vi "Main_Marvin Remake.vi"() -> ()   [LabVIEW 2017]
uses:
  PCAN_Driver/ControlCAN.llb/DevType.ctl
  PCAN_Driver/ControlCAN.llb/CAN Channel.ctl
  PCAN_Driver/ControlCAN.llb/VCI_INIT_CONFIG.ctl
  PCAN_Driver/ControlCAN.llb/InitFlag.ctl
  PCAN_Driver/ControlCAN.llb/Fliter.ctl
  PCAN_Driver/ControlCAN.llb/Mode.ctl
  <vilib>/Utility/miscctls.llb/LVRowAndColumnTypeDef.ctl
  <vilib>/Utility/sysdir.llb/System Directory Type.ctl
  <vilib>/Utility/config.llb/Read Key (String).vi
  <vilib>/Utility/config.llb/Write Key (String).vi
  <vilib>/Utility/cursorutil.llb/Set Cursor (Icon Pict).vi
  PCAN_Driver/ControlCAN.lvlib
  <vilib>/Utility/config.llb/NI_LVConfig.lvlib
panel:
  out "ADCValOutput Single":dbl
  out "Numeric 3":i32
  out "5.4.0":bool=TRUE
  out "MaxEbaySpeed":u16
  out "AuxiONResult 2":bool
  out "AuxiOFFResult 2":bool
  out "Numeric 2":dbl
  out "UUT SoftwareVer2":string
  out "Numeric":dbl
  out "DSP Board S/N":string
  out "POWER Board S/N":string caption="DRIVER Board S/N"
  out "BurnInSpeed":u16
  out "SpeedCommandSpeed":u16
  out "VenableSpeed":u16
  out "CurrentTest":T1(ring)
  out "TesterVersion":string
  out "ClosePanel":bool=TRUE
  out "UUT SN Report":string
  out "Automation":bool
  out "Test Failed":bool
  out "AuxiOFFResult":bool
  out "AuxiONResult":bool
  out "SensCalResult":bool
  out "VisualInspectionResult":bool
  out "BurnResult":bool
  out "BurnSpeed":bool
  out "BurnTemp":bool
  out "BurnDC":bool
  out "TempControlResult":bool
  out "MotorTempResult":bool
  out "StopTimeResult":bool
  out "SpeedResult":bool=TRUE
  out "VenableDirectionResult":bool
  out "VenableResult":bool
  out "ComTestResult":bool=TRUE
  out "UUT SoftwareVer":string
  out "Next SN":i32
  in  "SetSN":bool
  out "Current SN":i32
  out "Cal":dbl
  out "AO[1]Meas":dbl
  out "FullSpeed2 Speed":dbl
  out "FullSpeed2 Current":dbl
  out "FullSpeed1 Current":dbl
  out "FullSpeed1 Speed":dbl
  out "MaxBurnInTempVal":dbl
  in  "Stop Burn-in":bool
  out "VISA Tester":refnum<visa-resource-name>
  out "UUT":u8
  out "CAN Status":bool
  in  "Channel 2":T2 caption="Channel" items=["Channel 1", "Channel 2"]
  out "Config_CANAT":T8 {"DevType" items=["USB-CAN"=3, "USB-CAN2"=4]; "CanIndex" items=["通道1", "通道2"]; "VCI_INIT_CONFIG"."Fliter" items=["接收所有类型"=3, "只接收标准帧"=4, "只接收扩展帧"=7]; "VCI_INIT_CONFIG"."Mode" items=["正常工作", "自测模式（环回）", "仅侦听模式"]; "VCI_INIT_CONFIG"."InitFlag" items=["使用Flash参数", "使用界面设置参数"]}
  out "Array":u64[][](array[numeric]) format="%016x"
  out "Motor Phase Current RMS":dbl
  out "Ambient Temperature":dbl
  out "Speed error":bool
  out "Commutation err":bool
  out "Under voltage/Over voltage":bool
  out "Derated drive temp":bool
  out "Motor Over temperature":bool
  out "Motor Sensor temp Fauilre":bool
  out "Drive Over temperature":bool
  out "Drive Sensor temp Failure":bool
  out "Ambient Over temp":bool
  out "Ambient Sensor temp":bool
  out "DC Voltage":dbl
  out "DC Current":dbl
  out "Power transistor Heat sink Temp.":dbl
  out "Motor Stator Temp.":dbl
  out "Motor Speed RPM":dbl
  out "ECS State":u16
  out "UUT":string="EBAY"
  in  "Logger Path":path
  in  "Report":bool
  in  "Start":bool
  in  "ATR":string[][](table)=[["Test Communication", "-", "-", "-", "-", ""], ["Set S/N", "-", "-", "-", "-", ""], ["Set Board Number", "-", "-", "-", "-", ""], [" ", "", "", "", "", ""], ["Test Communication", "-", "-", "-", "-", ""], ["Get S/N", "-", "-", "-", "", ""], ["Get Board Number", "-", "-", "-", "", ""], ["Get FW", "-", "-", "-", "", ""], ["Enable Motor", "", "", "", "", ""], ["Small position command", "", "", "", "", ""], ["Measure delta", "", "", "", "", ""], ["Velocity command", "", "", "", "", ""]]
  in  "Settings":bool
  in  "Refresh Button":bool
  out "Status":bool
  in  "VISA Marvin":refnum<visa-resource-name>="COM6"
  in  "Serial Com":bool
  in  "Help Button":bool
  out "Pannel User Message":string
  in  "Stop Button":bool
  # "Marvin"
  # "REDLER TECHNOLOGIES LTD"
  # "ver 1.2p"
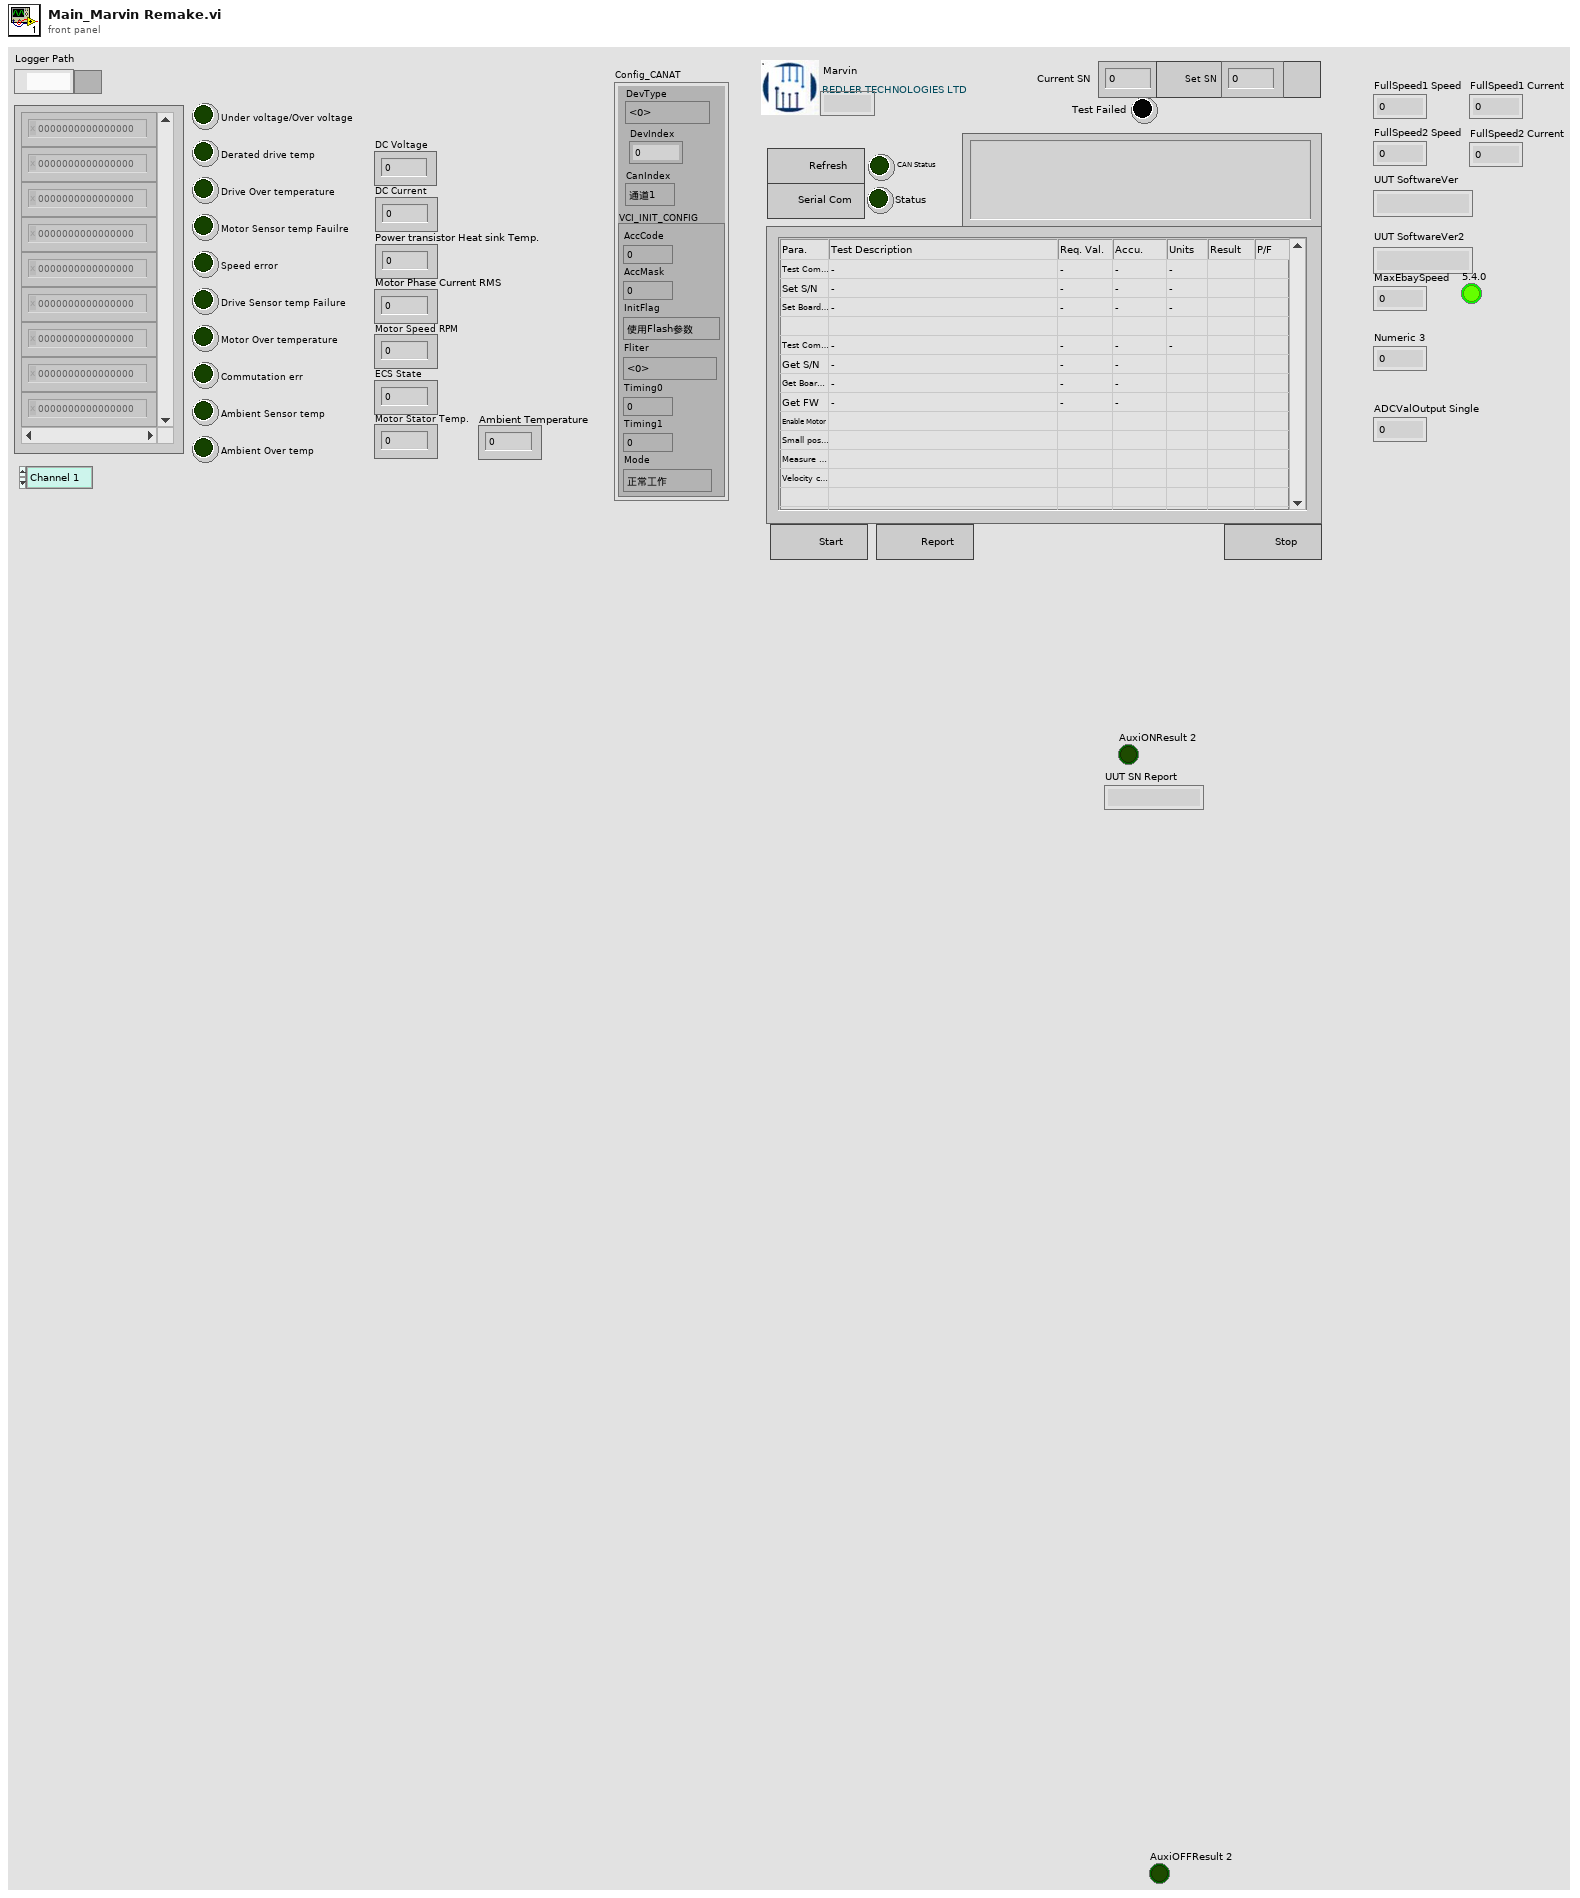
[diagram p1: front panel]
types:
  T1 = enum16{"Auxiliary", "Temp Sens Cal", "Com Test", "Enable Test", "Speed Command", "Stop Time", "Temp Control", "Burn in", "Visual Inspec", "Empty"}
  T2 = typedef "CAN Channel.ctl" = u32
  T3 = typedef "DevType.ctl" = u32
  T4 = typedef "ControlCAN.lvlib/VCI_INIT_CONFIG.ctl" = cluster{"AccCode":u32, "AccMask":u32, "InitFlag":T5, "Fliter":T6, "Timing0":u8, "Timing1":u8, "Mode":T7}
  T5 = typedef "ControlCAN.lvlib/InitFlag.ctl" = u32
  T6 = typedef "ControlCAN.lvlib/Fliter.ctl" = u8
  T7 = typedef "ControlCAN.lvlib/Mode.ctl" = u8
  T8 = cluster{"DevType":T3, "DevIndex":u32, "CanIndex":T2, "VCI_INIT_CONFIG":T4}
  T9 = cluster{"VISA":refnum<visa-resource-name>, "Array Test":enum16{"Auxiliary", "Temp Sens Cal", "Com Test", "Enable Test", "Speed Command", "Stop Time", "Temp Control", "Burn in", "Visual Inspec", "Empty"}[]}
  T10 = cluster{"ID":u32, "MSGTYPE":u8, "LEN":u8, "aDATA":u8[]}[]
  T11 = enum16{"Erase ATR Table", "Stop", "MainProgram", "Initialize"}
  T12 = typedef "NI_LVConfig.lvlib/Config Data RefNum.ctl" = refnum<k1>
  T13 = enum16{"K15", "K16", "K17", "Venable", "Firmeware", "Fan", "Power", "120C", "110C", "100C", "90C", "80C", "70C", "60C", "50C", "40C", "30C", "25C", "20C", "10C", "0C"}
  T14 = enum16{"Stop", "Result", "FullSpeed2", "MD[1]=1", "FullSpeed1", "MD[1]=0"}
  T15 = enum8{"Term1", "Term2", "Current", "Fan", "TempCPU"}
  T16 = enum16{"Stop", "AO[1]=Meas.", "TA[5]", "AO[1]=0", "Start"}
  T17 = enum16{"Stop", "BurnIn", "Ambient Temp", "MotorSpeed", "DC Current Measure", "Start"}
  T18 = enum16{"Auxiliary", "Temp Sens Cal", "Com Test", "Enable Test", "Speed Command", "Stop Time", "Temp Control", "Burn in", "Visual Inspec", "Empty"}[]
  T19 = enum16{"K15", "K16", "K17", "Venable", "Firmeware", "Fan", "Power", "120C", "110C", "100C", "90C", "80C", "70C", "60C", "50C", "40C", "30C", "25C", "20C", "10C", "0C"}[]
  T20 = enum32{"6000", "11500", "15100", "11500-2", "6000-2"}[]
  T21 = enum8{"Enabled", "Disabled", "Disabled and Grayed Out"}
  T22 = typedef "LVRowAndColumnTypeDef.ctl" = cluster{"Row":i32, "Column":i32}
  T23 = enum32{"Invalid", "Standard", "Closed", "Hidden", "Minimized", "Maximized"}
  T24 = cluster{"ID":u32, "MSGTYPE":u8, "LEN":u8, "aDATA":u8[]}
  T25 = enum16{"open", "replace", "create", "open or create", "replace or create", "replace or create with confirmation"}
  T26 = typedef "ControlCAN.lvlib/DevType.ctl" = u32
  T27 = typedef "ControlCAN.lvlib/CAN Channel.ctl" = u32
  T28 = cluster{"DevType":T26, "DevIndex":u32, "CanIndex":T27, "VCI_INIT_CONFIG":T4}
  T29 = typedef "ControlCAN.lvlib/VCI_CAN_OBJ.ctl" = cluster{"ID":u32, "TimeStamp":u32, "TimeFlag":u8, "SendType":u8, "RemoteFlag":u8, "ExternFlag":u8, "DataLen":u8, "Data":u8[], "Reserved":u8[]}
  T30 = cluster{"Type":enum16{"接收", "发送"}, "Channel":T2, "Time":timestamp, "VCI_CAN_OBJ":T29}[]
  T31 = cluster{"Type":enum16{"接收", "发送"}, "Channel":T2, "Time":timestamp, "VCI_CAN_OBJ":T29}
  T32 = typedef "LVPoint32TypeDef.ctl" = cluster{"Horizontal":i32, "Vertical":i32}
  T33 = enum8{"Term1", "Term2", "Current", "Fan", "TempCPU"}[]
  T34 = typedef "System Directory Type.ctl" = i32
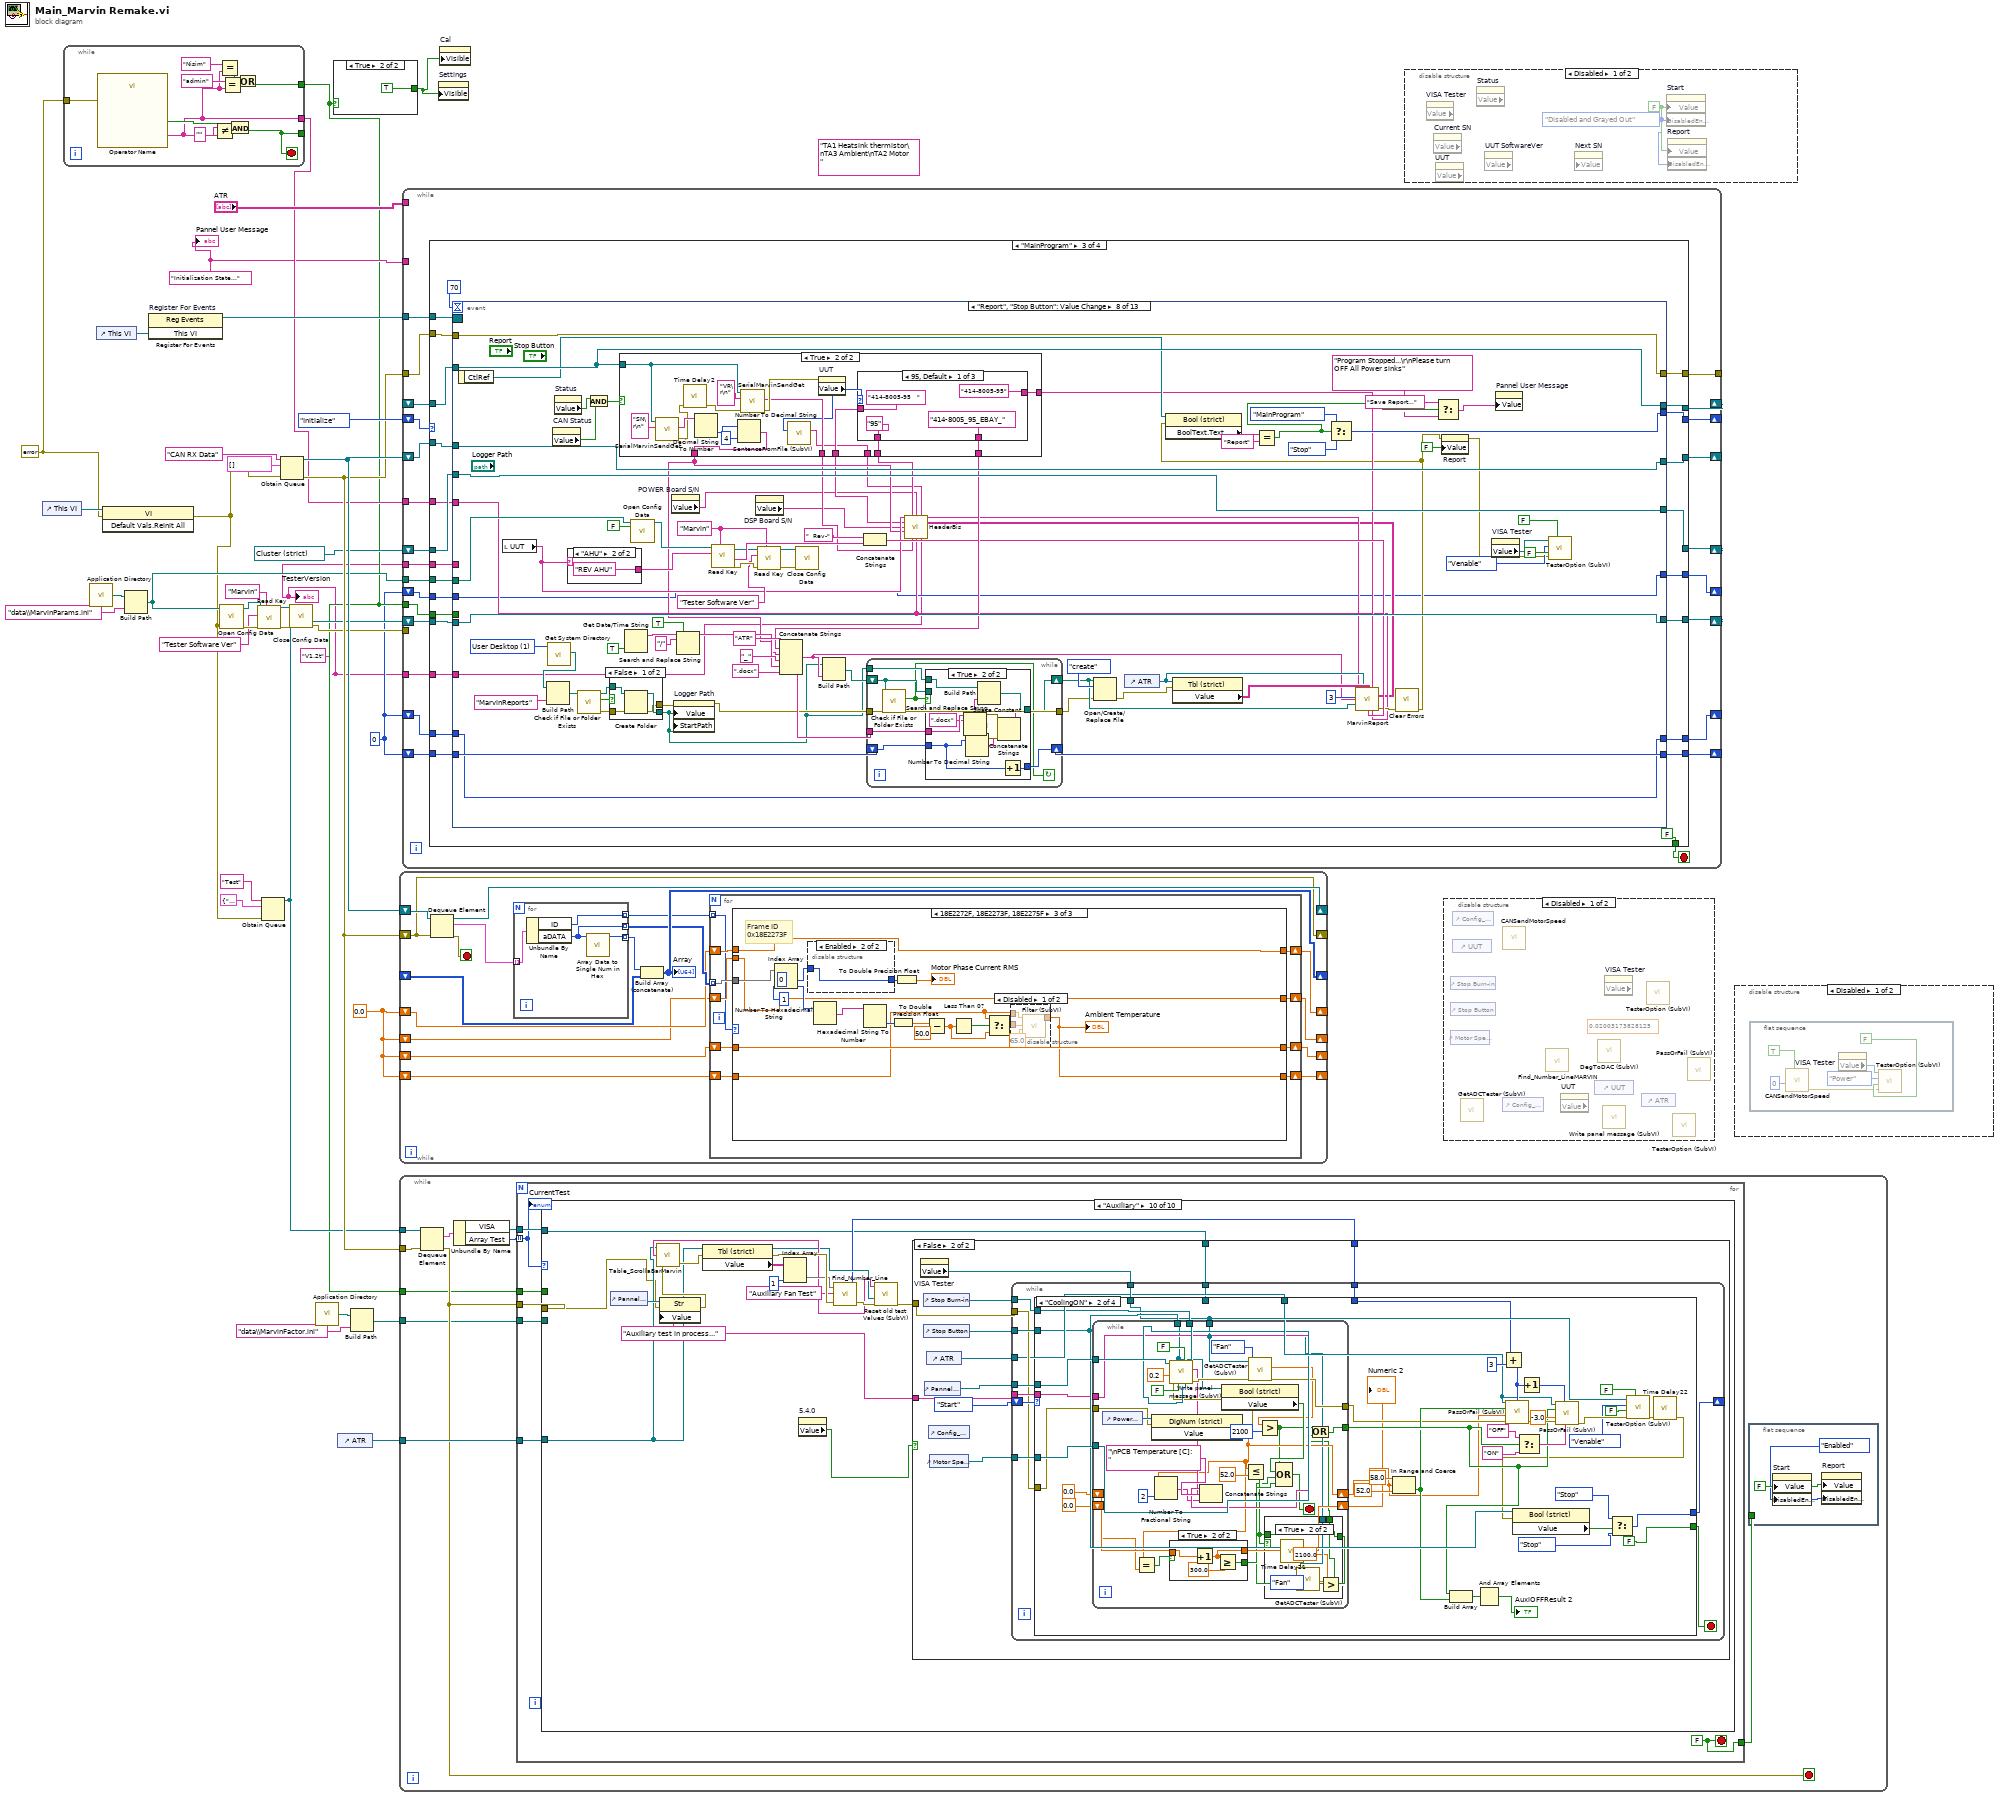
[diagram p0: block diagram]
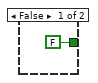
[diagram p2: hidden frame]
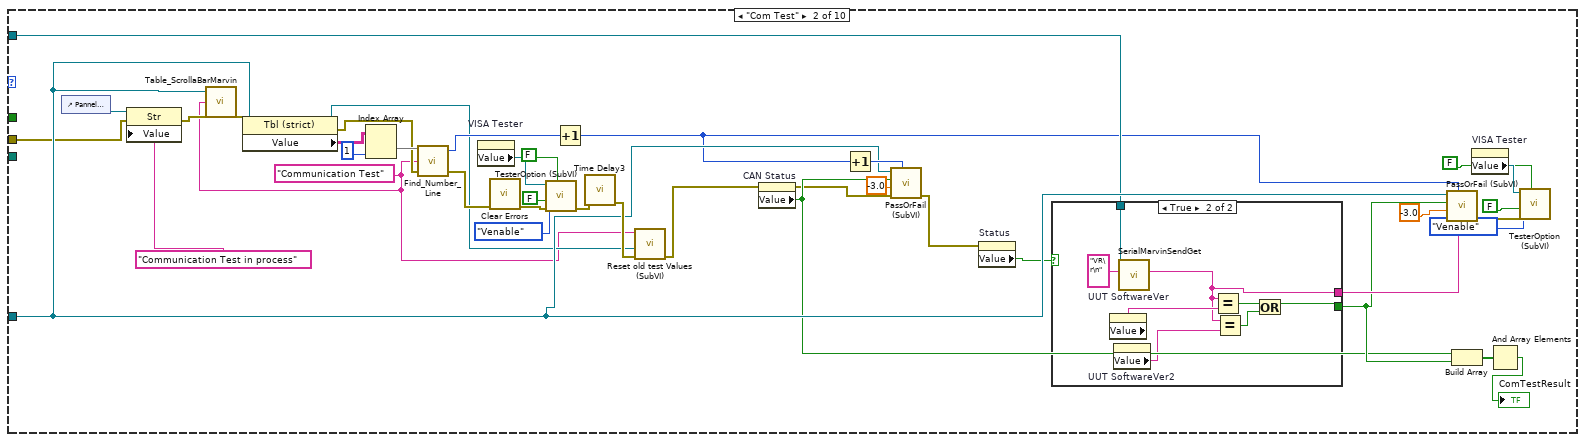
[diagram p7: hidden frame]
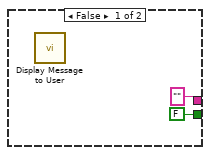
[diagram p8: hidden frame]
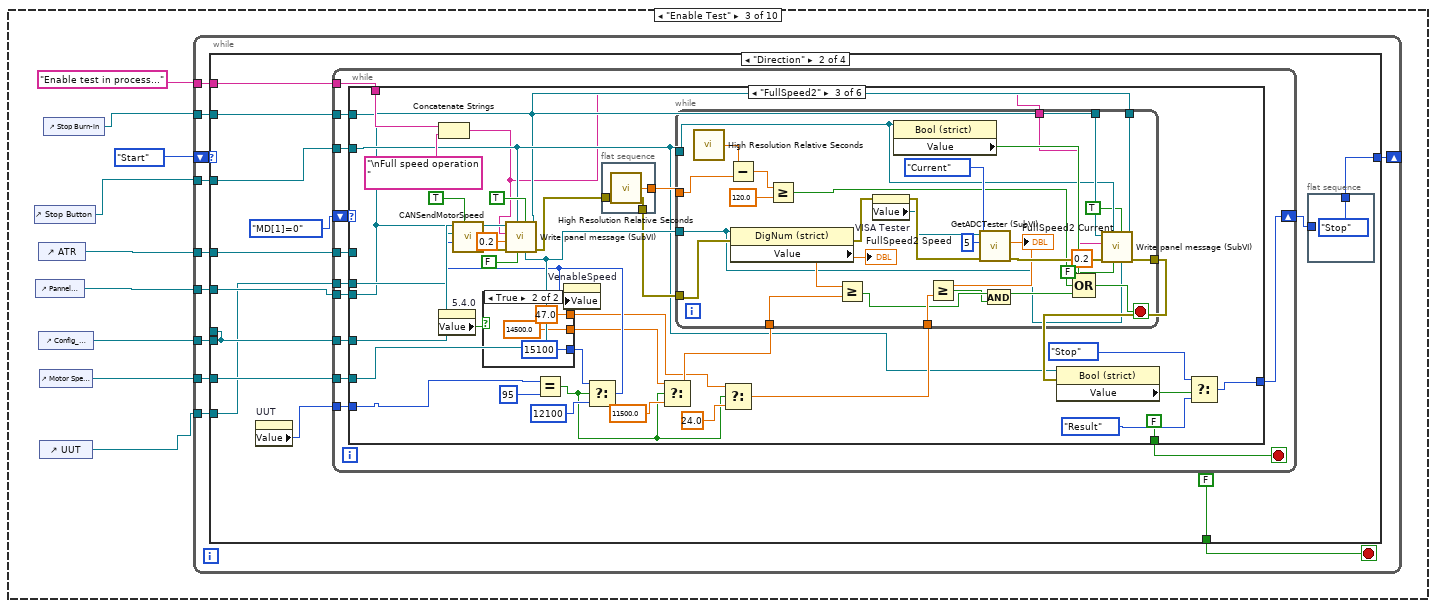
[diagram p9: hidden frame]
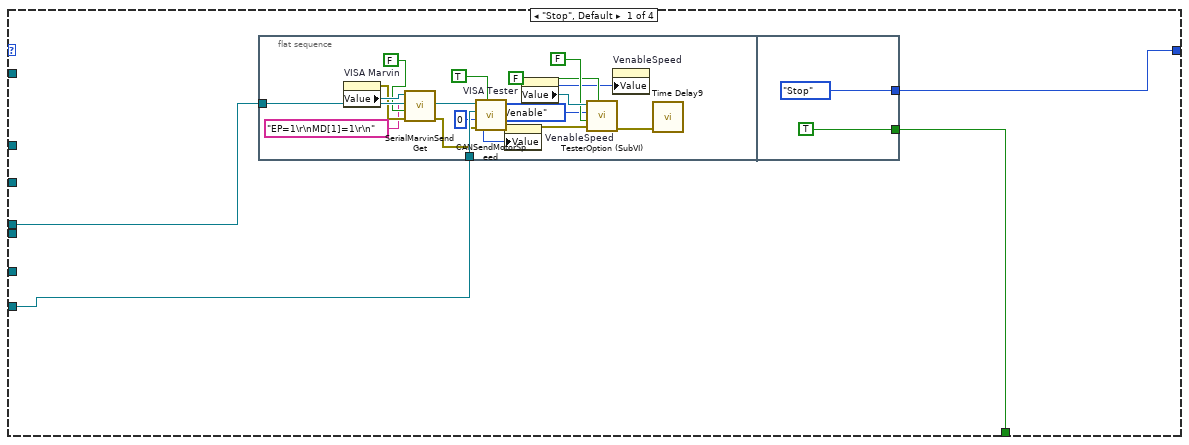
[diagram p10: hidden frame]
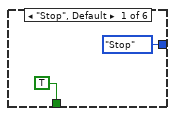
[diagram p11: hidden frame]
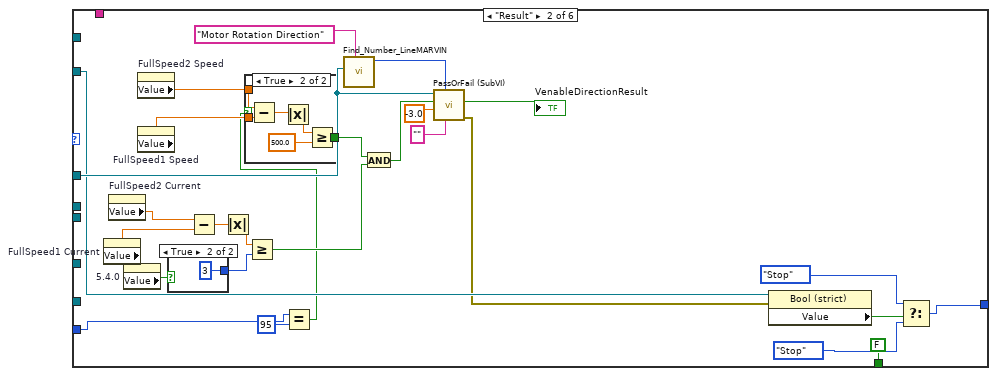
[diagram p12: hidden frame]
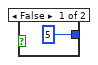
[diagram p13: hidden frame]
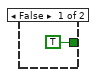
[diagram p14: hidden frame]
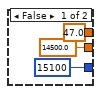
[diagram p15: hidden frame]
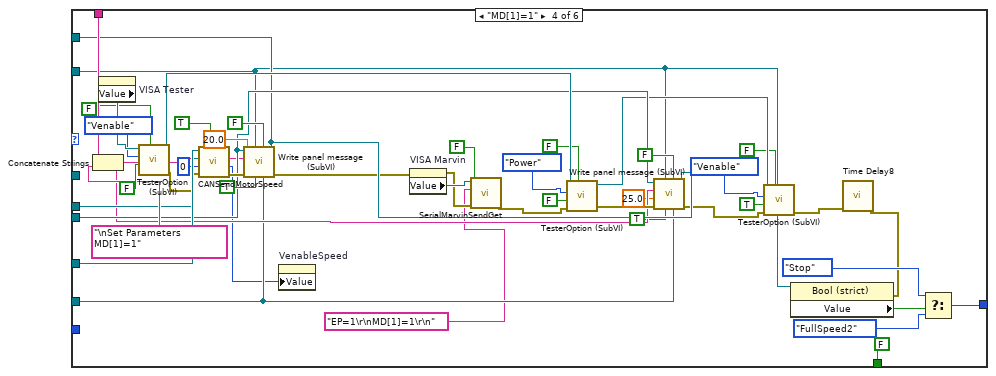
[diagram p16: hidden frame]
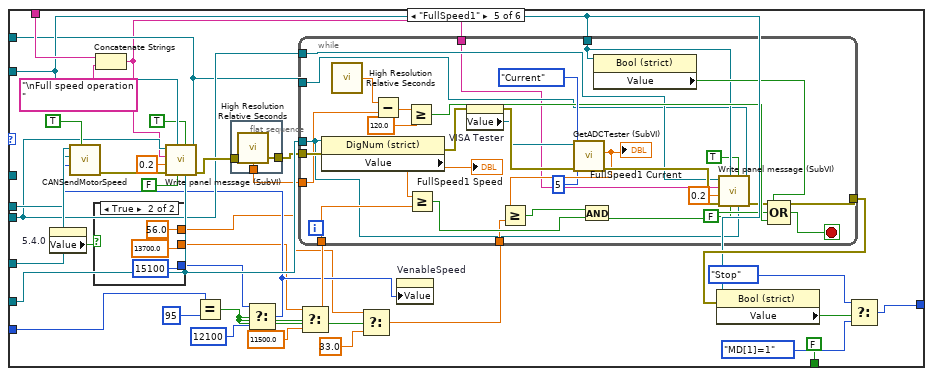
[diagram p17: hidden frame]
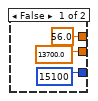
[diagram p18: hidden frame]
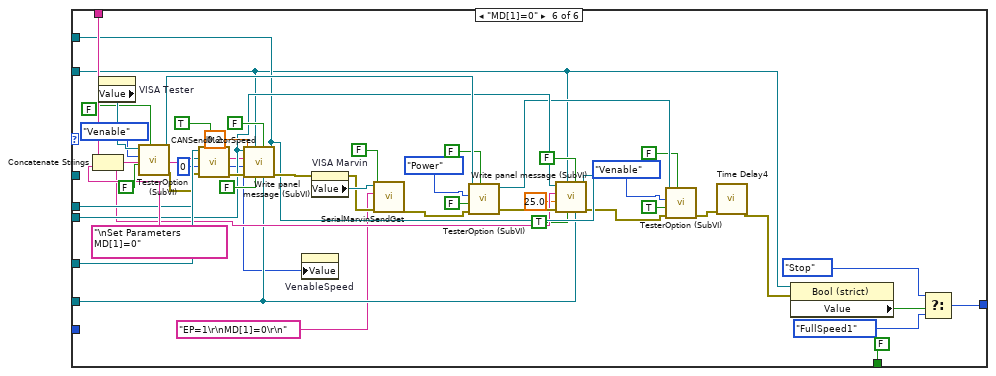
[diagram p19: hidden frame]
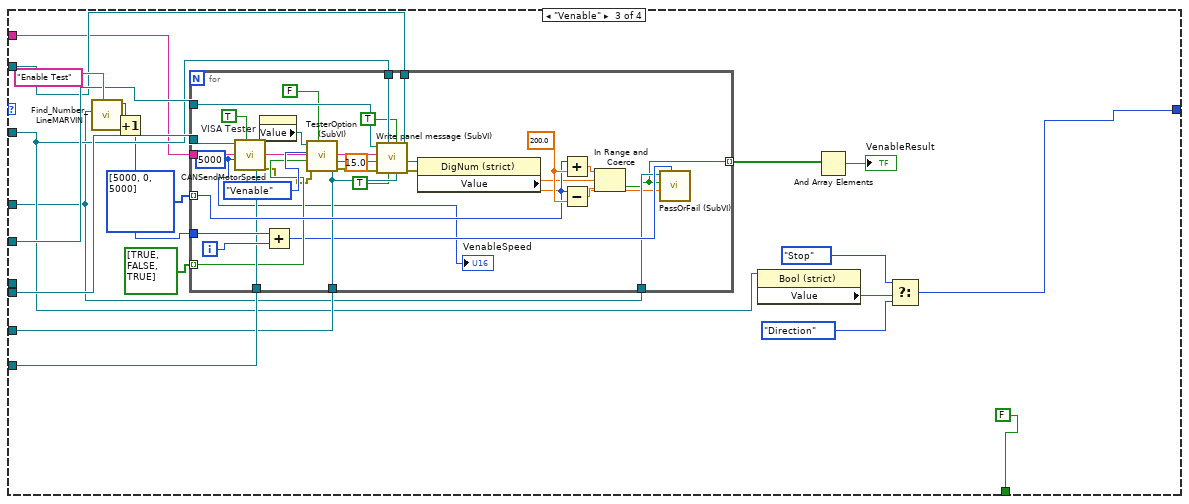
[diagram p20: hidden frame]
diagram:
  w1 = "V1.2t" ("Tester Software Ver")
  (unwired) "TA1 Heatsink thermistor\nTA3 Ambient\nTA2 Motor "
  w19 = "Initialization State..."
  w2 = 0
  w26 = 0.0
  w5 = errorcluster {"status"=FALSE, "code"=0, "source"=""} ("error in (no error)")
  n1 = control-ref of="This VI"() -> (w6:refnum<vi>)
  n2 = while {
    tunnel: [w44] -> _
    tunnel: [w40] -> w21
    tunnel: [w41] -> w3
    tunnel: w5 -> [w37]
    stop <- w44 stop-if-true
    n3 = call "Operator Name"("error in (no error)"=w37) -> ("Operator Name"=w40:string, "OK"=w45:bool)  [unwired: 16 in, 1 out]
    n4 = Not Equal?(x=w40, y="") -> (x != y?=w46:bool)
    n5 = Equal?(x="Nisim", y=w40) -> (x = y?=w38:bool)
    n6 = Equal?(x="admin", y=w40) -> (x = y?=w42:bool)
    n7 = And(x=w45, y=w46) -> (x .and. y?=w44:bool)
    n8 = Or(x=w38, y=w42) -> (x .or. y?=w41:bool)
  }
  n9 = call <vilib>:"Application Directory.vi"() -> ("Application Directory"=w25:path)
  n10 = control-ref of="This VI"() -> (w23:refnum<vi>)
  n11 = invoke class="VI" method="Default Vals.Reinit All"(reference=w6, error in=w5) -> (error out=w4:errorcluster)  [unwired: 1 in, 2 out]
  n12 = Build Path(base path=w25, name or relative path="data\\MarvinParams.ini") -> (appended path=w8:path)
  n13 = register-events "Register For Events"(w23) -> (reference out=w22:refnum<event-registration>)  [unwired: 2 in, 1 out]
  n14 = call <vilib>:"Open Config Data.vi"("error in (no error)"=w4, "configuration file path"=w8) -> ("error out"=w14:errorcluster, "refnum"=w13:T12)  [unwired: 1 in, 7 out]
  n15 = call-poly <vilib>:"Read Key.vi"("section"="Marvin", "error in (no error)"=w14, "key"="Tester Software Ver", "refnum"=w13) -> ("error out"=w11:errorcluster, "refnum out"=w10:T12)  [unwired: 2 in, 4 out]
  n16 = Obtain Queue(name (unnamed)="Test", element data type=T9 {"VISA"="COM1", "Array Test"=[]}, error in (no error)=w4) -> (queue out=w30:refnum<queue>)  [unwired: 2 in, 2 out]
  n17 = Obtain Queue(name (unnamed)="CAN RX Data", element data type=T10 [], error in (no error)=w4) -> (queue out=w33:refnum<queue>, error out=w31:errorcluster)  [unwired: 2 in, 1 out]
  n18 = call <vilib>:"Close Config Data.vi"("error in (no error)"=w11, "refnum"=w10) -> ("error out"=w9:errorcluster)  [unwired: 8 in, 1 out]
  n19 = call <vilib>:"Application Directory.vi"() -> ("Application Directory"=w16:path)
  n20 = case shown="True" w3 {
    tunnel: [FALSE TRUE] -> w20
    frame False {
    }
    frame True {
    }
  }
  n21 = control-ref of="ATR"() -> (w18:refnum<vi>)
  n22 = Build Path(base path=w16, name or relative path="data\\MarvinFactor.ini") -> (appended path=w15:path)
  n23 = while {
    shift-right: [w65] -> _
    shift-left: w33 -> [w67]
    shift-right: [w63] -> _
    shift-left: _ -> [w64]
    shift-right: [w59] -> _
    shift-left: w31 -> [w59]
    shift-right: [w57] -> _
    shift-left: w26 -> [w58]
    shift-right: [w56] -> _
    shift-left: w26 -> [w55]
    shift-right: [w54] -> _
    shift-left: w26 -> [w53]
    shift-right: [w52] -> _
    shift-left: w26 -> [w51]
    stop <- w66 stop-if-true
    n24 = Dequeue Element(queue=w67, error in (no error)=w59) -> (queue out=w65:refnum<queue>, element=w60:T10, error out=w66:errorcluster)  [unwired: 1 in, 1 out]
    n25 = for {
      tunnel: [w213] -> w62 mode=indexing
      tunnel: w60 -> [w212] mode=indexing
      tunnel: [w211] -> w61 mode=indexing
      tunnel: [w210] -> w50 mode=indexing
      n26 = Unbundle By Name(w212) -> ("ID"=w210:u32, "aDATA"=w211:u8[])
      n27 = call "Array Data to Single Num in Hex.vi"("aDATA"=w211) -> ("Numeric"=w213:u64)  [unwired: 10 in]
    }
    n28 = Build Array (concatenate)(w62, w64) -> (w63:u64[][])
    "Array" <- w63
    n29 = for {
      tunnel: w61 -> [w77] mode=indexing
      shift-right: [w75] -> w57
      shift-left: w58 -> [w76]
      shift-right: [w74] -> w56
      shift-left: w55 -> [w73]
      shift-right: [w72] -> w54
      shift-left: w53 -> [w71]
      shift-right: [w70] -> w52
      shift-left: w51 -> [w69]
      tunnel: w50 -> [w68] mode=indexing
      n30 = case shown="18E2272F, 18E2273F, 18E2275F" w68 {
        tunnel: w77 -> [w114 w162 w200]
        tunnel: w76 -> [w88 w151 w189]
        tunnel: [w87 w151 w189] -> w75
        tunnel: [w84 w150 w188] -> w74
        tunnel: w73 -> [w83 w150 w188]
        tunnel: [w80 w149 w187] -> w72
        tunnel: w71 -> [w79 w149 w187]
        tunnel: [w78 w148 w183] -> w70
        tunnel: w69 -> [w78 w148 w182]
        frame 417408815, 417408831, 417408863, Default {
          # "Frame ID\n0x18E1273F"
          n31 = Index Array(array=w114, index #1=0 ("index"), index #2=1 ("index"), index #3=2 ("index"), index #4=3 ("index"), index #5=4 ("index"), index #6=5 ("index"), index #7=6 ("index"), index #8=7 ("index")) -> (element #1=w98:u8, element #2=w100:u8, element #3=w101:u8, element #4=w105:u8, element #5=w108:u8, element #6=w112:u8, element #7=w113:u8, element #8=w111:u8)
          n32 = Number To Hexadecimal String(2:w111) -> (0:w125:string)  [unwired: 1 in]
          n33 = Join Numbers(hi=w113, lo=w112) -> ((hi.lo)=w132:u16)
          n34 = Join Numbers(hi=w101, lo=w100) -> ((hi.lo)=w102:u16)
          n35 = Number To Hexadecimal String(2:w108) -> (0:w109:string)  [unwired: 1 in]
          n36 = Number To Hexadecimal String(2:w132) -> (0:w131:string)  [unwired: 1 in]
          n37 = Number To Hexadecimal String(2:w98) -> (0:w99:string)  [unwired: 1 in]
          n38 = Number To Hexadecimal String(2:w102) -> (0:w103:string)  [unwired: 1 in]
          n39 = Number To Hexadecimal String(2:w105) -> (0:w106:string)  [unwired: 1 in]
          n40 = Hexadecimal String To Number(string=w125) -> (number=w124:u32)  [unwired: 2 in, 1 out]
          n41 = To Double Precision Float(number=w124) -> (double precision float=→"DC Current":dbl)
          n42 = Hexadecimal String To Number(string=w109) -> (number=w110:u32)  [unwired: 2 in, 1 out]
          n43 = Hexadecimal String To Number(string=w131) -> (number=w130:u32)  [unwired: 2 in, 1 out]
          n44 = Hexadecimal String To Number(string=w99) -> (number=w96:u32)  [unwired: 2 in, 1 out]
          n45 = Hexadecimal String To Number(string=w103) -> (number=w104:u32)  [unwired: 2 in, 1 out]
          n46 = Hexadecimal String To Number(string=w106) -> (number=w107:u32)  [unwired: 2 in, 1 out]
          n47 = To Double Precision Float(number=u32 10 ("y")) -> (double precision float=w128:dbl)
          n48 = To Double Precision Float(number=w130) -> (double precision float=w127:dbl)
          n49 = To Double Precision Float(number=w110) -> (double precision float=w93:dbl)
          n50 = To Double Precision Float(number=w104) -> (double precision float=w89:dbl)
          n51 = To Double Precision Float(number=w107) -> (double precision float=w95:dbl)
          n52 = Divide(x=w127, y=w128) -> (x/y=→"DC Voltage":dbl)
          n53 = To Unsigned Word Integer(number=w96) -> (unsigned 16bit integer=→"ECS State":u16)
          n54 = disable-structure shown="Enabled" {
            disable-tunnel: w89 -> [w146 w147]
            disable-tunnel: w88 -> [w145 _]
            disable-tunnel: [w143 w147] -> w87
            frame Disabled {
              n55 = call "Filter (SubVI).vi"("Delta"=5000.0, "NewVal"=w146, "OldVal"=w145) -> ("Val"=w143:dbl)  [unwired: 8 in]
            }
            frame Enabled {
            }
          }
          "Motor Speed RPM" <- w87
          n56 = Subtract(x=w93, y=50.0 ("x")) -> (x-y=w82:dbl)
          n57 = Subtract(x=w95, y=50.0 ("x")) -> (x-y=w85:dbl)
          n58 = Less Than 0?(x=w85) -> (x < 0?=w91:bool)
          n59 = Less Than 0?(x=w82) -> (x < 0?=w90:bool)
          n60 = Select(t=w83, s=w91, f=w85) -> (s? t:f=w86:dbl)
          n61 = Select(t=w79, s=w90, f=w82) -> (s? t:f=w81:dbl)
          n62 = disable-structure shown="Enabled" {
            disable-tunnel: w86 -> [w141 w142]
            disable-tunnel: [w140 w142] -> w84
            disable-tunnel: w83 -> [w139 _]
            frame Disabled {
              n63 = call "Filter (SubVI).vi"("Delta"=130.0, "NewVal"=w141, "OldVal"=w139) -> ("Val"=w140:dbl)  [unwired: 8 in]
            }
            frame Enabled {
            }
          }
          "Motor Stator Temp." <- w84
          n64 = disable-structure shown="Enabled" {
            disable-tunnel: w81 -> [w136 w137]
            disable-tunnel: [w134 w137] -> w80
            disable-tunnel: w79 -> [w133 _]
            frame Disabled {
              n65 = call "Filter (SubVI).vi"("Delta"=100.0, "NewVal"=w136, "OldVal"=w133) -> ("Val"=w134:dbl)  [unwired: 8 in]
            }
            frame Enabled {
            }
          }
          "Power transistor Heat sink Temp." <- w80
        }
        frame 417539887, 417539903, 417539935 {
          # "Framde ID\n0x18E3273F"
          n66 = control-ref of="UUT"() -> (w152:refnum<vi>)
          n67 = property on="Property Node" class="DigNum (strict)"(reference=w152) -> ("Value"=w153:u8)  [unwired: 1 in, 2 out]
          n68 = Index Array(array=w162, index #1=0 ("index"), index #2=1 ("index")) -> (element #1=w160:u8, element #2=w155:u8)
          n69 = Number To Boolean Array(number=w160) -> (Boolean array=w159:bool[])
          n70 = Number To Boolean Array(number=w155) -> (Boolean array=w157:bool[])
          n71 = Boolean To (0,1)(Boolean=w157) -> (0, 1=w154:i16[])
          n72 = Boolean To (0,1)(Boolean=w159) -> (0, 1=w158:i16[])
          n73 = case shown="95" w153 {
            tunnel: w154 -> [_ w163]
            frame 0, Default {
            }
            frame 95 {
              n74 = for {
                tunnel: w163 -> [w168] mode=indexing
                i -> [w164]
                stop <- w166 stop-if-true
                n75 = Not Equal To 0?(x=w168) -> (x != 0?=w167:bool)
                n76 = case shown="0, Default" w164 {
                  tunnel: w167 -> [w169 w170]
                  frame 0, Default {
                    "Ambient Sensor temp" <- w169
                  }
                  frame 1 {
                    "Ambient Over temp" <- w170
                  }
                }
                n77 = Equal?(x=w164, y=1.0) -> (x = y?=w166:bool)
              }
            }
          }
          n78 = for {
            tunnel: w158 -> [w172] mode=indexing
            i -> [w173]
            n79 = Not Equal To 0?(x=w172) -> (x != 0?=w171:bool)
            n80 = case shown="1" w173 {
              tunnel: w171 -> [w174 w175 w176 w177 w178 w179 w180 w181]
              frame 0, Default {
                "Drive Sensor temp Failure" <- w174
              }
              frame 1 {
                "Drive Over temperature" <- w175
              }
              frame 2 {
                "Motor Sensor temp Fauilre" <- w176
              }
              frame 3 {
                "Motor Over temperature" <- w177
              }
              frame 4 {
                "Derated drive temp" <- w178
              }
              frame 5 {
                "Under voltage/Over voltage" <- w179
              }
              frame 6 {
                "Commutation err" <- w180
              }
              frame 7 {
                "Speed error" <- w181
              }
            }
          }
        }
        frame 417474351, 417474367, 417474399 {
          # "Frame ID\n0x18E2273F"
          n81 = Index Array(array=w200, index #1=0 ("index"), index #2=1 ("index")) -> (element #1=w197:u8, element #2=w194:u8)
          n82 = disable-structure shown="Enabled" {
            disable-tunnel: [w208 w209] -> w198
            disable-tunnel: w197 -> [w207 w209]
            frame Disabled {
              n83 = Number To Hexadecimal String(2:w207) -> (0:w206:string)  [unwired: 1 in]
              n84 = Hexadecimal String To Number(string=w206) -> (number=w208:u32)  [unwired: 2 in, 1 out]
            }
            frame Enabled {
            }
          }
          n85 = Number To Hexadecimal String(2:w194) -> (0:w192:string)  [unwired: 1 in]
          n86 = Hexadecimal String To Number(string=w192) -> (number=w193:u32)  [unwired: 2 in, 1 out]
          n87 = To Double Precision Float(number=w193) -> (double precision float=w191:dbl)
          n88 = To Double Precision Float(number=w198) -> (double precision float=→"Motor Phase Current RMS":dbl)
          n89 = Subtract(x=w191, y=50.0) -> (x-y=w185:dbl)
          n90 = Less Than 0?(x=w185) -> (x < 0?=w186:bool)
          n91 = Select(t=w182, s=w186, f=w185) -> (s? t:f=w184:dbl)
          n92 = disable-structure shown="Disabled" {
            disable-tunnel: w184 -> [w204 w205]
            disable-tunnel: [w202 w205] -> w183
            disable-tunnel: w182 -> [w201 _]
            frame Disabled {
              n93 = call "Filter (SubVI).vi"("Delta"=65.0, "NewVal"=w204, "OldVal"=w201) -> ("Val"=w202:dbl)  [unwired: 8 in]
            }
            frame Enabled {
            }
          }
          "Ambient Temperature" <- w183
        }
      }
    }
  }
  n94 = while {
    tunnel: w18 -> [w223]
    tunnel: w31 -> [w221]
    tunnel: w30 -> [w222]
    tunnel: w15 -> [w215]
    tunnel: w3 -> [w214]
    stop <- w217 stop-if-true
    n95 = Dequeue Element(queue=w222, error in (no error)=w221) -> (element=w220:T9, error out=w217:errorcluster)  [unwired: 1 in, 2 out]
    n96 = Unbundle By Name(w220) -> ("VISA"=w219:refnum<visa-resource-name>, "Array Test"=w218:T18)
    n97 = for {
      tunnel: w218 -> [w229] mode=indexing
      tunnel: w219 -> [w232]
      tunnel: w223 -> [w231]
      tunnel: w217 -> [w230]
      tunnel: [w228] -> w216
      tunnel: w215 -> [w227]
      tunnel: w214 -> [w226]
      stop <- w228 stop-if-true
      w228 = FALSE
      n98 = case shown="\"Auxiliary\"" w229 {
        tunnel: w232 -> [_ w257 _ _ w871 _ _ _ w1512 w1720]
        tunnel: w231 -> [_ w264 _ w703 w867 w1044 _ w1472 w1519 w1726]
        tunnel: w230 -> [_ w261 _ w718 w877 w1026 _ w1470 w1517 w1725]
        tunnel: w227 -> [_ _ _ _ _ w1028 _ _ _ _]
        tunnel: w226 -> [_ _ _ _ _ _ w1218 _ _ _]
        frame "Empty", Default {
        }
        frame "Com Test" {
          w240 = "Communication Test" ("Test Paragraph")
          n99 = control-ref of="Pannel User Message"() -> (w262:refnum<vi>)
          n100 = property class="Str"(reference=w262, error in=w261, "Value"="Communication Test in process") -> (error out=w260:errorcluster)  [unwired: 1 out]
          n101 = call "Table_ScrollaBarMarvin.vi"("error in"=w260, "Line to focus"=w240, "reference in"=w264) -> ("error out"=w263:errorcluster)  [unwired: 2 out]
          n102 = property class="Tbl (strict)"(reference=w264, error in=w263) -> (reference out=w241:refnum<vi>, error out=w270:errorcluster, "Value"=w271:string[][])
          n103 = Index Array(array=w271, index (col)=1 ("disabled index (col)")) -> (element=w272:string[])  [unwired: 1 in]
          n104 = call "Find_Number_Line.vi"("error in"=w270, "Test Paragraph"=w240, "Row Headers[]"=w272) -> ("error out"=w268:errorcluster, "Line number"=w267:i32)  [unwired: 1 out]
          n105 = property on="VISA Tester" class="VISAName"() -> ("Value"=w251:refnum<visa-resource-name>)  [unwired: 2 in, 2 out]
          n106 = call <vilib>:"Clear Errors.vi"("error in (no error)"=w268) -> ("error out"=w253:errorcluster)  [unwired: 5 in, 1 out]
          n107 = call "TesterOption (SubVI).vi"("2 Options"=FALSE, "error in (no error)"=w253, "On/Off"=FALSE, "Tester Option"=T13."Venable", "VISA Refnum in"=w251) -> ("error out"=w252:errorcluster)  [unwired: 5 in, 1 out]
          n108 = Increment(x=w267) -> (x+1=w233:i32)
          n109 = call "Time Delay3"("error in (no error)"=w252) -> ("error out"=w265:errorcluster)  [unwired: 10 in]
          n110 = call "Reset old test Values (SubVI).vi"("error in"=w265, "Atr in"=w241, "Test Paragraph"=w240) -> ("error out"=w235:errorcluster)  [unwired: 8 in]
          n111 = property on="CAN Status" class="Bool (strict)"(error in=w235) -> (error out=w234:errorcluster, "Value"=w236:bool)  [unwired: 1 in, 1 out]
          n112 = Increment(x=w233) -> (x+1=w266:i32)
          n113 = call "PassOrFail (SubVI).vi"("index (row)"=w266, "error in (no error)"=w234, "Data in"=-3.0, "Pass?Fail"=w236, "Table in"=w264) -> ("error out"=w256:errorcluster)  [unwired: 6 in]
          n114 = property on="Status" class="Bool (strict)"(error in=w256) -> ("Value"=w258:bool)  [unwired: 1 in, 2 out]
          n115 = case shown="True" w258 {
            tunnel: w257 -> [_ w282]
            tunnel: [FALSE w278] -> w238
            tunnel: ["" ("read buffer") w276] -> w255
            frame False {
              n116 = call "Display Message to User"() -> ()  [unwired: 10 in, 2 out]
            }
            frame True {
              n117 = property on="UUT SoftwareVer" class="Str"() -> ("Value"=w280:string)  [unwired: 2 in, 2 out]
              n118 = property on="UUT SoftwareVer2" class="Str"() -> ("Value"=w275:string)  [unwired: 2 in, 2 out]
              n119 = call "SerialMarvinSendGet.vi"("write buffer"="VR\r\n", "VISA resource name"=w282) -> ("read buffer"=w276:string)  [unwired: 8 in, 1 out]
              n120 = Equal?(x=w276, y=w280) -> (x = y?=w279:bool)
              n121 = Equal?(x=w276, y=w275) -> (x = y?=w277:bool)
              n122 = Or(x=w279, y=w277) -> (x .or. y?=w278:bool)
            }
          }
          n123 = call "PassOrFail (SubVI).vi"("String Res"=w255, "index (row)"=w233, "Data in"=-3.0, "Pass?Fail"=w238, "Table in"=w264) -> ("error out"=w247:errorcluster)  [unwired: 6 in]
          n124 = Build Array(w236, w238) -> (w239:bool[])
          n125 = property on="VISA Tester" class="VISAName"() -> ("Value"=w246:refnum<visa-resource-name>)  [unwired: 2 in, 2 out]
          n126 = And Array Elements(Boolean array=w239) -> (logical AND=→"ComTestResult":bool)
          n127 = call "TesterOption (SubVI).vi"("2 Options"=FALSE, "error in (no error)"=w247, "On/Off"=FALSE, "Tester Option"=T13."Venable", "VISA Refnum in"=w246) -> ()  [unwired: 5 in, 2 out]
        }
        frame "Enable Test" {
          n128 = control-ref of="Stop Button"() -> (w285:refnum<vi>)
          n129 = control-ref of="Pannel User Message"() -> (w287:refnum<vi>)
          n130 = control-ref of="ATR"() -> (w286:refnum<vi>)
          n131 = control-ref of="Config_CANAT"() -> (w288:refnum<vi>)
          n132 = control-ref of="Motor Speed RPM"() -> (w289:refnum<vi>)
          n133 = control-ref of="UUT"() -> (w290:refnum<vi>)
          n134 = control-ref of="Stop Burn-in"() -> (w291:refnum<vi>)
          n135 = while {
            shift-right: [w296] -> _
            shift-left: enum16{"Stop", "Direction", "Venable", "Start"}."Start" -> [w302]
            tunnel: w285 -> [w301]
            tunnel: w286 -> [w300]
            tunnel: w287 -> [w299]
            tunnel: w288 -> [w292]
            tunnel: w289 -> [w298]
            tunnel: w290 -> [w293]
            tunnel: w291 -> [w295]
            tunnel: "Enable test in process..." ("Strin") -> [w294]
            stop <- w297 stop-if-true
            n136 = case shown="\"Direction\"" w302 {
              tunnel: w301 -> [_ w334 w633 w680]
              tunnel: w300 -> [_ w329 w631 w687]
              tunnel: w299 -> [_ w332 w635 w686]
              tunnel: w292 -> [_ w335 w638 _]
              tunnel: w298 -> [_ w331 w636 w678]
              tunnel: w293 -> [w303 w325 w637 _]
              tunnel: [w306 FALSE FALSE FALSE] -> w297
              tunnel: [w304 w328 w632 w684] -> w296
              tunnel: w295 -> [_ w333 w634 w679]
              tunnel: w294 -> [_ w330 w630 w677]
              tunnel: w292 -> [w305 _ _ _]
              frame "Stop", Default {
                n137 = flat-sequence {
                  tunnel: w303 -> [w318]
                  tunnel: w305 -> [w317]
                  tunnel: [TRUE] -> w306
                  tunnel: [enum16{"Stop", "Direction", "Venable", "Start"}."Stop"] -> w304
                  frame #0 {
                    w307 = u16 0 ("Motor Speed RPM")
                    n138 = property on="VISA Marvin" class="VISAName"() -> (error out=w311:errorcluster, "Value"=w312:refnum<visa-resource-name>)  [unwired: 2 in, 1 out]
                    n139 = call "SerialMarvinSendGet.vi"("error in (no error)"=w311, "Clear Log"=FALSE, "write buffer"="EP=1\r\nMD[1]=1\r\n", "VISA resource name"=w312) -> ("error out"=w308:errorcluster)  [unwired: 6 in, 1 out]
                    n140 = call "CANSendMotorSpeed.vi"("Remote"=TRUE, "error in (no error)"=w308, "Motor Speed RPM"=w307, "UUT"=w318, "CAN Cluster in"=w317) -> ("error out"=w320:errorcluster)  [unwired: 6 in]
                    n141 = property on="VenableSpeed" class="DigNum (strict)"("Value"=w307) -> ()  [unwired: 2 in, 2 out]
                    n142 = property on="VISA Tester" class="VISAName"() -> ("Value"=w321:refnum<visa-resource-name>)  [unwired: 2 in, 2 out]
                    n143 = call "TesterOption (SubVI).vi"("2 Options"=FALSE, "error in (no error)"=w320, "On/Off"=FALSE, "Tester Option"=T13."Venable", "VISA Refnum in"=w321) -> ("error out"=w313:errorcluster)  [unwired: 5 in, 1 out]
                    n144 = property on="VenableSpeed" class="DigNum (strict)"("Value"=w307) -> ()  [unwired: 2 in, 2 out]
                    n145 = call "Time Delay9"("error in (no error)"=w313) -> ()  [unwired: 10 in, 1 out]
                  }
                  frame #1 {
                  }
                }
              }
              frame "Direction" {
                n146 = property on="UUT" class="DigNum (strict)"() -> ("Value"=w324:u8)  [unwired: 2 in, 2 out]
                n147 = while {
                  shift-right: [w348] -> w327
                  shift-left: T14."MD[1]=0" -> [w349]
                  tunnel: w335 -> [w346]
                  tunnel: w325 -> [w345]
                  tunnel: w334 -> [w344]
                  tunnel: w333 -> [w343]
                  tunnel: w332 -> [w342]
                  tunnel: w331 -> [w341]
                  tunnel: w330 -> [w340]
                  tunnel: w329 -> [w339]
                  tunnel: w324 -> [w338]
                  stop <- w347 stop-if-true
                  n148 = case shown="\"FullSpeed2\"" w349 {
                    tunnel: [T14."Stop" w374 w419 w505 w539 w625] -> w348
                    tunnel: [TRUE FALSE FALSE FALSE FALSE FALSE] -> w347
                    tunnel: w346 -> [_ _ w417 w499 w537 w619]
                    tunnel: w345 -> [_ _ w414 w479 w534 w598]
                    tunnel: w344 -> [_ w362 w396 w470 w519 w588]
                    tunnel: w343 -> [_ _ w394 w480 w517 w599]
                    tunnel: w342 -> [_ _ w395 w481 w518 w600]
                    tunnel: w341 -> [_ _ w410 w468 w531 w594]
                    tunnel: w340 -> [_ _ w405 w489 w529 w608]
                    tunnel: w339 -> [_ w366 _ _ _ _]
                    tunnel: w338 -> [_ w354 w392 _ w512 _]
                    frame "Stop", Default {
                    }
                    frame "Result" {
                      n149 = property on="FullSpeed1 Current" class="DigNum (strict)"() -> ("Value"=w369:dbl)  [unwired: 2 in, 2 out]
                      n150 = property on="FullSpeed2 Current" class="DigNum (strict)"() -> ("Value"=w370:dbl)  [unwired: 2 in, 2 out]
                      n151 = property on="5.4.0" class="Bool (strict)"() -> ("Value"=w352:bool)  [unwired: 2 in, 2 out]
                      n152 = property on="FullSpeed2 Speed" class="DigNum (strict)"() -> ("Value"=w372:dbl)  [unwired: 2 in, 2 out]
                      n153 = property on="FullSpeed1 Speed" class="DigNum (strict)"() -> ("Value"=w371:dbl)  [unwired: 2 in, 2 out]
                      n154 = case shown="True" w352 {
                        tunnel: [u32 5 ("y") u32 3 ("y")] -> w353
                        frame False {
                        }
                        frame True {
                        }
                      }
                      n155 = Subtract(x=w370, y=w369) -> (x-y=w368:dbl)
                      n156 = Absolute Value(x=w368) -> (abs(x)=w358:dbl)
                      n157 = Greater Or Equal?(x=w358, y=w353) -> (x >= y?=w364:bool)
                      n158 = Equal?(x=w354, y=u8 95) -> (x = y?=w356:bool)
                      n159 = case shown="True" w356 {
                        tunnel: w372 -> [_ w385]
                        tunnel: w371 -> [_ w384]
                        tunnel: [TRUE w381] -> w365
                        frame False {
                        }
                        frame True {
                          n160 = Subtract(x=w385, y=w384) -> (x-y=w386:dbl)
                          n161 = Absolute Value(x=w386) -> (abs(x)=w383:dbl)
                          n162 = Greater Or Equal?(x=w383, y=500.0) -> (x >= y?=w381:bool)
                        }
                      }
                      n163 = call "Find_Number_LineMARVIN.vi"("Test Paragraph"="Motor Rotation Direction", "TableIn"=w366) -> ("Line number"=w363:i32)  [unwired: 3 in, 3 out]
                      n164 = And(x=w365, y=w364) -> (x .and. y?=w355:bool)
                      "VenableDirectionResult" <- w355
                      n165 = call "PassOrFail (SubVI).vi"("String Res"="", "index (row)"=w363, "Data in"=-3.0, "Pass?Fail"=w355, "Table in"=w366) -> ("error out"=w361:errorcluster)  [unwired: 6 in]
                      n166 = property class="Bool (strict)"(reference=w362, error in=w361) -> ("Value"=w377:bool)  [unwired: 2 out]
                      n167 = Select(t=T14."Stop", s=w377, f=T14."Stop") -> (s? t:f=w374:T14)
                    }
                    frame "FullSpeed2" {
                      n168 = Concatenate Strings(w405, "\nFull speed operation " ("string")) -> (w393:string)
                      n169 = property on="5.4.0" class="Bool (strict)"() -> ("Value"=w390:bool)  [unwired: 2 in, 2 out]
                      n170 = case shown="True" w390 {
                        tunnel: [u16 15100 ("t") u16 15100 ("t")] -> w389
                        tunnel: [14500.0 ("t") 14500.0 ("t")] -> w388
                        tunnel: [47.0 ("t") 47.0 ("t")] -> w387
                        frame False {
                        }
                        frame True {
                        }
                      }
                      n171 = Equal?(x=w392, y=u8 95) -> (x = y?=w402:bool)
                      n172 = Select(t=w389, s=w402, f=u16 12100 ("y")) -> (s? t:f=w391:u16)
                      n173 = call "CANSendMotorSpeed.vi"("Remote"=TRUE, "Motor Speed RPM"=w391, "UUT"=w414, "CAN Cluster in"=w417) -> ("error out"=w412:errorcluster)  [unwired: 7 in]
                      n174 = call "Write panel message (SubVI).vi"("Stop BurnIn"=w394, 4:"rpm"=w410, 5:"rpm"=TRUE ("rpm"), "PrintTime"=FALSE, "Stop"=w396, "error in (no error)"=w412, "Time to wait"=0.2, "Strin"=w393, "String in"=w395) -> ("error out"=w399:errorcluster)  [unwired: 2 in]
                      n175 = property on="VenableSpeed" class="DigNum (strict)"("Value"=w391) -> ()  [unwired: 2 in, 2 out]
                      n176 = flat-sequence {
                        tunnel: w399 -> [w430]
                        tunnel: [w430] -> w398
                        tunnel: [w429] -> w397
                        frame #0 {
                          n177 = call <vilib>:"High Resolution Relative Seconds.vi"() -> ("relative seconds"=w429:dbl)
                        }
                      }
                      n178 = Select(t=w388, s=w402, f=11500.0) -> (s? t:f=w401:dbl)
                      n179 = Select(t=w387, s=w402, f=24.0) -> (s? t:f=w400:dbl)
                      n180 = while {
                        tunnel: w410 -> [w432]
                        tunnel: w398 -> [w460]
                        tunnel: [w440] -> w407
                        tunnel: w401 -> [w453]
                        tunnel: w400 -> [w452]
                        tunnel: w397 -> [w448]
                        tunnel: w396 -> [w438]
                        tunnel: w395 -> [w439]
                        tunnel: w394 -> [w436]
                        tunnel: w393 -> [w435]
                        stop <- w450 stop-if-true
                        n181 = call <vilib>:"High Resolution Relative Seconds.vi"() -> ("relative seconds"=w449:dbl)
                        n182 = Subtract(x=w449, y=w448) -> (x-y=w447:dbl)
                        n183 = property class="DigNum (strict)"(reference=w432, error in=w460) -> (error out=w459:errorcluster, "Value"=w454:dbl)  [unwired: 1 out]
                        "FullSpeed2 Speed" <- w454
                        n184 = Greater Or Equal?(x=w447, y=120.0) -> (x >= y?=w445:bool)
                        n185 = Greater Or Equal?(x=w454, y=w453) -> (x >= y?=w444:bool)
                        n186 = property on="VISA Tester" class="VISAName"(error in=w459) -> (error out=w458:errorcluster, "Value"=w457:refnum<visa-resource-name>)  [unwired: 1 in, 1 out]
                        n187 = property class="Bool (strict)"(reference=w438) -> ("Value"=w443:bool)  [unwired: 1 in, 2 out]
                        n188 = call "GetADCTester (SubVI).vi"("error in (no error)"=w458, "GetADCTester"=T15."Current", "TimeToGet"=5, "VISA Refnum in"=w457) -> ("error out"=w455:errorcluster, "ADCValOutput Single"=w451:dbl)  [unwired: 5 in, 1 out]
                        "FullSpeed2 Current" <- w451
                        n189 = Greater Or Equal?(x=w451, y=w452) -> (x >= y?=w441:bool)
                        n190 = And(x=w444, y=w441) -> (x .and. y?=w442:bool)
                        n191 = Compound Arithmetic op=OR(w443, w445, w442) -> (w450:bool)
                        n192 = call "Write panel message (SubVI).vi"("Stop BurnIn"=w436, 4:"rpm"=w432, 5:"rpm"=TRUE ("rpm"), "PrintTime"=FALSE, "Stop"=w438, "error in (no error)"=w455, "Time to wait"=0.2, "Strin"=w435, "String in"=w439) -> ("error out"=w440:errorcluster)  [unwired: 2 in]
                      }
                      n193 = property class="Bool (strict)"(reference=w396, error in=w407) -> ("Value"=w422:bool)  [unwired: 2 out]
                      n194 = Select(t=T14."Stop", s=w422, f=T14."Result") -> (s? t:f=w419:T14)
                    }
                    frame "MD[1]=1" {
                      w461 = u16 0 ("Motor Speed RPM")
                      n195 = Concatenate Strings(w489, "\nSet Parameters MD[1]=1" ("Strin")) -> (w478:string)
                      n196 = property on="VISA Tester" class="VISAName"() -> ("Value"=w494:refnum<visa-resource-name>)  [unwired: 2 in, 2 out]
                      n197 = call "TesterOption (SubVI).vi"("2 Options"=FALSE, "On/Off"=FALSE, "Tester Option"=T13."Venable", "VISA Refnum in"=w494) -> ("error out"=w495:errorcluster, "VISA Refnum out"=w485:refnum<visa-resource-name>)  [unwired: 6 in]
                      n198 = call "CANSendMotorSpeed.vi"("Remote"=TRUE, "error in (no error)"=w495, "Motor Speed RPM"=w461, "UUT"=w479, "CAN Cluster in"=w499) -> ("error out"=w497:errorcluster)  [unwired: 6 in]
                      n199 = call "Write panel message (SubVI).vi"("Stop BurnIn"=w480, 4:"rpm"=w468, 5:"rpm"=FALSE ("rpm"), "PrintTime"=TRUE, "Stop"=w470, "error in (no error)"=w497, "Time to wait"=20.0, "Strin"=w478, "String in"=w481) -> ("error out"=w467:errorcluster)  [unwired: 2 in]
                      n200 = property on="VenableSpeed" class="DigNum (strict)"("Value"=w461) -> ()  [unwired: 2 in, 2 out]
                      n201 = property on="VISA Marvin" class="VISAName"(error in=w467) -> (error out=w496:errorcluster, "Value"=w501:refnum<visa-resource-name>)  [unwired: 1 in, 1 out]
                      n202 = call "SerialMarvinSendGet.vi"("error in (no error)"=w496, "Clear Log"=FALSE, "write buffer"="EP=1\r\nMD[1]=1\r\n", "VISA resource name"=w501) -> ("error out"=w484:errorcluster)  [unwired: 6 in, 1 out]
                      n203 = call "TesterOption (SubVI).vi"("2 Options"=FALSE, "error in (no error)"=w484, "On/Off"=FALSE, "Tester Option"=T13."Power", "VISA Refnum in"=w485) -> ("error out"=w482:errorcluster, "VISA Refnum out"=w471:refnum<visa-resource-name>)  [unwired: 5 in]
                      n204 = call "Write panel message (SubVI).vi"("Stop BurnIn"=w480, 4:"rpm"=w468, 5:"rpm"=FALSE ("rpm"), "PrintTime"=TRUE, "Stop"=w470, "error in (no error)"=w482, "Time to wait"=25.0, "Strin"=w478, "String in"=w481) -> ("error out"=w472:errorcluster)  [unwired: 2 in]
                      n205 = call "TesterOption (SubVI).vi"("2 Options"=FALSE, "error in (no error)"=w472, "On/Off"=TRUE, "Tester Option"=T13."Venable", "VISA Refnum in"=w471) -> ("error out"=w469:errorcluster)  [unwired: 5 in, 1 out]
                      n206 = call "Time Delay8"("error in (no error)"=w469) -> ("error out"=w465:errorcluster)  [unwired: 10 in]
                      n207 = property class="Bool (strict)"(reference=w470, error in=w465) -> ("Value"=w506:bool)  [unwired: 2 out]
                      n208 = Select(t=T14."Stop", s=w506, f=T14."FullSpeed2") -> (s? t:f=w505:T14)
                    }
                    frame "FullSpeed1" {
                      n209 = property on="5.4.0" class="Bool (strict)"() -> ("Value"=w507:bool)  [unwired: 2 in, 2 out]
                      n210 = case shown="True" w507 {
                        tunnel: [u16 15100 ("t") u16 15100 ("t")] -> w510
                        tunnel: [13700.0 ("t") 13700.0 ("t")] -> w509
                        tunnel: [56.0 ("t") 56.0 ("t")] -> w508
                        frame False {
                        }
                        frame True {
                        }
                      }
                      n211 = Concatenate Strings(w529, "\nFull speed operation " ("string")) -> (w516:string)
                      n212 = Equal?(x=w512, y=u8 95) -> (x = y?=w527:bool)
                      n213 = flat-sequence {
                        tunnel: w522 -> [w550]
                        tunnel: [w550] -> w521
                        tunnel: [w549] -> w520
                        frame #0 {
                          n214 = call <vilib>:"High Resolution Relative Seconds.vi"() -> ("relative seconds"=w549:dbl)
                        }
                      }
                      n215 = Select(t=w510, s=w527, f=u16 12100 ("y")) -> (s? t:f=w511:u16)
                      n216 = call "CANSendMotorSpeed.vi"("Remote"=TRUE, "Motor Speed RPM"=w511, "UUT"=w534, "CAN Cluster in"=w537) -> ("error out"=w532:errorcluster)  [unwired: 7 in]
                      n217 = call "Write panel message (SubVI).vi"("Stop BurnIn"=w517, 4:"rpm"=w531, 5:"rpm"=TRUE ("rpm"), "PrintTime"=FALSE, "Stop"=w519, "error in (no error)"=w532, "Time to wait"=0.2, "Strin"=w516, "String in"=w518) -> ("error out"=w522:errorcluster)  [unwired: 2 in]
                      n218 = Select(t=w509, s=w527, f=11500.0) -> (s? t:f=w524:dbl)
                      n219 = Select(t=w508, s=w527, f=33.0) -> (s? t:f=w523:dbl)
                      n220 = while {
                        tunnel: w531 -> [w552]
                        tunnel: w521 -> [w580]
                        tunnel: [w560] -> w530
                        tunnel: w524 -> [w572]
                        tunnel: w523 -> [w569]
                        tunnel: w520 -> [w567]
                        tunnel: w519 -> [w558]
                        tunnel: w518 -> [w559]
                        tunnel: w517 -> [w556]
                        tunnel: w516 -> [w555]
                        stop <- w574 stop-if-true
                        n221 = property class="DigNum (strict)"(reference=w552, error in=w580) -> (error out=w579:errorcluster, "Value"=w573:dbl)  [unwired: 1 out]
                        "FullSpeed1 Speed" <- w573
                        n222 = call <vilib>:"High Resolution Relative Seconds.vi"() -> ("relative seconds"=w568:dbl)
                        n223 = Subtract(x=w568, y=w567) -> (x-y=w566:dbl)
                        n224 = Greater Or Equal?(x=w566, y=120.0) -> (x >= y?=w564:bool)
                        n225 = Greater Or Equal?(x=w573, y=w572) -> (x >= y?=w571:bool)
                        n226 = property on="VISA Tester" class="VISAName"(error in=w579) -> (error out=w578:errorcluster, "Value"=w577:refnum<visa-resource-name>)  [unwired: 1 in, 1 out]
                        n227 = call "GetADCTester (SubVI).vi"("error in (no error)"=w578, "GetADCTester"=T15."Current", "TimeToGet"=5, "VISA Refnum in"=w577) -> ("error out"=w575:errorcluster, "ADCValOutput Single"=w570:dbl)  [unwired: 5 in, 1 out]
                        "FullSpeed1 Current" <- w570
                        n228 = Greater Or Equal?(x=w570, y=w569) -> (x >= y?=w561:bool)
                        n229 = And(x=w561, y=w571) -> (x .and. y?=w562:bool)
                        n230 = property class="Bool (strict)"(reference=w558) -> ("Value"=w563:bool)  [unwired: 1 in, 2 out]
                        n231 = call "Write panel message (SubVI).vi"("Stop BurnIn"=w556, 4:"rpm"=w552, 5:"rpm"=TRUE ("rpm"), "PrintTime"=FALSE, "Stop"=w558, "error in (no error)"=w575, "Time to wait"=0.2, "Strin"=w555, "String in"=w559) -> ("error out"=w560:errorcluster)  [unwired: 2 in]
                        n232 = Compound Arithmetic op=OR(w563, w562, w564) -> (w574:bool)
                      }
                      n233 = property on="VenableSpeed" class="DigNum (strict)"("Value"=w511) -> ()  [unwired: 2 in, 2 out]
                      n234 = property class="Bool (strict)"(reference=w519, error in=w530) -> ("Value"=w542:bool)  [unwired: 2 out]
                      n235 = Select(t=T14."Stop", s=w542, f=T14."MD[1]=1") -> (s? t:f=w539:T14)
                    }
                    frame "MD[1]=0" {
                      w581 = u16 0 ("Motor Speed RPM")
                      n236 = Concatenate Strings(w608, "\nSet Parameters MD[1]=0" ("Strin")) -> (w597:string)
                      n237 = property on="VISA Tester" class="VISAName"() -> ("Value"=w614:refnum<visa-resource-name>)  [unwired: 2 in, 2 out]
                      n238 = call "TesterOption (SubVI).vi"("2 Options"=FALSE, "On/Off"=FALSE, "Tester Option"=T13."Venable", "VISA Refnum in"=w614) -> ("error out"=w615:errorcluster, "VISA Refnum out"=w604:refnum<visa-resource-name>)  [unwired: 6 in]
                      n239 = call "CANSendMotorSpeed.vi"("Remote"=TRUE, "error in (no error)"=w615, "Motor Speed RPM"=w581, "UUT"=w598, "CAN Cluster in"=w619) -> ("error out"=w617:errorcluster)  [unwired: 6 in]
                      n240 = call "Write panel message (SubVI).vi"("Stop BurnIn"=w599, 4:"rpm"=w594, 5:"rpm"=FALSE ("rpm"), "PrintTime"=FALSE, "Stop"=w588, "error in (no error)"=w617, "Time to wait"=0.2, "Strin"=w597, "String in"=w600) -> ("error out"=w611:errorcluster)  [unwired: 2 in]
                      n241 = property on="VenableSpeed" class="DigNum (strict)"("Value"=w581) -> ()  [unwired: 2 in, 2 out]
                      n242 = property on="VISA Marvin" class="VISAName"(error in=w611) -> (error out=w616:errorcluster, "Value"=w621:refnum<visa-resource-name>)  [unwired: 1 in, 1 out]
                      n243 = call "SerialMarvinSendGet.vi"("error in (no error)"=w616, "Clear Log"=FALSE, "write buffer"="EP=1\r\nMD[1]=0\r\n", "VISA resource name"=w621) -> ("error out"=w603:errorcluster)  [unwired: 6 in, 1 out]
                      n244 = call "TesterOption (SubVI).vi"("2 Options"=FALSE, "error in (no error)"=w603, "On/Off"=FALSE, "Tester Option"=T13."Power", "VISA Refnum in"=w604) -> ("error out"=w601:errorcluster, "VISA Refnum out"=w589:refnum<visa-resource-name>)  [unwired: 5 in]
                      n245 = call "Write panel message (SubVI).vi"("Stop BurnIn"=w599, 4:"rpm"=w594, 5:"rpm"=FALSE ("rpm"), "PrintTime"=TRUE, "Stop"=w588, "error in (no error)"=w601, "Time to wait"=25.0, "Strin"=w597, "String in"=w600) -> ("error out"=w590:errorcluster)  [unwired: 2 in]
                      n246 = call "TesterOption (SubVI).vi"("2 Options"=FALSE, "error in (no error)"=w590, "On/Off"=TRUE, "Tester Option"=T13."Venable", "VISA Refnum in"=w589) -> ("error out"=w587:errorcluster)  [unwired: 5 in, 1 out]
                      n247 = call "Time Delay4"("error in (no error)"=w587) -> ("error out"=w583:errorcluster)  [unwired: 10 in]
                      n248 = property class="Bool (strict)"(reference=w588, error in=w583) -> ("Value"=w626:bool)  [unwired: 2 out]
                      n249 = Select(t=T14."Stop", s=w626, f=T14."FullSpeed1") -> (s? t:f=w625:T14)
                    }
                  }
                }
                n250 = flat-sequence {
                  tunnel: [enum16{"Stop", "Direction", "Venable", "Start"}."Stop"] -> w328
                  tunnel: w327 -> [_]
                  frame #0 {
                  }
                }
              }
              frame "Venable" {
                n251 = call "Find_Number_LineMARVIN.vi"("Test Paragraph"="Enable Test", "TableIn"=w631) -> ("Line number"=w639:i32)  [unwired: 3 in, 3 out]
                n252 = Increment(x=w639) -> (x+1=w627:i32)
                n253 = for {
                  tunnel: u16[] [5000, 0, 5000] -> [w669] mode=indexing
                  tunnel: bool[] [TRUE, FALSE, TRUE] -> [w665] mode=indexing
                  tunnel: w627 -> [w670]
                  tunnel: w638 -> [w668]
                  tunnel: w637 -> [w667]
                  tunnel: w636 -> [w656]
                  tunnel: w635 -> [w660]
                  tunnel: w633 -> [w659]
                  tunnel: w634 -> [w658]
                  tunnel: w631 -> [w652]
                  tunnel: w630 -> [w650]
                  tunnel: [w649] -> w629 mode=indexing
                  i -> [w671]
                  w647 = u16 5000 ("Motor Speed RPM")
                  w673 = 200.0 ("y")
                  n254 = call "CANSendMotorSpeed.vi"("Remote"=TRUE, "Motor Speed RPM"=w647, "UUT"=w667, "CAN Cluster in"=w668) -> ("error out"=w664:errorcluster)  [unwired: 7 in]
                  n255 = property on="VISA Tester" class="VISAName"() -> ("Value"=w663:refnum<visa-resource-name>)  [unwired: 2 in, 2 out]
                  n256 = Add(x=w670, y=w671) -> (x+y=w653:i32)
                  n257 = call "TesterOption (SubVI).vi"("2 Options"=FALSE, "error in (no error)"=w664, "On/Off"=w665, "Tester Option"=T13."Venable", "VISA Refnum in"=w663) -> ("error out"=w662:errorcluster)  [unwired: 5 in, 1 out]
                  n258 = call "Write panel message (SubVI).vi"("Stop BurnIn"=w658, 4:"rpm"=w656, 5:"rpm"=TRUE ("rpm"), "PrintTime"=TRUE, "Stop"=w659, "error in (no error)"=w662, "Time to wait"=15.0, "Strin"=w650, "String in"=w660) -> ("error out"=w661:errorcluster)  [unwired: 2 in]
                  n259 = property class="DigNum (strict)"(reference=w656, error in=w661) -> ("Value"=w651:dbl)  [unwired: 2 out]
                  n260 = Add(x=w669, y=w673) -> (x+y=w675:dbl)
                  n261 = Subtract(x=w669, y=w673) -> (x-y=w674:dbl)
                  n262 = In Range and Coerce(upper limit=w675, x=w651, lower limit=w674) -> (In Range?=w649:bool)  [unwired: 1 out]
                  n263 = call "PassOrFail (SubVI).vi"("index (row)"=w653, "Data in"=w651, "Pass?Fail"=w649, "Table in"=w652) -> ()  [unwired: 7 in, 1 out]
                  "VenableSpeed" <- w647
                }
                n264 = property class="Bool (strict)"(reference=w633) -> ("Value"=w646:bool)  [unwired: 1 in, 2 out]
                n265 = And Array Elements(Boolean array=w629) -> (logical AND=→"VenableResult":bool)
                n266 = Select(t=enum16{"Stop", "Direction", "Venable", "Start"}."Stop", s=w646, f=enum16{"Stop", "Direction", "Venable", "Start"}."Direction") -> (s? t:f=w632:enum16{"Stop", "Direction", "Venable", "Start"})
              }
              frame "Start" {
                w695 = "Enable Test" ("Test Paragraph")
                n267 = property class="Str"(reference=w686, "Value"=w677) -> (reference out=w696:refnum<vi>, error out=w683:errorcluster)  [unwired: 1 in]
                n268 = call "Table_ScrollaBarMarvin.vi"("error in"=w683, "Line to focus"=w695, "reference in"=w687) -> ("error out"=w692:errorcluster)  [unwired: 2 out]
                n269 = call "Reset old test Values (SubVI).vi"("error in"=w692, "Atr in"=w687, "Test Paragraph"=w695) -> ("error out"=w691:errorcluster)  [unwired: 8 in]
                n270 = property on="VISA Tester" class="VISAName"(error in=w691) -> (error out=w690:errorcluster, "Value"=w689:refnum<visa-resource-name>)  [unwired: 1 in, 1 out]
                n271 = property class="Bool (strict)"(reference=w680) -> ("Value"=w700:bool)  [unwired: 1 in, 2 out]
                n272 = call "TesterOption (SubVI).vi"("2 Options"=FALSE, "error in (no error)"=w690, "On/Off"=TRUE, "Tester Option"=T13."Venable", "VISA Refnum in"=w689) -> ("error out"=w688:errorcluster)  [unwired: 5 in, 1 out]
                n273 = Select(t=enum16{"Stop", "Direction", "Venable", "Start"}."Stop", s=w700, f=enum16{"Stop", "Direction", "Venable", "Start"}."Venable") -> (s? t:f=w684:enum16{"Stop", "Direction", "Venable", "Start"})
                n274 = call "Write panel message (SubVI).vi"("Stop BurnIn"=w679, 4:"rpm"=w678, 5:"rpm"=FALSE ("rpm"), "PrintTime"=FALSE, "Stop"=w680, "error in (no error)"=w688, "Time to wait"=0.2, "Strin"=w677, "String in"=w696) -> ()  [unwired: 2 in, 1 out]
              }
            }
          }
        }
        frame "Speed Command" {
          w707 = "Speed Command Test in process..." ("Value")
          w704 = "Speed Command Test" ("Test Paragraph")
          n275 = control-ref of="Pannel User Message"() -> (w719:refnum<vi>)
          n276 = property class="Str"(reference=w719, error in=w718, "Value"=w707) -> (error out=w717:errorcluster)  [unwired: 1 out]
          n277 = call "Table_ScrollaBarMarvin.vi"("error in"=w717, "Line to focus"=w704, "reference in"=w703) -> ("error out"=w720:errorcluster)  [unwired: 2 out]
          n278 = property class="Tbl (strict)"(reference=w703, error in=w720) -> (error out=w722:errorcluster, "Value"=w723:string[][])  [unwired: 1 out]
          n279 = property on="5.4.0" class="Bool (strict)"() -> ("Value"=w702:bool)  [unwired: 2 in, 2 out]
          n280 = Index Array(array=w723, index (col)=1 ("disabled index (col)")) -> (element=w724:string[])  [unwired: 1 in]
          n281 = case shown="True" w702 {
            tunnel: [u16[] [6000, 11500, 15100] u16[] [11500, 12700, 14700]] -> w701
            frame False {
            }
            frame True {
            }
          }
          n282 = call "Find_Number_Line.vi"("error in"=w722, "Test Paragraph"=w704, "Row Headers[]"=w724) -> ("error out"=w705:errorcluster, "Line number"=w708:i32)  [unwired: 1 out]
          n283 = call "Reset old test Values (SubVI).vi"("error in"=w705, "Atr in"=w703, "Test Paragraph"=w704) -> ()  [unwired: 8 in, 1 out]
          n284 = control-ref of="Pannel User Message"() -> (w712:refnum<vi>)
          n285 = control-ref of="Stop Burn-in"() -> (w716:refnum<vi>)
          n286 = control-ref of="Config_CANAT"() -> (w713:refnum<vi>)
          n287 = control-ref of="Motor Speed RPM"() -> (w714:refnum<vi>)
          n288 = control-ref of="UUT"() -> (w715:refnum<vi>)
          n289 = control-ref of="Stop Button"() -> (w710:refnum<vi>)
          n290 = control-ref of="ATR"() -> (w711:refnum<vi>)
          n291 = property on="UUT" class="DigNum (strict)"() -> ("Value"=w706:u8)  [unwired: 2 in, 2 out]
          n292 = while {
            shift-right: [w739] -> _
            shift-left: enum16{"Stop", "StopTime", "Speeds", "Start"}."Start" -> [w740]
            tunnel: w710 -> [w738]
            tunnel: w711 -> [w737]
            tunnel: w712 -> [w736]
            tunnel: w713 -> [w735]
            tunnel: w714 -> [w734]
            tunnel: w715 -> [w733]
            tunnel: w716 -> [w732]
            tunnel: w708 -> [w731]
            tunnel: w707 -> [w730]
            tunnel: w706 -> [w728]
            tunnel: w701 -> [w727]
            stop <- w729 stop-if-true
            n293 = case shown="\"Stop\", Default" w740 {
              tunnel: [w744 w774 w814 w858] -> w739
              tunnel: w738 -> [_ w769 w818 w856]
              tunnel: w737 -> [_ w759 w822 _]
              tunnel: w736 -> [_ w770 w819 _]
              tunnel: w735 -> [w742 w772 w821 _]
              tunnel: w734 -> [_ w767 w816 _]
              tunnel: w733 -> [w743 w771 w813 _]
              tunnel: w732 -> [_ w768 w817 _]
              tunnel: w731 -> [_ _ w823 _]
              tunnel: w730 -> [_ _ w820 _]
              tunnel: [w741 w773 w815 FALSE ("Value")] -> w729
              tunnel: w728 -> [_ _ w807 _]
              tunnel: w727 -> [_ _ w804 _]
              frame "Stop", Default {
                n294 = flat-sequence {
                  tunnel: w743 -> [w748]
                  tunnel: w742 -> [w747]
                  tunnel: [enum16{"Stop", "StopTime", "Speeds", "Start"}."Stop"] -> w744
                  tunnel: [TRUE] -> w741
                  frame #0 {
                    w745 = u16 0 ("Motor Speed RPM")
                    n295 = call "CANSendMotorSpeed.vi"("Remote"=TRUE, "Motor Speed RPM"=w745, "UUT"=w748, "CAN Cluster in"=w747) -> ("error out"=w752:errorcluster)  [unwired: 7 in]
                    n296 = property on="SpeedCommandSpeed" class="DigNum (strict)"("Value"=w745) -> ()  [unwired: 2 in, 2 out]
                    n297 = property on="VISA Tester" class="VISAName"() -> ("Value"=w753:refnum<visa-resource-name>)  [unwired: 2 in, 2 out]
                    n298 = call "TesterOption (SubVI).vi"("2 Options"=FALSE, "error in (no error)"=w752, "On/Off"=FALSE, "Tester Option"=T13."Venable", "VISA Refnum in"=w753) -> ()  [unwired: 5 in, 2 out]
                  }
                  frame #1 {
                  }
                }
              }
              frame "StopTime" {
                w756 = u16 0 ("Motor Speed RPM")
                n299 = call "Table_ScrollaBarMarvin.vi"("Line to focus"="Motor Stop time", "reference in"=w759) -> ("error out"=w760:errorcluster)  [unwired: 1 in, 2 out]
                n300 = property on="SpeedCommandSpeed" class="DigNum (strict)"("Value"=w756) -> ()  [unwired: 2 in, 2 out]
                n301 = call "CANSendMotorSpeed.vi"("Remote"=TRUE, "error in (no error)"=w760, "Motor Speed RPM"=w756, "UUT"=w771, "CAN Cluster in"=w772) -> ("error out"=w777:errorcluster)  [unwired: 6 in]
                n302 = flat-sequence {
                  tunnel: [w803] -> w776
                  tunnel: w777 -> [w802]
                  tunnel: [w802] -> w778
                  frame #0 {
                    n303 = call <vilib>:"High Resolution Relative Seconds.vi"() -> ("relative seconds"=w803:dbl)
                  }
                }
                n304 = while {
                  tunnel: [w798] -> w773
                  tunnel: w770 -> [w796]
                  tunnel: w769 -> [w795]
                  tunnel: w768 -> [w793]
                  tunnel: w767 -> [w792]
                  tunnel: "Stop Time Test in process..." ("Value") -> [w780]
                  tunnel: [w788] -> w757
                  tunnel: w778 -> [w800]
                  tunnel: [w789] -> w765
                  tunnel: w776 -> [w799]
                  tunnel: [w787] -> w761
                  stop <- w779 stop-if-true
                  n305 = call "Write panel message (SubVI).vi"("Stop BurnIn"=w793, 4:"rpm"=w792, 5:"rpm"=TRUE ("rpm"), "PrintTime"=FALSE, "Stop"=w795, "error in (no error)"=w800, "Time to wait"=0.1, "Strin"=w780, "String in"=w796) -> ("error out"=w797:errorcluster)  [unwired: 2 in]
                  n306 = control-ref of="Motor Speed RPM"() -> (w786:refnum<vi>)
                  n307 = property class="DigNum (strict)"(reference=w786, error in=w797) -> (error out=w789:errorcluster, "Value"=w785:dbl)  [unwired: 1 out]
                  n308 = call <vilib>:"High Resolution Relative Seconds.vi"() -> ("relative seconds"=w783:dbl)
                  n309 = property class="Bool (strict)"(reference=w795) -> ("Value"=w798:bool)  [unwired: 1 in, 2 out]
                  n310 = Subtract(x=w783, y=w799) -> (x-y=w787:dbl)
                  n311 = Greater Or Equal?(x=w787, y=50.0) -> (x >= y?=w781:bool)
                  n312 = Less Or Equal?(x=w785, y=0.0) -> (x <= y?=w788:bool)
                  n313 = Compound Arithmetic op=OR(w788, w781, w798) -> (w779:bool)
                }
                "StopTimeResult" <- w757
                n314 = call "Find_Number_LineMARVIN.vi"("Test Paragraph"="Motor Stop time", "TableIn"=w759) -> ("Line number"=w762:i32)  [unwired: 3 in, 3 out]
                n315 = call "PassOrFail (SubVI).vi"("index (row)"=w762, "error in (no error)"=w765, "Data in"=w761, "Pass?Fail"=w757, "Table in"=w759) -> ("error out"=w764:errorcluster)  [unwired: 6 in]
                n316 = flat-sequence {
                  tunnel: [enum16{"Stop", "StopTime", "Speeds", "Start"}."Stop"] -> w774
                  tunnel: w764 -> [_]
                  frame #0 {
                  }
                }
              }
              frame "Speeds" {
                n317 = Equal?(x=w807, y=u8 95) -> (x = y?=w811:bool)
                n318 = Select(t=w804, s=w811, f=u16[] [6000, 9000, 12100]) -> (s? t:f=w809:u16[])
                n319 = for {
                  tunnel: w809 -> [w849] mode=indexing
                  tunnel: w823 -> [w842]
                  tunnel: w822 -> [w841]
                  tunnel: w813 -> [w840]
                  tunnel: w821 -> [w839]
                  tunnel: w820 -> [w838]
                  tunnel: w819 -> [w837]
                  tunnel: w818 -> [w836]
                  tunnel: w817 -> [w834]
                  tunnel: w816 -> [w832]
                  tunnel: [w830] -> w815
                  tunnel: [w829] -> w808
                  tunnel: [w828] -> w806 mode=indexing
                  i -> [w848]
                  stop <- w830 stop-if-true
                  w850 = 200.0 ("y")
                  n320 = Increment(x=w848) -> (x+1=w847:i32)
                  n321 = Add(x=w842, y=w847) -> (x+y=w843:i32)
                  n322 = call "CANSendMotorSpeed.vi"("Remote"=TRUE, "Motor Speed RPM"=w849, "UUT"=w840, "CAN Cluster in"=w839) -> ("error out"=w854:errorcluster)  [unwired: 7 in]
                  n323 = control-ref of="Motor Speed RPM"() -> (w855:refnum<vi>)
                  n324 = call "Write panel message (SubVI).vi"("Stop BurnIn"=w834, 4:"rpm"=w832, 5:"rpm"=TRUE ("rpm"), "PrintTime"=TRUE, "Stop"=w836, "error in (no error)"=w854, "Time to wait"=30.0 ("Delay Time (sec)"), "Strin"=w838, "String in"=w837) -> ("error out"=w846:errorcluster)  [unwired: 2 in]
                  n325 = property class="DigNum (strict)"(reference=w855, error in=w846) -> (error out=w853:errorcluster, "Value"=w831:dbl)  [unwired: 1 out]
                  n326 = property class="Bool (strict)"(reference=w836) -> ("Value"=w830:bool)  [unwired: 1 in, 2 out]
                  n327 = Add(x=w849, y=w850) -> (x+y=w852:dbl)
                  n328 = Subtract(x=w849, y=w850) -> (x-y=w851:dbl)
                  n329 = In Range and Coerce(upper limit=w852, x=w831, lower limit=w851) -> (In Range?=w828:bool)  [unwired: 1 out]
                  n330 = call "PassOrFail (SubVI).vi"("index (row)"=w843, "error in (no error)"=w853, "Data in"=w831, "Pass?Fail"=w828, "Table in"=w841) -> ("error out"=w829:errorcluster)  [unwired: 6 in]
                  "SpeedCommandSpeed" <- w849
                }
                n331 = flat-sequence {
                  tunnel: w815 -> [w827]
                  tunnel: [w825] -> w814
                  tunnel: w808 -> [_]
                  frame #0 {
                    n332 = Select(t=enum16{"Stop", "StopTime", "Speeds", "Start"}."Stop", s=w827, f=enum16{"Stop", "StopTime", "Speeds", "Start"}."StopTime") -> (s? t:f=w825:enum16{"Stop", "StopTime", "Speeds", "Start"})
                  }
                }
                n333 = And Array Elements(Boolean array=w806) -> (logical AND=→"SpeedResult":bool)
              }
              frame "Start" {
                n334 = property on="VISA Tester" class="VISAName"() -> ("Value"=w866:refnum<visa-resource-name>)  [unwired: 2 in, 2 out]
                n335 = call "TesterOption (SubVI).vi"("2 Options"=FALSE, "On/Off"=TRUE, "Tester Option"=T13."Venable", "VISA Refnum in"=w866) -> ("error out"=w857:errorcluster)  [unwired: 6 in, 1 out]
                n336 = property class="Bool (strict)"(reference=w856, error in=w857) -> ("Value"=w862:bool)  [unwired: 2 out]
                n337 = Select(t=enum16{"Stop", "StopTime", "Speeds", "Start"}."Stop", s=w862, f=enum16{"Stop", "StopTime", "Speeds", "Start"}."Speeds") -> (s? t:f=w858:enum16{"Stop", "StopTime", "Speeds", "Start"})
              }
            }
          }
        }
        frame "Stop Time" {
          w870 = "Motor Temperature test in process..." ("Value")
          w868 = "Motor Termistor Input Test" ("Test Paragraph")
          n338 = control-ref of="Pannel User Message"() -> (w878:refnum<vi>)
          n339 = property class="Str"(reference=w878, error in=w877, "Value"=w870) -> (error out=w876:errorcluster)  [unwired: 1 out]
          n340 = call "Table_ScrollaBarMarvin.vi"("error in"=w876, "Line to focus"=w868, "reference in"=w867) -> ("error out"=w880:errorcluster)  [unwired: 2 out]
          n341 = property class="Tbl (strict)"(reference=w867, error in=w880) -> (reference out=w873:refnum<vi>, error out=w882:errorcluster, "Value"=w883:string[][])
          n342 = Index Array(array=w883, index (col)=1 ("disabled index (col)")) -> (element=w884:string[])  [unwired: 1 in]
          n343 = call "Find_Number_LineMARVIN.vi"("Test Paragraph"=w868, "error in"=w882, "TableIn"=w867, "Row Headers[]"=w884) -> ("error out"=w879:errorcluster, "Line number"=w872:i32)  [unwired: 1 in, 2 out]
          n344 = call "Reset old test Values (SubVI).vi"("error in"=w879, "Atr in"=w867, "Test Paragraph"=w868) -> ("error out"=w869:errorcluster)  [unwired: 8 in]
          n345 = property on="Status" class="Bool (strict)"(error in=w869) -> (error out=w874:errorcluster, "Value"=w875:bool)  [unwired: 1 in, 1 out]
          n346 = case shown="True" w875 {
            selector: w875 -> [w888 _]
            tunnel: w874 -> [w890 _]
            tunnel: w873 -> [w887 _]
            tunnel: w872 -> [w886 w893]
            tunnel: w871 -> [_ w898]
            tunnel: w870 -> [_ w894]
            frame False {
              n347 = flat-sequence {
                tunnel: w890 -> [w891]
                tunnel: [w891] -> w889
                frame #0 {
                  n348 = One Button Dialog(message="Please establish RS connection.") -> ()  [unwired: 1 in, 1 out]
                }
              }
              n349 = Increment(x=w886) -> (x+1=w885:i32)
              n350 = call "PassOrFail (SubVI).vi"("index (row)"=w885, "error in (no error)"=w889, "Pass?Fail"=w888, "Table in"=w887) -> ()  [unwired: 7 in, 1 out]
            }
            frame True {
              n351 = control-ref of="Stop Burn-in"() -> (w900:refnum<vi>)
              n352 = control-ref of="Pannel User Message"() -> (w902:refnum<vi>)
              n353 = control-ref of="Config_CANAT"() -> (w896:refnum<vi>)
              n354 = control-ref of="ATR"() -> (w903:refnum<vi>)
              n355 = control-ref of="Motor Speed RPM"() -> (w904:refnum<vi>)
              n356 = control-ref of="UUT"() -> (w895:refnum<vi>)
              n357 = control-ref of="Stop Button"() -> (w901:refnum<vi>)
              n358 = property on="VISA Tester" class="VISAName"() -> ("Value"=w897:refnum<visa-resource-name>)  [unwired: 2 in, 2 out]
              n359 = while {
                shift-right: [w908] -> _
                shift-left: T16."Start" -> [w918]
                tunnel: w900 -> [w917]
                tunnel: w901 -> [w916]
                tunnel: w902 -> [w915]
                tunnel: w903 -> [w914]
                tunnel: w904 -> [w913]
                tunnel: w898 -> [w912]
                tunnel: w897 -> [w911]
                tunnel: w896 -> [w910]
                tunnel: w895 -> [w909]
                tunnel: w894 -> [w906]
                tunnel: w893 -> [w905]
                stop <- w907 stop-if-true
                n360 = case shown="\"Start\"" w918 {
                  tunnel: w917 -> [_ w941 w1000]
                  tunnel: w916 -> [_ w933 w1002]
                  tunnel: w915 -> [_ w942 w1004]
                  tunnel: w914 -> [_ w931 _]
                  tunnel: w913 -> [_ w940 w999]
                  tunnel: w912 -> [_ w945 _]
                  tunnel: w911 -> [w921 w944 w993]
                  tunnel: w910 -> [_ _ w1010]
                  tunnel: w909 -> [_ _ w1009]
                  tunnel: [w919 w934 w995] -> w908
                  tunnel: [w920 FALSE FALSE] -> w907
                  tunnel: w906 -> [_ w943 _]
                  tunnel: w905 -> [_ w930 _]
                  frame "Stop", Default {
                    n361 = flat-sequence {
                      tunnel: w921 -> [w922]
                      tunnel: [TRUE] -> w920
                      tunnel: [T16."Stop"] -> w919
                      frame #0 {
                        n362 = call "TesterOption (SubVI).vi"("2 Options"=FALSE, "On/Off"=FALSE, "Tester Option"=T13."Venable", "VISA Refnum in"=w922) -> ()  [unwired: 6 in, 2 out]
                      }
                      frame #1 {
                      }
                    }
                  }
                  frame "TA[5]" {
                    w946 = T19 [enum."60C", enum."90C", enum."120C"] items=["K15", "K16", "K17", "Venable", "Firmeware", "Fan", "Power", "120C", "110C", "100C", "90C", "80C", "70C", "60C", "50C", "40C", "30C", "25C", "20C", "10C", "0C"]
                    n363 = for {
                      tunnel: w946 -> [w970] mode=indexing
                      tunnel: w945 -> [w969]
                      tunnel: w944 -> [w968]
                      tunnel: w943 -> [w967]
                      tunnel: w942 -> [w966]
                      tunnel: w933 -> [w965]
                      tunnel: w941 -> [w964]
                      tunnel: w940 -> [w963]
                      tunnel: dbl[] [60.0, 90.0, 120.0] -> [w953] mode=indexing
                      tunnel: [w952] -> w932
                      tunnel: w931 -> [w959]
                      tunnel: w930 -> [w958]
                      tunnel: [w947] -> w929 mode=indexing
                      i -> [w956]
                      w951 = 3.0 ("y")
                      n364 = for {
                        N: 5 -> [_]
                        tunnel: w970 -> [w972]
                        tunnel: w969 -> [w988]
                        tunnel: w968 -> [w984]
                        tunnel: w967 -> [w982]
                        tunnel: w966 -> [w981]
                        tunnel: w965 -> [w980]
                        tunnel: w964 -> [w978]
                        tunnel: w963 -> [w975]
                        tunnel: [w974] -> w962 mode=indexing
                        tunnel: [w973] -> w960
                        n365 = call "TesterOption (SubVI).vi"("2 Options"=FALSE, "On/Off"=TRUE, "Tester Option"=w972, "VISA Refnum in"=w984) -> ("error out"=w985:errorcluster)  [unwired: 6 in, 1 out]
                        n366 = call "Write panel message (SubVI).vi"("Stop BurnIn"=w978, 4:"rpm"=w975, 5:"rpm"=FALSE ("rpm"), "PrintTime"=FALSE, "Stop"=w980, "error in (no error)"=w985, "Time to wait"=1.0, "Strin"=w982, "String in"=w981) -> ("error out"=w983:errorcluster)  [unwired: 2 in]
                        n367 = call "SerialMarvinSendGet.vi"("error in (no error)"=w983, "write buffer"="TA[2]\r\n", "VISA resource name"=w988) -> ("error out"=w973:errorcluster, "read buffer"=w986:string)  [unwired: 7 in]
                        n368 = Fract/Exp String To Number(string=w986) -> (number=w974:dbl)  [unwired: 3 in, 1 out]
                      }
                      n369 = Increment(x=w956) -> (x+1=w955:i32)
                      n370 = Add Array Elements(numeric array=w962) -> (sum=w961:dbl)
                      n371 = Add(x=w953, y=w951) -> (x+y=w950:dbl)
                      n372 = Subtract(x=w953, y=w951) -> (x-y=w949:dbl)
                      n373 = Divide(x=w961, y=5.0) -> (x/y=w948:dbl)
                      n374 = In Range and Coerce(upper limit=w950, x=w948, lower limit=w949) -> (In Range?=w947:bool)  [unwired: 1 out]
                      n375 = Add(x=w958, y=w955) -> (x+y=w957:i32)
                      n376 = call "PassOrFail (SubVI).vi"("index (row)"=w957, "error in (no error)"=w960, "Data in"=w948, "Pass?Fail"=w947, "Table in"=w959) -> ("error out"=w952:errorcluster)  [unwired: 6 in]
                    }
                    n377 = property class="Bool (strict)"(reference=w933, error in=w932) -> ("Value"=w938:bool)  [unwired: 2 out]
                    n378 = Select(t=T16."Stop", s=w938, f=T16."Stop") -> (s? t:f=w934:T16)
                    n379 = And Array Elements(Boolean array=w929) -> (logical AND=→"MotorTempResult":bool)
                  }
                  frame "Start" {
                    n380 = call "Write panel message (SubVI).vi"("Stop BurnIn"=w1000, 4:"rpm"=w999, 5:"rpm"=FALSE ("rpm"), "PrintTime"=FALSE, "Stop"=w1002, "Time to wait"=0.1, "Strin"="Motor Temperature test in process...\nInitialization state...", "String in"=w1004) -> ("error out"=w1005:errorcluster)  [unwired: 3 in]
                    n381 = call "TesterOption (SubVI).vi"("2 Options"=FALSE, "error in (no error)"=w1005, "On/Off"=FALSE, "Tester Option"=T13."Venable", "VISA Refnum in"=w993) -> ("error out"=w1007:errorcluster)  [unwired: 5 in, 1 out]
                    n382 = call "CANSendMotorSpeed.vi"("Remote"=TRUE, "error in (no error)"=w1007, "Motor Speed RPM"=u16 0, "UUT"=w1009, "CAN Cluster in"=w1010) -> ("error out"=w992:errorcluster)  [unwired: 6 in]
                    n383 = property class="Bool (strict)"(reference=w1002, error in=w992) -> ("Value"=w1014:bool)  [unwired: 2 out]
                    n384 = Select(t=T16."Stop", s=w1014, f=T16."TA[5]") -> (s? t:f=w995:T16)
                  }
                }
              }
            }
          }
        }
        frame "Temp Control" {
          w1032 = "Temperature control test in process..." ("Value")
          w1030 = "Temperature Control Algorithm Test" ("Test Paragraph")
          n385 = control-ref of="Pannel User Message"() -> (w1043:refnum<vi>)
          n386 = call <vilib>:"Open Config Data.vi"("error in (no error)"=w1026, "create file if necessary (T)"=FALSE, "configuration file path"=w1028) -> ("error out"=w1029:errorcluster, "refnum"=w1025:T12)  [unwired: 7 out]
          n387 = property class="Str"(reference=w1043, error in=w1026, "Value"=w1032) -> (error out=w1042:errorcluster)  [unwired: 1 out]
          n388 = call-poly <vilib>:"Read Key.vi"("section"="Marvin", "error in (no error)"=w1029, "default value"="10", "key"="Temp Algorithm", "refnum"=w1025) -> ("error out"=w1021:errorcluster, "value"=w1019:string, "refnum out"=w1020:T12)  [unwired: 1 in, 3 out]
          n389 = Decimal String To Number(string=w1019) -> (number=w1017:i32)  [unwired: 2 in, 1 out]
          n390 = Less Or Equal To 0?(x=w1017) -> (x <= 0?=w1018:bool)
          n391 = Select(t=10, s=w1018, f=w1017) -> (s? t:f=w1016:i32)
          n392 = call <vilib>:"Close Config Data.vi"("error in (no error)"=w1021, "refnum"=w1020) -> ()  [unwired: 8 in, 2 out]
          n393 = control-ref of="Pannel User Message"() -> (w1037:refnum<vi>)
          n394 = control-ref of="Motor Speed RPM"() -> (w1035:refnum<vi>)
          n395 = control-ref of="Stop Button"() -> (w1039:refnum<vi>)
          n396 = control-ref of="ATR"() -> (w1038:refnum<vi>)
          n397 = control-ref of="Config_CANAT"() -> (w1036:refnum<vi>)
          n398 = control-ref of="UUT"() -> (w1034:refnum<vi>)
          n399 = control-ref of="Stop Burn-in"() -> (w1033:refnum<vi>)
          n400 = call "Table_ScrollaBarMarvin.vi"("error in"=w1042, "Line to focus"=w1030, "reference in"=w1044) -> ("error out"=w1041:errorcluster)  [unwired: 2 out]
          n401 = call "Reset old test Values (SubVI).vi"("error in"=w1041, "Atr in"=w1044, "Test Paragraph"=w1030) -> ("error out"=w1031:errorcluster)  [unwired: 8 in]
          n402 = while {
            tunnel: w1031 -> [w1057]
            shift-right: [w1055] -> _
            shift-left: enum16{"Stop", "Algorithm", "Start"}."Start" -> [w1056]
            tunnel: w1039 -> [w1054]
            tunnel: w1038 -> [w1053]
            tunnel: w1037 -> [w1052]
            tunnel: w1036 -> [w1051]
            tunnel: w1035 -> [w1050]
            tunnel: w1034 -> [w1049]
            tunnel: w1033 -> [w1047]
            tunnel: w1032 -> [w1046]
            tunnel: w1016 -> [w1045]
            stop <- w1048 stop-if-true
            n403 = case shown="\"Algorithm\"" w1056 {
              tunnel: w1057 -> [_ _ w1211]
              tunnel: [w1058 w1082 w1200] -> w1055
              tunnel: w1054 -> [_ w1092 w1204]
              tunnel: w1053 -> [_ w1088 _]
              tunnel: w1052 -> [_ w1093 _]
              tunnel: w1051 -> [w1061 _ w1185]
              tunnel: w1050 -> [_ w1089 _]
              tunnel: w1049 -> [w1060 _ w1184]
              tunnel: [w1059 FALSE FALSE] -> w1048
              tunnel: w1047 -> [_ w1091 _]
              tunnel: w1046 -> [_ w1090 _]
              tunnel: w1045 -> [_ w1076 _]
              frame "Stop", Default {
                n404 = flat-sequence {
                  tunnel: w1061 -> [w1066]
                  tunnel: w1060 -> [w1064]
                  tunnel: [TRUE] -> w1059
                  tunnel: [enum16{"Stop", "Algorithm", "Start"}."Stop"] -> w1058
                  frame #0 {
                    n405 = call "CANSendMotorSpeed.vi"("Remote"=TRUE, "Motor Speed RPM"=u16 0, "UUT"=w1064, "CAN Cluster in"=w1066) -> ("error out"=w1062:errorcluster)  [unwired: 7 in]
                    n406 = property on="VISA Tester" class="VISAName"() -> ("Value"=w1070:refnum<visa-resource-name>)  [unwired: 2 in, 2 out]
                    n407 = call "TesterOption (SubVI).vi"("2 Options"=FALSE, "error in (no error)"=w1062, "On/Off"=FALSE, "Tester Option"=T13."Venable", "VISA Refnum in"=w1070) -> ()  [unwired: 5 in, 2 out]
                  }
                  frame #1 {
                  }
                  frame #2 {
                  }
                }
              }
              frame "Algorithm" {
                w1077 = T20 [enum."6000", enum."11500", enum."15100", enum."11500-2", enum."6000-2"] items=["6000", "11500", "15100", "11500-2", "6000-2"]
                n408 = property on="5.4.0" class="Bool (strict)"() -> ("Value"=w1075:bool)  [unwired: 2 in, 2 out]
                n409 = case shown="True" w1075 {
                  tunnel: [string[] ["Tair <   68 ± 2 °C", "Tair >= 68 ± 2 °C", "Tair >= 88 ± 2 °C", "Tair <= 80 ± 2 °C", "Tair <= 60 ± 2 °C"] string[] ["Tair <   67 ± 3 °C", "Tair >= 67 ± 3 °C", "Tair >= 83 ± 3 °C", "Tair <= 80 ± 3 °C", "Tair <= 64 ± 3 °C"]] -> w1087
                  tunnel: [dbl[] [68.0, 68.0, 88.0, 80.0, 60.0] dbl[] [67.0, 67.0, 83.0, 80.0, 64.0]] -> w1086
                  tunnel: [dbl[] [6000.0, 11500.0, 15100.0, 11500.0, 6000.0] dbl[] [11500.0, 12700.0, 14700.0, 12700.0, 11500.0]] -> w1085
                  tunnel: [dbl[] [6000.0, 6400.0, 11700.0, 14600.0, 11000.0] dbl[] [11500.0, 11700.0, 12900.0, 14400.0, 12000.0]] -> w1084
                  tunnel: [2.0 3.0] -> w1074
                  tunnel: [1288.0 ("Rt") 1202.0 ("Rt")] -> w1073
                  frame False {
                    # "60 Deg"
                    # "Speed Goal"
                    # "Speed Ind"
                    # "Temp Goal"
                  }
                  frame True {
                    # "50 Deg"
                    # "Speed Goal"
                    # "Speed Ind"
                    # "Temp Goal"
                  }
                }
                n410 = for {
                  tunnel: w1093 -> [w1135]
                  tunnel: w1092 -> [w1134]
                  tunnel: w1091 -> [w1133]
                  tunnel: w1090 -> [w1132]
                  tunnel: w1089 -> [w1131]
                  tunnel: w1088 -> [w1118]
                  tunnel: w1087 -> [w1116] mode=indexing
                  shift-right: [w1128] -> _
                  shift-left: w1073 -> [w1129]
                  tunnel: w1086 -> [w1127] mode=indexing
                  tunnel: w1085 -> [w1126] mode=indexing
                  tunnel: w1084 -> [w1125] mode=indexing
                  tunnel: [w1114] -> w1083
                  tunnel: [w1113] -> w1079 mode=indexing
                  tunnel: [w1112] -> w1080 mode=indexing
                  tunnel: w1077 -> [w1111] mode=indexing
                  tunnel: w1076 -> [w1110]
                  tunnel: w1074 -> [w1109]
                  i -> [w1108]
                  stop <- w1130 stop-if-true
                  n411 = call <vilib>:"High Resolution Relative Seconds.vi"() -> ("relative seconds"=w1124:dbl)
                  n412 = while {
                    tunnel: w1135 -> [w1165]
                    tunnel: w1134 -> [w1157]
                    tunnel: w1133 -> [w1164]
                    tunnel: w1132 -> [w1143]
                    tunnel: w1131 -> [w1166]
                    shift-right: [w1162] -> w1128
                    shift-left: w1129 -> [w1161]
                    tunnel: w1111 -> [w1163]
                    tunnel: w1127 -> [w1160]
                    tunnel: w1126 -> [w1159]
                    tunnel: w1125 -> [w1158]
                    tunnel: w1124 -> [w1154]
                    tunnel: [w1149] -> w1119
                    tunnel: [w1148] -> w1112
                    tunnel: [w1147] -> w1117
                    tunnel: [w1146] -> w1113
                    tunnel: [w1145] -> w1115
                    tunnel: w1110 -> [w1137]
                    tunnel: w1109 -> [w1136]
                    stop <- w1155 stop-if-true
                    n413 = call "DegToDAC (SubVI).vi"("R2"=0.0, "Rt"=w1161) -> ("error out"=w1173:errorcluster, "output array"=w1174:u8[])  [unwired: 8 in]
                    n414 = call <vilib>:"High Resolution Relative Seconds.vi"() -> ("relative seconds"=w1153:dbl)
                    n415 = property on="VISA Tester" class="VISAName"() -> ("Value"=w1176:refnum<visa-resource-name>)  [unwired: 2 in, 2 out]
                    n416 = Byte Array To String(unsigned byte array=w1174) -> (string=w1175:string)
                    n417 = Subtract(x=w1154, y=w1153) -> (x-y=w1152:dbl)
                    n418 = VISA Write(VISA resource name=w1176, write buffer=w1175, error in (no error)=w1173) -> (error out=w1172:errorcluster)  [unwired: 2 out]
                    n419 = Greater Or Equal?(x=w1152, y=120.0) -> (x >= y?=w1150:bool)
                    n420 = call <vilib>:"Clear Errors.vi"("error in (no error)"=w1172) -> ("error out"=w1171:errorcluster)  [unwired: 5 in, 1 out]
                    n421 = control-ref of="Ambient Temperature"() -> (w1144:refnum<vi>)
                    n422 = property class="DigNum (strict)"(reference=w1144) -> ("Value"=w1142:dbl)  [unwired: 1 in, 2 out]
                    n423 = property class="Bool (strict)"(reference=w1157) -> ("Value"=w1156:bool)  [unwired: 1 in, 2 out]
                    n424 = Number To Fractional String(number=w1142, precision (6)=i16 2) -> (F-format string=w1139:string)  [unwired: 2 in]
                    n425 = Concatenate Strings(w1143, "\nAmbient  Temp. [C]: " ("string"), w1139) -> (w1138:string)
                    n426 = call "Write panel message (SubVI).vi"("Stop BurnIn"=w1164, 4:"rpm"=w1166, 5:"rpm"=TRUE ("rpm"), "PrintTime"=TRUE, "Stop"=w1157, "error in (no error)"=w1171, "Time to wait"=3.0, "Strin"=w1138, "String in"=w1165) -> ("error out"=w1170:errorcluster)  [unwired: 2 in]
                    n427 = call "TempAlgoTest (SubVI).vi"("Temp"=w1144, "Speed Ind"=w1158, "Motor Speed RPM"=w1166, "Round"=w1163, "Temp Up In"=w1161, "error in (no error)"=w1170, "String in"=w1165, "Temp Goal"=w1160, "Stop"=w1157, "Speed Goal"=w1159, "Stop BurnIn"=w1164, "AD Resistor Step"=w1137, "Strin"=w1138, "AccuTemp"=w1136) -> (14:"Speed Pass/Fail"=w1148:bool, "Temp  Pass/Fail"=w1147:dbl, "Temp Up Out"=w1162:dbl, 17:"Speed Pass/Fail"=w1149:dbl, "Temp Pass/Fail"=w1146:bool, "error out"=w1145:errorcluster)
                    n428 = Compound Arithmetic op=OR(w1150, w1148, w1156) -> (w1155:bool)
                  }
                  n429 = property class="Bool (strict)"(reference=w1134) -> ("Value"=w1130:bool)  [unwired: 1 in, 2 out]
                  n430 = call "Find_Number_LineMARVIN.vi"("Test Paragraph"=w1116, "error in"=w1115, "TableIn"=w1118) -> ("error out"=w1120:errorcluster, "Line number"=w1123:i32)  [unwired: 2 in, 2 out]
                  n431 = Increment(x=w1123) -> (x+1=w1122:i32)
                  n432 = call "PassOrFail (SubVI).vi"("index (row)"=w1122, "error in (no error)"=w1120, "Data in"=w1117, "Pass?Fail"=w1113, "Table in"=w1118) -> ("error out"=w1121:errorcluster)  [unwired: 6 in]
                  n433 = call "PassOrFail (SubVI).vi"("index (row)"=w1123, "error in (no error)"=w1121, "Data in"=w1119, "Pass?Fail"=w1112, "Table in"=w1118) -> ("error out"=w1114:errorcluster)  [unwired: 6 in]
                  "Numeric 3" <- w1108
                }
                n434 = Build Array (concatenate)(w1080, w1079) -> (w1081:bool[])
                n435 = flat-sequence {
                  tunnel: w1083 -> [_]
                  tunnel: [enum16{"Stop", "Algorithm", "Start"}."Stop"] -> w1082
                  frame #0 {
                  }
                }
                n436 = And Array Elements(Boolean array=w1081) -> (logical AND=→"TempControlResult":bool)
              }
              frame "Start" {
                n437 = call <vilib>:"Clear Errors.vi"("error in (no error)"=w1211) -> ("error out"=w1186:errorcluster)  [unwired: 5 in, 1 out]
                n438 = call "CANSendMotorSpeed.vi"("Remote"=TRUE, "error in (no error)"=w1186, "Motor Speed RPM"=u16 0, "UUT"=w1184, "CAN Cluster in"=w1185) -> ("error out"=w1181:errorcluster)  [unwired: 6 in]
                n439 = call "Time Delay15"("error in (no error)"=w1181) -> ("error out"=w1180:errorcluster)  [unwired: 10 in]
                n440 = call "DegToDAC (SubVI).vi"("error in (no error)"=w1180, "R2"=0.0, "Rt"=1202.0) -> ("error out"=w1191:errorcluster, "output array"=w1192:u8[])  [unwired: 7 in]
                n441 = property on="VISA Tester" class="VISAName"() -> ("Value"=w1194:refnum<visa-resource-name>)  [unwired: 2 in, 2 out]
                n442 = Byte Array To String(unsigned byte array=w1192) -> (string=w1193:string)
                n443 = VISA Write(VISA resource name=w1194, write buffer=w1193, error in (no error)=w1191) -> (error out=w1183:errorcluster)  [unwired: 2 out]
                n444 = call "Time Delay16"("error in (no error)"=w1183) -> ("error out"=w1182:errorcluster)  [unwired: 10 in]
                n445 = property on="VISA Tester" class="VISAName"() -> ("Value"=w1210:refnum<visa-resource-name>)  [unwired: 2 in, 2 out]
                n446 = call "TesterOption (SubVI).vi"("On/Off 2"=TRUE, "Tester Option 2"=T13."Venable", "2 Options"=TRUE, "error in (no error)"=w1182, "On/Off"=TRUE, "Tester Option"=T13."K16", "VISA Refnum in"=w1210) -> ("error out"=w1196:errorcluster)  [unwired: 3 in, 1 out]
                n447 = call "Time Delay12"("error in (no error)"=w1196) -> ("error out"=w1195:errorcluster)  [unwired: 10 in]
                n448 = call "CANSendMotorSpeed.vi"("Remote"=FALSE, "error in (no error)"=w1195, "Motor Speed RPM"=u16 0, "UUT"=w1184, "CAN Cluster in"=w1185) -> ("error out"=w1179:errorcluster)  [unwired: 6 in]
                n449 = call "Time Delay17"("error in (no error)"=w1179) -> ("error out"=w1178:errorcluster)  [unwired: 10 in]
                n450 = property class="Bool (strict)"(reference=w1204, error in=w1178) -> ("Value"=w1203:bool)  [unwired: 2 out]
                n451 = Select(t=enum16{"Stop", "Algorithm", "Start"}."Stop", s=w1203, f=enum16{"Stop", "Algorithm", "Start"}."Algorithm") -> (s? t:f=w1200:enum16{"Stop", "Algorithm", "Start"})
              }
            }
          }
        }
        frame "Burn in" {
          n452 = property on="5.4.0" class="Bool (strict)"() -> ("Value"=w1216:bool)  [unwired: 2 in, 2 out]
          n453 = control-ref of="Stop Button"() -> (w1222:refnum<vi>)
          n454 = case shown="True" w1216 {
            tunnel: [u16 15100 ("y") u16 14700 ("y")] -> w1215
            tunnel: [50.0 ("y") 45.0 ("y")] -> w1214
            tunnel: [15100.0 ("y") 14700.0 ("y")] -> w1213
            tunnel: [u16 15100 ("t") u16 14700 ("t")] -> w1212
            frame False {
            }
            frame True {
            }
          }
          n455 = control-ref of="Pannel User Message"() -> (w1225:refnum<vi>)
          n456 = control-ref of="ATR"() -> (w1221:refnum<vi>)
          n457 = control-ref of="Config_CANAT"() -> (w1224:refnum<vi>)
          n458 = control-ref of="UUT"() -> (w1223:refnum<vi>)
          n459 = control-ref of="Stop Burn-in"() -> (w1220:refnum<vi>)
          n460 = property on="UUT" class="DigNum (strict)"() -> ("Value"=w1219:u8)  [unwired: 2 in, 2 out]
          n461 = while {
            tunnel: w1225 -> [w1251]
            tunnel: w1221 -> [w1250]
            tunnel: w1224 -> [w1249]
            tunnel: w1223 -> [w1248]
            tunnel: w1222 -> [w1247]
            shift-right: [w1246] -> _
            shift-left: T17."Start" -> [w1253]
            shift-right: [w1252] -> _
            shift-left: _ -> [w1244]
            tunnel: w1220 -> [w1243]
            tunnel: w1219 -> [w1242]
            tunnel: w1218 -> [w1241]
            shift-right: [w1240] -> _
            shift-left: FALSE -> [w1239]
            tunnel: w1215 -> [w1238]
            tunnel: w1214 -> [w1237]
            tunnel: w1213 -> [w1236]
            tunnel: w1212 -> [w1235]
            stop <- w1245 stop-if-true
            n462 = case shown="\"Stop\", Default" w1253 {
              tunnel: [w1259 w1295 w1363 w1390 w1420 w1455] -> w1252
              tunnel: w1251 -> [_ w1287 _ _ _ w1454]
              tunnel: w1250 -> [_ w1290 w1336 w1378 w1407 w1441]
              tunnel: w1249 -> [w1255 w1286 _ _ _ w1453]
              tunnel: w1248 -> [w1254 w1283 _ _ _ w1434]
              tunnel: w1247 -> [_ _ w1365 w1392 w1424 w1447]
              tunnel: [w1257 T17."Stop" w1366 w1393 w1425 w1443] -> w1246
              tunnel: [w1258 FALSE FALSE FALSE FALSE FALSE] -> w1245
              tunnel: w1244 -> [w1259 w1295 w1363 w1390 w1420 _]
              tunnel: w1243 -> [_ _ _ _ _ w1437]
              tunnel: w1242 -> [_ w1280 w1330 w1373 w1402 w1433]
              tunnel: w1241 -> [_ w1276 _ _ _ _]
              tunnel: [FALSE ("Stop Burn-in") w1275 FALSE w1371 w1399 FALSE ("Stop Burn-in")] -> w1240
              tunnel: w1239 -> [_ _ w1325 _ _ _]
              tunnel: w1238 -> [_ _ _ _ _ w1428]
              tunnel: w1237 -> [_ _ _ _ w1397 _]
              tunnel: w1236 -> [_ _ _ w1369 _ _]
              tunnel: w1235 -> [_ w1273 _ _ _ _]
              frame "Stop", Default {
                n463 = flat-sequence {
                  tunnel: w1255 -> [w1262]
                  tunnel: w1254 -> [w1261]
                  tunnel: [TRUE] -> w1258
                  tunnel: [T17."Stop"] -> w1257
                  frame #0 {
                    w1260 = u16 0 ("Motor Speed RPM")
                    n464 = call "CANSendMotorSpeed.vi"("Remote"=TRUE, "Motor Speed RPM"=w1260, "UUT"=w1261, "CAN Cluster in"=w1262) -> ("error out"=w1264:errorcluster)  [unwired: 7 in]
                    n465 = property on="BurnInSpeed" class="DigNum (strict)"("Value"=w1260) -> ()  [unwired: 2 in, 2 out]
                    n466 = property on="VISA Tester" class="VISAName"() -> ("Value"=w1269:refnum<visa-resource-name>)  [unwired: 2 in, 2 out]
                    n467 = call "TesterOption (SubVI).vi"("2 Options"=FALSE, "error in (no error)"=w1264, "On/Off"=FALSE, "Tester Option"=T13."Venable", "VISA Refnum in"=w1269) -> ("error out"=w1266:errorcluster)  [unwired: 5 in, 1 out]
                    n468 = property on="Stop Burn-in" class="Bool (strict)"(error in=w1266, "Visible"=FALSE) -> ()  [unwired: 1 in, 2 out]
                  }
                  frame #1 {
                  }
                }
              }
              frame "BurnIn" {
                w1275 = FALSE ("Stop Burn-in")
                n469 = control-ref of="Motor Speed RPM"() -> (w1289:refnum<vi>)
                n470 = control-ref of="Stop Button"() -> (w1288:refnum<vi>)
                n471 = property on="Stop Burn-in" class="Bool (strict)"("Visible"=w1276) -> (error out=w1291:errorcluster)  [unwired: 2 in, 1 out]
                n472 = Equal?(x=w1280, y=u8 95) -> (x = y?=w1279:bool)
                n473 = call "Find_Number_LineMARVIN.vi"("Test Paragraph"="After 10 min of operation", "error in"=w1291, "TableIn"=w1290) -> ("error out"=w1293:errorcluster, "Line number"=w1294:i32)  [unwired: 2 in, 2 out]
                n474 = Select(t=w1273, s=w1279, f=u16 12100 ("y")) -> (s? t:f=w1282:u16)
                n475 = for {
                  tunnel: w1293 -> [w1312]
                  tunnel: dbl[] [600.0, 600.0, 600.0] -> [w1316] mode=indexing
                  tunnel: w1294 -> [w1321]
                  tunnel: w1290 -> [w1311]
                  tunnel: w1289 -> [w1310]
                  tunnel: w1288 -> [w1309]
                  tunnel: w1287 -> [w1308]
                  tunnel: w1286 -> [w1304]
                  tunnel: w1283 -> [w1303]
                  tunnel: w1282 -> [w1299]
                  tunnel: [w1301] -> w1281
                  tunnel: [w1300] -> w1278 mode=indexing
                  i -> [w1318]
                  n476 = call "CANSendMotorSpeed.vi"("Remote"=TRUE, "error in (no error)"=w1312, "Motor Speed RPM"=w1299, "UUT"=w1303, "CAN Cluster in"=w1304) -> ("error out"=w1306:errorcluster)  [unwired: 6 in]
                  n477 = control-ref of="Stop Burn-in"() -> (w1307:refnum<vi>)
                  n478 = Add(x=w1321, y=w1318) -> (x+y=w1317:i32)
                  n479 = call "Write panel message (SubVI).vi"("Stop BurnIn"=w1307, 4:"rpm"=w1310, 5:"rpm"=TRUE ("rpm"), "PrintTime"=TRUE, "Stop"=w1309, "error in (no error)"=w1306, "Time to wait"=w1316, "Strin"="Burn-in test in process...", "String in"=w1308) -> ("error out"=w1313:errorcluster)  [unwired: 2 in]
                  n480 = control-ref of="Power transistor Heat sink Temp."() -> (w1322:refnum<vi>)
                  n481 = property on="MaxBurnInTempVal" class="DigNum (strict)"() -> ("Value"=w1320:dbl)  [unwired: 2 in, 2 out]
                  n482 = property class="DigNum (strict)"(reference=w1322, error in=w1313) -> (error out=w1302:errorcluster, "Value"=w1319:dbl)  [unwired: 1 out]
                  n483 = property on="BurnInSpeed" class="DigNum (strict)"("Value"=w1299) -> ()  [unwired: 2 in, 2 out]
                  n484 = Less Or Equal?(x=w1319, y=w1320) -> (x <= y?=w1300:bool)
                  n485 = call "PassOrFail (SubVI).vi"("index (row)"=w1317, "error in (no error)"=w1302, "Data in"=w1319, "Pass?Fail"=w1300, "Table in"=w1311) -> ("error out"=w1301:errorcluster)  [unwired: 6 in]
                }
                n486 = And Array Elements(Boolean array=w1278) -> (logical AND=→"BurnResult":bool)
                n487 = property on="Stop Burn-in" class="Bool (strict)"(error in=w1281, "Value"=w1275, "Visible"=w1275) -> ()  [unwired: 1 in, 2 out]
              }
              frame "Ambient Temp" {
                w1341 = 2 ("disabled index (col)")
                n488 = control-ref of="Power transistor Heat sink Temp."() -> (w1351:refnum<vi>)
                n489 = call "Find_Number_LineMARVIN.vi"("Test Paragraph"="Ambient Temperature", "TableIn"=w1336) -> ("error out"=w1362:errorcluster, "Line number"=w1342:i32)  [unwired: 3 in, 2 out]
                n490 = Equal?(x=w1330, y=u8 95) -> (x = y?=w1331:bool)
                n491 = property class="DigNum (strict)"(reference=w1351, error in=w1362) -> (error out=w1353:errorcluster, "Value"=w1343:dbl)  [unwired: 1 out]
                n492 = Select(t=25.0 ("y"), s=w1331, f=25.0 ("y")) -> (s? t:f=w1352:dbl)
                n493 = Select(t=13.0 ("y"), s=w1331, f=13.0) -> (s? t:f=w1354:dbl)
                n494 = Add(x=w1352, y=w1354) -> (x+y=w1361:dbl)
                n495 = Subtract(x=w1352, y=w1354) -> (x-y=w1360:dbl)
                n496 = In Range and Coerce(upper limit=w1361, x=w1343, lower limit=w1360) -> (In Range?=w1327:bool)  [unwired: 1 out]
                "BurnTemp" <- w1327
                n497 = call "PassOrFail (SubVI).vi"("index (row)"=w1342, "error in (no error)"=w1353, "Data in"=w1343, "Pass?Fail"=w1327, "Table in"=w1336) -> ("error out"=w1333:errorcluster)  [unwired: 6 in]
                n498 = property class="Tbl (strict)"(reference=w1336, error in=w1333) -> (reference out=w1335:refnum<vi>, error out=w1350:errorcluster, "Value"=w1349:string[][])
                n499 = Add(x=w1343, y=25.0) -> (x+y=w1334:dbl)
                "MaxBurnInTempVal" <- w1334
                n500 = Number To Fractional String(number=w1334, precision (6)=i16 0) -> (F-format string=w1348:string)  [unwired: 2 in]
                n501 = Concatenate Strings("< " ("string"), w1348) -> (w1337:string)
                n502 = Increment(x=w1342) -> (x+1=w1340:i32)
                n503 = Increment(x=w1340) -> (x+1=w1339:i32)
                n504 = Increment(x=w1339) -> (x+1=w1338:i32)
                n505 = Replace Array Subset(array=w1349, new element #1=w1337, index (row) #1=w1340, index (col) #1=w1341, new element #2=w1337, index (row) #2=w1339, index (col) #2=w1341, new element #3=w1337, index (row) #3=w1338, index (col) #3=w1341) -> (w1347:string[][])
                n506 = Not(x=w1327) -> (.not. x?=w1326:bool)
                n507 = property class="Tbl (strict)"(reference=w1335, error in=w1350, "Value"=w1347) -> (error out=w1332:errorcluster)  [unwired: 1 out]
                n508 = property class="Bool (strict)"(reference=w1365, error in=w1332) -> ("Value"=w1328:bool)  [unwired: 2 out]
                n509 = Compound Arithmetic op=OR(w1326, w1325, w1328) -> (w1329:bool)
                n510 = Select(t=T17."Stop", s=w1329, f=T17."BurnIn") -> (s? t:f=w1366:T17)
              }
              frame "MotorSpeed" {
                n511 = control-ref of="Motor Speed RPM"() -> (w1376:refnum<vi>)
                n512 = Equal?(x=w1373, y=u8 95) -> (x = y?=w1374:bool)
                n513 = call "Find_Number_LineMARVIN.vi"("Test Paragraph"="Fan speed", "TableIn"=w1378) -> ("error out"=w1389:errorcluster, "Line number"=w1381:i32)  [unwired: 3 in, 2 out]
                n514 = property class="DigNum (strict)"(reference=w1376, error in=w1389) -> (error out=w1379:errorcluster, "Value"=w1380:dbl)  [unwired: 1 out]
                n515 = Select(t=w1369, s=w1374, f=12100.0 ("y")) -> (s? t:f=w1377:dbl)
                n516 = Select(t=200.0 ("y"), s=w1374, f=200.0) -> (s? t:f=w1382:dbl)
                n517 = Add(x=w1377, y=w1382) -> (x+y=w1388:dbl)
                n518 = Subtract(x=w1377, y=w1382) -> (x-y=w1387:dbl)
                n519 = In Range and Coerce(upper limit=w1388, x=w1380, lower limit=w1387) -> (In Range?=w1372:bool)  [unwired: 1 out]
                "BurnSpeed" <- w1372
                n520 = call "PassOrFail (SubVI).vi"("index (row)"=w1381, "error in (no error)"=w1379, "Data in"=w1380, "Pass?Fail"=w1372, "Table in"=w1378) -> ("error out"=w1375:errorcluster)  [unwired: 6 in]
                n521 = property class="Bool (strict)"(reference=w1392, error in=w1375) -> ("Value"=w1396:bool)  [unwired: 2 out]
                n522 = Select(t=T17."Stop", s=w1396, f=T17."Ambient Temp") -> (s? t:f=w1393:T17)
                n523 = Not(x=w1372) -> (.not. x?=w1371:bool)
              }
              frame "DC Current Measure" {
                n524 = property on="VISA Tester" class="VISAName"() -> (error out=w1418:errorcluster, "Value"=w1422:refnum<visa-resource-name>)  [unwired: 2 in, 1 out]
                n525 = call "GetADCTester (SubVI).vi"("error in (no error)"=w1418, "GetADCTester"=T15."Current", "TimeToGet"=10, "VISA Refnum in"=w1422) -> ("error out"=w1419:errorcluster, "ADCValOutput Single"=w1406:dbl)  [unwired: 5 in, 1 out]
                n526 = Equal?(x=w1402, y=u8 95) -> (x = y?=w1403:bool)
                n527 = call "Find_Number_LineMARVIN.vi"("Test Paragraph"="DC Input Current", "error in"=w1419, "TableIn"=w1407) -> ("error out"=w1417:errorcluster, "Line number"=w1408:i32)  [unwired: 2 in, 2 out]
                n528 = Select(t=w1397, s=w1403, f=28.0 ("y")) -> (s? t:f=w1410:dbl)
                n529 = Select(t=5.0 ("y"), s=w1403, f=3.0) -> (s? t:f=w1409:dbl)
                n530 = Add(x=w1410, y=w1409) -> (x+y=w1416:dbl)
                n531 = Subtract(x=w1410, y=w1409) -> (x-y=w1415:dbl)
                n532 = In Range and Coerce(upper limit=w1416, x=w1406, lower limit=w1415) -> (In Range?=w1401:bool)  [unwired: 1 out]
                "BurnDC" <- w1401
                n533 = call "PassOrFail (SubVI).vi"("index (row)"=w1408, "error in (no error)"=w1417, "Data in"=w1406, "Pass?Fail"=w1401, "Table in"=w1407) -> ("error out"=w1405:errorcluster)  [unwired: 6 in]
                n534 = property class="Bool (strict)"(reference=w1424, error in=w1405) -> ("Value"=w1400:bool)  [unwired: 2 out]
                n535 = Not(x=w1401) -> (.not. x?=w1399:bool)
                n536 = Select(t=T17."Stop", s=w1400, f=T17."MotorSpeed") -> (s? t:f=w1425:T17)
              }
              frame "Start" {
                w1429 = "Burn-in Test" ("Line to focus")
                w1431 = "Burn-in test in process...\nFull Speed Operation" ("Value")
                n537 = Equal?(x=w1433, y=u8 95) -> (x = y?=w1435:bool)
                n538 = property class="Str"(reference=w1454, "Value"=w1431) -> (reference out=w1451:refnum<vi>, error out=w1436:errorcluster)  [unwired: 1 in]
                n539 = call "Find_Number_LineMARVIN.vi"("Test Paragraph"=w1429, "error in"=w1436, "TableIn"=w1441) -> ("error out"=w1460:errorcluster, "Line number"=w1461:i32)  [unwired: 2 in, 2 out]
                n540 = Select(t=w1428, s=w1435, f=u16 12100 ("y")) -> (s? t:f=w1467:u16)
                "BurnInSpeed" <- w1467
                n541 = call "Table_ScrollaBarMarvin.vi"("error in"=w1460, "Line to focus"=w1429, "reference in"=w1441) -> ("error out"=w1462:errorcluster)  [unwired: 2 out]
                n542 = call "Reset old test Values (SubVI).vi"("error in"=w1462, "Atr in"=w1441, "Test Paragraph"=w1429) -> ("error out"=w1463:errorcluster)  [unwired: 8 in]
                n543 = Increment(x=w1461) -> (x+1=w1455:i32)
                n544 = property on="VISA Tester" class="VISAName"(error in=w1463) -> (error out=w1464:errorcluster, "Value"=w1465:refnum<visa-resource-name>)  [unwired: 1 in, 1 out]
                n545 = call "TesterOption (SubVI).vi"("2 Options"=FALSE, "error in (no error)"=w1464, "On/Off"=TRUE, "Tester Option"=T13."Venable", "VISA Refnum in"=w1465) -> ("error out"=w1466:errorcluster)  [unwired: 5 in, 1 out]
                n546 = call "CANSendMotorSpeed.vi"("Remote"=TRUE, "error in (no error)"=w1466, "Motor Speed RPM"=w1467, "UUT"=w1434, "CAN Cluster in"=w1453) -> ("error out"=w1452:errorcluster)  [unwired: 6 in]
                n547 = control-ref of="Motor Speed RPM"() -> (w1440:refnum<vi>)
                n548 = call "Write panel message (SubVI).vi"("Stop BurnIn"=w1437, 4:"rpm"=w1440, 5:"rpm"=TRUE ("rpm"), "PrintTime"=TRUE, "Stop"=w1447, "error in (no error)"=w1452, "Time to wait"=50.0, "Strin"=w1431, "String in"=w1451) -> ("error out"=w1439:errorcluster)  [unwired: 2 in]
                n549 = property class="Bool (strict)"(reference=w1447, error in=w1439) -> ("Value"=w1446:bool)  [unwired: 2 out]
                n550 = Select(t=T17."Stop", s=w1446, f=T17."DC Current Measure") -> (s? t:f=w1443:T17)
              }
            }
          }
        }
        frame "Visual Inspec" {
          n551 = control-ref of="Stop Button"() -> (w1471:refnum<vi>)
          n552 = property class="Bool (strict)"(reference=w1471, error in=w1470) -> (error out=w1469:errorcluster, "Value"=w1468:bool)  [unwired: 1 out]
          n553 = case shown="False" w1468 {
            tunnel: w1472 -> [w1486 _]
            tunnel: w1469 -> [w1473 _]
            frame False {
              n554 = property on="VISA Tester" class="VISAName"() -> ("Value"=w1485:refnum<visa-resource-name>)  [unwired: 2 in, 2 out]
              n555 = call "TesterOption (SubVI).vi"("2 Options"=FALSE, "error in (no error)"=w1473, "On/Off"=FALSE, "Tester Option"=T13."Venable", "VISA Refnum in"=w1485) -> ("error out"=w1481:errorcluster)  [unwired: 5 in, 1 out]
              n556 = local read "UUT"() -> (w1477:u8)
              n557 = Equal?(x=w1477, y=u8 95) -> (x = y?=w1478:bool)
              n558 = case shown="True" w1478 {
                tunnel: w1486 -> [w1490 w1500]
                tunnel: w1481 -> [w1489 w1499]
                tunnel: [w1491 w1502] -> w1480
                tunnel: [w1492 w1501] -> w1476
                tunnel: string[] ["Verification of Components Not Installed", "Manufacturing Defects", "DC Input Current Drawn", "12V", "5V", "3.3V", "1.8V", "Reverse Polarity Test - DC Input Current", "Weight Check", "J3.B to Chassis", "J1.16 to Chassis", "J1 Body to Chassis", "J2  Body to Chassis", "J3  Body to Chassis", "J1.17 to J1.18", "Sealing Test", "Mounting Holes Test - Jig Fit"] ("deleted portion 3") -> [w1487 w1497]
                frame False {
                  # "AHU"
                  n559 = for {
                    tunnel: w1487 -> [w1496] mode=indexing
                    tunnel: w1490 -> [w1495]
                    tunnel: w1489 -> [w1494]
                    tunnel: [w1493] -> w1488
                    n560 = call "Reset old test Values (SubVI).vi"("error in"=w1494, "Atr in"=w1495, "Test Paragraph"=w1496) -> ("error out"=w1493:errorcluster)  [unwired: 8 in]
                  }
                  n561 = call "VisualInspectionAHUold.vi"("error in (no error)"=w1488, "TableRef"=w1490) -> ("error out"=w1492:errorcluster, "VisualInspectionResult"=w1491:bool)  [unwired: 8 in]
                }
                frame True {
                  # "EBAY"
                  n562 = for {
                    tunnel: w1500 -> [w1506]
                    tunnel: w1499 -> [w1505]
                    tunnel: [w1504] -> w1498
                    tunnel: w1497 -> [w1503] mode=indexing
                    n563 = call "Reset old test Values (SubVI).vi"("error in"=w1505, "Atr in"=w1506, "Test Paragraph"=w1503) -> ("error out"=w1504:errorcluster)  [unwired: 8 in]
                  }
                  n564 = call "VisualInspectionEBAYold.vi"("error in (no error)"=w1498, "TableRef"=w1500) -> ("error out"=w1501:errorcluster, "VisualInspectionResult"=w1502:bool)  [unwired: 8 in]
                }
              }
              "VisualInspectionResult" <- w1480
              n565 = property on="Automation" class="Bool (strict)"(error in=w1476) -> ("Value"=w1475:bool)  [unwired: 1 in, 2 out]
              n566 = case shown="True" w1475 {
                frame False {
                }
                frame True {
                  w1507 = TRUE ("Value (Signaling)")
                  n567 = property on="SetSN" class="Bool (strict)"("Val(Sgnl)"=w1507, "Value"=w1507) -> ()  [unwired: 2 in, 2 out]
                }
              }
            }
            frame True {
            }
          }
        }
        frame "Temp Sens Cal" {
          w1511 = "Temperature sensor calibration test in process..." ("Value")
          w1509 = "Temperature Sensor Calibration" ("Test Paragraph")
          n568 = control-ref of="Pannel User Message"() -> (w1518:refnum<vi>)
          n569 = property class="Str"(reference=w1518, error in=w1517, "Value"=w1511) -> (error out=w1516:errorcluster)  [unwired: 1 out]
          n570 = call "Table_ScrollaBarMarvin.vi"("error in"=w1516, "Line to focus"=w1509, "reference in"=w1519) -> ("error out"=w1521:errorcluster)  [unwired: 2 out]
          n571 = property class="Tbl (strict)"(reference=w1519, error in=w1521) -> (reference out=w1508:refnum<vi>, error out=w1523:errorcluster, "Value"=w1524:string[][])
          n572 = Index Array(array=w1524, index (col)=1 ("disabled index (col)")) -> (element=w1525:string[])  [unwired: 1 in]
          n573 = call "Find_Number_Line.vi"("error in"=w1523, "Test Paragraph"=w1509, "Row Headers[]"=w1525) -> ("error out"=w1520:errorcluster, "Line number"=w1513:i32)  [unwired: 1 out]
          n574 = property on="Status" class="Bool (strict)"(error in=w1520) -> (error out=w1514:errorcluster, "Value"=w1515:bool)  [unwired: 1 in, 1 out]
          n575 = call "Reset old test Values (SubVI).vi"("error in"=w1514, "Atr in"=w1508, "Test Paragraph"=w1509) -> ("error out"=w1510:errorcluster)  [unwired: 8 in]
          n576 = case shown="True" w1515 {
            selector: w1515 -> [w1529 _]
            tunnel: w1510 -> [w1531 _]
            tunnel: w1508 -> [w1528 _]
            tunnel: w1513 -> [w1527 _]
            tunnel: w1512 -> [_ w1538]
            tunnel: w1511 -> [_ w1534]
            frame False {
              n577 = flat-sequence {
                tunnel: w1531 -> [w1532]
                tunnel: [w1532] -> w1530
                frame #0 {
                  n578 = One Button Dialog(message="Please establish RS connection.") -> ()  [unwired: 1 in, 1 out]
                }
              }
              n579 = Increment(x=w1527) -> (x+1=w1526:i32)
              n580 = call "PassOrFail (SubVI).vi"("index (row)"=w1526, "error in (no error)"=w1530, "Pass?Fail"=w1529, "Table in"=w1528) -> ()  [unwired: 7 in, 1 out]
            }
            frame True {
              n581 = control-ref of="Stop Burn-in"() -> (w1540:refnum<vi>)
              n582 = control-ref of="Pannel User Message"() -> (w1542:refnum<vi>)
              n583 = control-ref of="Config_CANAT"() -> (w1536:refnum<vi>)
              n584 = control-ref of="ATR"() -> (w1543:refnum<vi>)
              n585 = control-ref of="Motor Speed RPM"() -> (w1544:refnum<vi>)
              n586 = control-ref of="UUT"() -> (w1535:refnum<vi>)
              n587 = control-ref of="Stop Button"() -> (w1541:refnum<vi>)
              n588 = property on="VISA Tester" class="VISAName"() -> ("Value"=w1537:refnum<visa-resource-name>)  [unwired: 2 in, 2 out]
              n589 = while {
                shift-right: [w1547] -> _
                shift-left: T16."Start" -> [w1557]
                tunnel: w1540 -> [w1556]
                tunnel: w1541 -> [w1555]
                tunnel: w1542 -> [w1554]
                tunnel: w1543 -> [w1553]
                tunnel: w1544 -> [w1552]
                tunnel: w1538 -> [w1551]
                tunnel: w1537 -> [w1550]
                tunnel: w1536 -> [w1549]
                tunnel: w1535 -> [w1548]
                tunnel: w1534 -> [w1545]
                stop <- w1546 stop-if-true
                n590 = case shown="\"Stop\", Default" w1557 {
                  tunnel: w1556 -> [_ w1592 w1619 w1674 w1704]
                  tunnel: w1555 -> [_ w1593 w1611 w1660 w1706]
                  tunnel: w1554 -> [_ w1590 w1620 w1672 w1708]
                  tunnel: w1553 -> [_ w1570 _ _ _]
                  tunnel: w1552 -> [_ w1594 w1618 w1675 w1703]
                  tunnel: w1551 -> [_ w1603 w1623 w1684 w1700]
                  tunnel: w1550 -> [w1560 w1599 w1622 w1680 w1688]
                  tunnel: w1549 -> [_ _ _ _ w1714]
                  tunnel: w1548 -> [_ _ _ _ w1713]
                  tunnel: [w1558 w1579 w1612 w1663 w1691] -> w1547
                  tunnel: [w1559 FALSE FALSE FALSE FALSE] -> w1546
                  tunnel: w1545 -> [_ _ w1621 _ _]
                  frame "Stop", Default {
                    n591 = flat-sequence {
                      tunnel: w1560 -> [w1561]
                      tunnel: [TRUE] -> w1559
                      tunnel: [T16."Stop"] -> w1558
                      frame #0 {
                        n592 = call "TesterOption (SubVI).vi"("2 Options"=FALSE, "On/Off"=FALSE, "Tester Option"=T13."Venable", "VISA Refnum in"=w1561) -> ()  [unwired: 6 in, 2 out]
                      }
                      frame #1 {
                      }
                    }
                  }
                  frame "AO[1]=Meas." {
                    n593 = property on="AO[1]Meas" class="DigNum (strict)"() -> ("Value"=w1573:dbl)  [unwired: 2 in, 2 out]
                    n594 = Number To Fractional String(number=w1573) -> (F-format string=w1581:string)  [unwired: 3 in]
                    n595 = Search and Replace String(input string="EP=1\r\nAO[1]=0\r\n" ("write buffer"), search string="0", replace string=w1581) -> (result string=w1580:string)  [unwired: 5 in, 3 out]
                    n596 = call "SerialMarvinSendGet.vi"("Clear Log"=FALSE, "write buffer"=w1580, "VISA resource name"=w1603) -> ("error out"=w1598:errorcluster)  [unwired: 7 in, 1 out]
                    n597 = call "TesterOption (SubVI).vi"("2 Options"=FALSE, "error in (no error)"=w1598, "On/Off"=FALSE, "Tester Option"=T13."Power", "VISA Refnum in"=w1599) -> ("error out"=w1597:errorcluster, "VISA Refnum out"=w1584:refnum<visa-resource-name>)  [unwired: 5 in]
                    n598 = call "Write panel message (SubVI).vi"("Stop BurnIn"=w1592, 4:"rpm"=w1594, 5:"rpm"=FALSE ("rpm"), "PrintTime"=TRUE, "Stop"=w1593, "error in (no error)"=w1597, "Time to wait"=20.0, "Strin"="Temperature sensor calibration test in process...\nSet Parameters...", "String in"=w1590) -> ("error out"=w1585:errorcluster)  [unwired: 2 in]
                    n599 = call "TesterOption (SubVI).vi"("2 Options"=FALSE, "error in (no error)"=w1585, "On/Off"=FALSE, "Tester Option"=T13."Venable", "VISA Refnum in"=w1584) -> ("error out"=w1578:errorcluster)  [unwired: 5 in, 1 out]
                    n600 = flat-sequence {
                      tunnel: [T16."Stop"] -> w1579
                      tunnel: w1571 -> [_]
                      frame #0 {
                      }
                    }
                    n601 = In Range and Coerce(upper limit=0.1, x=w1573, lower limit=-0.1) -> (In Range?=w1568:bool)  [unwired: 1 out]
                    "SensCalResult" <- w1568
                    n602 = call "Find_Number_LineMARVIN.vi"("Test Paragraph"="Sensor Reading Analog Offset", "error in"=w1578, "TableIn"=w1570) -> ("error out"=w1572:errorcluster, "Line number"=w1576:i32)  [unwired: 2 in, 2 out]
                    n603 = call "PassOrFail (SubVI).vi"("Test#"="2", "index (row)"=w1576, "error in (no error)"=w1572, "Data in"=w1573, "Pass?Fail"=w1568, "Table in"=w1570) -> ("error out"=w1571:errorcluster)  [unwired: 5 in]
                  }
                  frame "TA[5]" {
                    w1624 = T19 [enum."50C", enum."80C", enum."100C", enum."120C"] items=["K15", "K16", "K17", "Venable", "Firmeware", "Fan", "Power", "120C", "110C", "100C", "90C", "80C", "70C", "60C", "50C", "40C", "30C", "25C", "20C", "10C", "0C"]
                    n604 = for {
                      tunnel: w1624 -> [w1639] mode=indexing
                      tunnel: w1623 -> [w1638]
                      tunnel: w1622 -> [w1637]
                      tunnel: w1621 -> [w1636]
                      tunnel: w1620 -> [w1635]
                      tunnel: w1611 -> [w1634]
                      tunnel: w1619 -> [w1633]
                      tunnel: w1618 -> [w1632]
                      tunnel: dbl[] [0.59774, 0.65238, 0.68545, 0.71584] -> [w1627] mode=indexing
                      tunnel: [w1626] -> w1607 mode=indexing
                      tunnel: [w1625] -> w1610
                      n605 = for {
                        N: 5 -> [_]
                        tunnel: w1639 -> [w1657]
                        tunnel: w1638 -> [w1656]
                        tunnel: w1637 -> [w1652]
                        tunnel: w1636 -> [w1650]
                        tunnel: w1635 -> [w1649]
                        tunnel: w1634 -> [w1648]
                        tunnel: w1633 -> [w1646]
                        tunnel: w1632 -> [w1643]
                        tunnel: [w1642] -> w1631 mode=indexing
                        tunnel: [w1641] -> w1625
                        n606 = call "TesterOption (SubVI).vi"("2 Options"=FALSE, "On/Off"=TRUE, "Tester Option"=w1657, "VISA Refnum in"=w1652) -> ("error out"=w1653:errorcluster)  [unwired: 6 in, 1 out]
                        n607 = call "Write panel message (SubVI).vi"("Stop BurnIn"=w1646, 4:"rpm"=w1643, 5:"rpm"=FALSE ("rpm"), "PrintTime"=FALSE, "Stop"=w1648, "error in (no error)"=w1653, "Time to wait"=1.0, "Strin"=w1650, "String in"=w1649) -> ("error out"=w1651:errorcluster)  [unwired: 2 in]
                        n608 = call "SerialMarvinSendGet.vi"("error in (no error)"=w1651, "write buffer"="TA[5]\r\n", "VISA resource name"=w1656) -> ("error out"=w1641:errorcluster, "read buffer"=w1654:string)  [unwired: 7 in]
                        n609 = Fract/Exp String To Number(string=w1654) -> (number=w1642:dbl)  [unwired: 3 in, 1 out]
                      }
                      n610 = Add Array Elements(numeric array=w1631) -> (sum=w1630:dbl)
                      n611 = Divide(x=w1630, y=5.0) -> (x/y=w1628:dbl)
                      n612 = Subtract(x=w1628, y=w1627) -> (x-y=w1626:dbl)
                    }
                    n613 = property class="Bool (strict)"(reference=w1611, error in=w1610) -> ("Value"=w1616:bool)  [unwired: 2 out]
                    n614 = Select(t=T16."Stop", s=w1616, f=T16."AO[1]=Meas.") -> (s? t:f=w1612:T16)
                    n615 = Array Size(array=w1607) -> (size(s)=w1606:i32)
                    n616 = Add Array Elements(numeric array=w1607) -> (sum=w1609:dbl)
                    n617 = Divide(x=w1609, y=w1606) -> (x/y=→"AO[1]Meas":dbl)
                  }
                  frame "AO[1]=0" {
                    n618 = call "SerialMarvinSendGet.vi"("write buffer"="EP=1\r\nAO[1]=0\r\n", "VISA resource name"=w1684) -> ("error out"=w1679:errorcluster)  [unwired: 8 in, 1 out]
                    n619 = call "TesterOption (SubVI).vi"("2 Options"=FALSE, "error in (no error)"=w1679, "On/Off"=FALSE, "Tester Option"=T13."Power", "VISA Refnum in"=w1680) -> ("error out"=w1678:errorcluster, "VISA Refnum out"=w1666:refnum<visa-resource-name>)  [unwired: 5 in]
                    n620 = call "Write panel message (SubVI).vi"("Stop BurnIn"=w1674, 4:"rpm"=w1675, 5:"rpm"=FALSE ("rpm"), "PrintTime"=TRUE, "Stop"=w1660, "error in (no error)"=w1678, "Time to wait"=20.0, "Strin"="Temperature sensor calibration test in process...\nSet Parameters...", "String in"=w1672) -> ("error out"=w1667:errorcluster)  [unwired: 2 in]
                    n621 = call "TesterOption (SubVI).vi"("2 Options"=FALSE, "error in (no error)"=w1667, "On/Off"=FALSE, "Tester Option"=T13."Venable", "VISA Refnum in"=w1666) -> ("error out"=w1661:errorcluster)  [unwired: 5 in, 1 out]
                    n622 = property class="Bool (strict)"(reference=w1660, error in=w1661) -> ("Value"=w1665:bool)  [unwired: 2 out]
                    n623 = Select(t=T16."Stop", s=w1665, f=T16."TA[5]") -> (s? t:f=w1663:T16)
                  }
                  frame "Start" {
                    n624 = call "Write panel message (SubVI).vi"("Stop BurnIn"=w1704, 4:"rpm"=w1703, 5:"rpm"=FALSE ("rpm"), "PrintTime"=FALSE, "Stop"=w1706, "Time to wait"=0.1, "Strin"="Temperature sensor calibration test in process...\nInitialization state...", "String in"=w1708) -> ("error out"=w1709:errorcluster)  [unwired: 3 in]
                    n625 = call "TesterOption (SubVI).vi"("2 Options"=FALSE, "error in (no error)"=w1709, "On/Off"=FALSE, "Tester Option"=T13."Venable", "VISA Refnum in"=w1688) -> ("error out"=w1711:errorcluster)  [unwired: 5 in, 1 out]
                    n626 = call "CANSendMotorSpeed.vi"("Remote"=TRUE, "error in (no error)"=w1711, "Motor Speed RPM"=u16 0, "UUT"=w1713, "CAN Cluster in"=w1714) -> ("error out"=w1698:errorcluster)  [unwired: 6 in]
                    n627 = call "SerialMarvinSendGet.vi"("error in (no error)"=w1698, "write buffer"="AO[1]\r\n", "VISA resource name"=w1700) -> ("error out"=w1687:errorcluster, "read buffer"=w1697:string)  [unwired: 7 in]
                    n628 = Equal?(x=w1697, y="0.0") -> (x = y?=w1689:bool)
                    n629 = property class="Bool (strict)"(reference=w1706, error in=w1687) -> ("Value"=w1718:bool)  [unwired: 2 out]
                    n630 = Select(t=T16."TA[5]", s=w1689, f=T16."AO[1]=0") -> (s? t:f=w1693:T16)
                    n631 = Select(t=T16."Stop", s=w1718, f=w1693) -> (s? t:f=w1691:T16)
                  }
                }
              }
            }
          }
        }
        frame "Auxiliary" {
          w1722 = "Auxiliary test in process..." ("Value")
          w1729 = "Auxiliary Fan Test" ("Test Paragraph")
          n632 = control-ref of="Pannel User Message"() -> (w1728:refnum<vi>)
          n633 = property class="Str"(reference=w1728, error in=w1725, "Value"=w1722) -> (error out=w1727:errorcluster)  [unwired: 1 out]
          n634 = call "Table_ScrollaBarMarvin.vi"("error in"=w1727, "Line to focus"=w1729, "reference in"=w1726) -> ("error out"=w1735:errorcluster)  [unwired: 2 out]
          n635 = property class="Tbl (strict)"(reference=w1726, error in=w1735) -> (reference out=w1724:refnum<vi>, error out=w1734:errorcluster, "Value"=w1733:string[][])
          n636 = Index Array(array=w1733, index (col)=1 ("disabled index (col)")) -> (element=w1732:string[])  [unwired: 1 in]
          n637 = property on="5.4.0" class="Bool (strict)"() -> ("Value"=w1719:bool)  [unwired: 2 in, 2 out]
          n638 = call "Find_Number_Line.vi"("error in"=w1734, "Test Paragraph"=w1729, "Row Headers[]"=w1732) -> ("error out"=w1730:errorcluster, "Line number"=w1721:i32)  [unwired: 1 out]
          n639 = call "Reset old test Values (SubVI).vi"("error in"=w1730, "Atr in"=w1724, "Test Paragraph"=w1729) -> ("error out"=w1723:errorcluster)  [unwired: 8 in]
          n640 = case shown="False" w1719 {
            tunnel: w1723 -> [w1745 w2126]
            tunnel: w1722 -> [w1740 w2121]
            tunnel: w1721 -> [w1738 w2119]
            tunnel: w1720 -> [w1736 w2117]
            frame True {
              n641 = property on="VISA Tester" class="VISAName"() -> ("Value"=w1739:refnum<visa-resource-name>)  [unwired: 2 in, 2 out]
              n642 = control-ref of="Stop Burn-in"() -> (w1742:refnum<vi>)
              n643 = control-ref of="Stop Button"() -> (w1743:refnum<vi>)
              n644 = control-ref of="Pannel User Message"() -> (w1744:refnum<vi>)
              n645 = control-ref of="ATR"() -> (w1737:refnum<vi>)
              n646 = control-ref of="Config_CANAT"() -> ()  [unwired: 1 out]
              n647 = control-ref of="Motor Speed RPM"() -> (w1741:refnum<vi>)
              n648 = while {
                shift-right: [w1752] -> _
                shift-left: enum16{"Stop", "CoolingON", "HotGunON", "Start"}."Start" -> [w1759]
                tunnel: w1745 -> [w1750]
                tunnel: w1744 -> [w1758]
                tunnel: w1743 -> [w1757]
                tunnel: w1742 -> [w1756]
                tunnel: w1741 -> [w1755]
                tunnel: w1740 -> [w1754]
                tunnel: w1739 -> [w1753]
                tunnel: w1738 -> [w1749]
                tunnel: w1737 -> [w1748]
                tunnel: w1736 -> [w1747]
                stop <- w1751 stop-if-true
                n649 = case shown="\"Start\"" w1759 {
                  tunnel: w1758 -> [_ w1805 w1900 w1952]
                  tunnel: w1757 -> [_ w1800 w1895 w1950]
                  tunnel: w1756 -> [_ w1804 w1899 w1951]
                  tunnel: w1755 -> [_ w1803 w1898 w1948]
                  tunnel: w1754 -> [_ w1794 w1889 w1949]
                  tunnel: w1753 -> [_ w1795 w1890 w1946]
                  tunnel: [w1761 w1797 w1892 w1941] -> w1752
                  tunnel: [w1760 FALSE FALSE FALSE] -> w1751
                  tunnel: w1750 -> [_ w1793 w1888 _]
                  tunnel: w1749 -> [_ w1788 w1883 w1942]
                  tunnel: w1748 -> [_ w1784 w1880 w1944]
                  tunnel: w1747 -> [_ _ _ w1953]
                  frame "Stop", Default {
                    n650 = flat-sequence {
                      tunnel: [enum16{"Stop", "CoolingON", "HotGunON", "Start"}."Stop"] -> w1761
                      tunnel: [TRUE] -> w1760
                      frame #0 {
                        n651 = property on="VISA Tester" class="VISAName"() -> ("Value"=w1765:refnum<visa-resource-name>)  [unwired: 2 in, 2 out]
                        n652 = call "TesterOption (SubVI).vi"("2 Options"=FALSE, "On/Off"=FALSE, "Tester Option"=T13."Venable", "VISA Refnum in"=w1765) -> ()  [unwired: 6 in, 2 out]
                      }
                      frame #1 {
                      }
                    }
                  }
                  frame "CoolingON" {
                    n653 = while {
                      tunnel: w1805 -> [w1840]
                      tunnel: w1804 -> [w1839]
                      tunnel: w1803 -> [w1835]
                      tunnel: [w1832] -> w1773
                      tunnel: w1800 -> [w1823]
                      tunnel: w1795 -> [w1809]
                      tunnel: w1794 -> [w1827]
                      tunnel: w1793 -> [w1824]
                      shift-right: [w1816] -> w1768
                      shift-left: 0.0 -> [w1817]
                      shift-right: [w1812] -> w1772
                      shift-left: 0.0 ("Value") -> [w1814]
                      tunnel: [w1807] -> w1776
                      stop <- w1821 stop-if-true
                      n654 = control-ref of="Power transistor Heat sink Temp."() -> (w1833:refnum<vi>)
                      n655 = property class="DigNum (strict)"(reference=w1833, error in=w1824) -> (error out=w1830:errorcluster, "Value"=w1812:dbl)  [unwired: 1 out]
                      n656 = Equal?(x=w1812, y=w1814) -> (x = y?=w1813:bool)
                      n657 = Number To Fractional String(number=w1812, precision (6)=i16 2) -> (F-format string=w1826:string)  [unwired: 2 in]
                      n658 = case shown="True" w1813 {
                        tunnel: w1817 -> [_ w1860]
                        tunnel: [0.0 w1858] -> w1816
                        tunnel: [FALSE w1857] -> w1815
                        frame False {
                        }
                        frame True {
                          n659 = Increment(x=w1860) -> (x+1=w1858:dbl)
                          n660 = Greater Or Equal?(x=w1858, y=300.0) -> (x >= y?=w1857:bool)
                        }
                      }
                      n661 = Concatenate Strings(w1827, "\nPCB Temperature [C]: " ("string"), w1826) -> (w1825:string)
                      n662 = call "Write panel message (SubVI).vi"("Stop BurnIn"=w1839, 4:"rpm"=w1835, 5:"rpm"=FALSE ("rpm"), "PrintTime"=FALSE, "Stop"=w1823, "error in (no error)"=w1830, "Time to wait"=0.2, "Strin"=w1825, "String in"=w1840) -> ("error out"=w1829:errorcluster)  [unwired: 2 in]
                      n663 = property class="Bool (strict)"(reference=w1823) -> ("Value"=w1822:bool)  [unwired: 1 in, 2 out]
                      n664 = Less Or Equal?(x=w1812, y=52.0) -> (x <= y?=w1811:bool)
                      n665 = call "GetADCTester (SubVI).vi"("error in (no error)"=w1829, "GetADCTester"=T15."Fan", "VISA Refnum in"=w1809) -> ("error out"=w1832:errorcluster, "ADCValOutput Single"=w1819:dbl)  [unwired: 6 in, 1 out]
                      n666 = Greater?(x=w1819, y=u32 2400) -> (0:w1808:bool)
                      n667 = case shown="True" w1811 {
                        tunnel: [w1847 w1854] -> w1810
                        tunnel: w1811 -> [w1847 w1854]
                        tunnel: w1809 -> [w1845 w1852]
                        tunnel: [w1841 w1848] -> w1807
                        frame False {
                          n668 = call "Time Delay11"() -> ("error out"=w1844:errorcluster)  [unwired: 11 in]
                          n669 = call "GetADCTester (SubVI).vi"("error in (no error)"=w1844, "GetADCTester"=T15."Fan", "VISA Refnum in"=w1845) -> ("ADCValOutput Single"=w1843:dbl)  [unwired: 6 in, 2 out]
                          n670 = Greater?(x=w1843, y=2400.0) -> (0:w1841:bool)
                        }
                        frame True {
                          n671 = call "Time Delay10"() -> ("error out"=w1851:errorcluster)  [unwired: 11 in]
                          n672 = call "GetADCTester (SubVI).vi"("error in (no error)"=w1851, "GetADCTester"=T15."Fan", "VISA Refnum in"=w1852) -> ("ADCValOutput Single"=w1850:dbl)  [unwired: 6 in, 2 out]
                          n673 = Greater?(x=w1850, y=2400.0) -> (0:w1848:bool)
                        }
                      }
                      n674 = Compound Arithmetic op=OR(w1808, w1822, w1810, w1815) -> (w1821:bool)
                    }
                    "Numeric" <- w1768
                    n675 = In Range and Coerce(upper limit=58.0, x=w1772, lower limit=52.0) -> (In Range?=w1775:bool)  [unwired: 1 out]
                    n676 = Build Array(w1776, w1775) -> (w1777:bool[])
                    n677 = And Array Elements(Boolean array=w1777) -> (logical AND=→"AuxiOFFResult":bool)
                    n678 = Add(x=w1788, y=3) -> (x+y=w1786:i32)
                    n679 = call "PassOrFail (SubVI).vi"("index (row)"=w1786, "error in (no error)"=w1773, "Data in"=w1772, "Pass?Fail"=w1775, "Table in"=w1784) -> ("error out"=w1790:errorcluster)  [unwired: 6 in]
                    n680 = Select(t="OFF", s=w1776, f="ON") -> (s? t:f=w1780:string)
                    n681 = Increment(x=w1786) -> (x+1=w1785:i32)
                    n682 = call "PassOrFail (SubVI).vi"("String Res"=w1780, "index (row)"=w1785, "error in (no error)"=w1790, "Data in"=-3.0, "Pass?Fail"=w1776, "Table in"=w1784) -> ("error out"=w1789:errorcluster)  [unwired: 5 in]
                    n683 = call "TesterOption (SubVI).vi"("2 Options"=FALSE, "error in (no error)"=w1789, "On/Off"=FALSE, "Tester Option"=T13."Venable" ("Tester Option 2"), "VISA Refnum in"=w1795) -> ("error out"=w1770:errorcluster)  [unwired: 5 in, 1 out]
                    n684 = call "Time Delay14"("error in (no error)"=w1770) -> ("error out"=w1769:errorcluster)  [unwired: 10 in]
                    n685 = property class="Bool (strict)"(reference=w1800, error in=w1769) -> ("Value"=w1806:bool)  [unwired: 2 out]
                    n686 = Select(t=enum16{"Stop", "CoolingON", "HotGunON", "Start"}."Stop", s=w1806, f=enum16{"Stop", "CoolingON", "HotGunON", "Start"}."Stop") -> (s? t:f=w1797:enum16{"Stop", "CoolingON", "HotGunON", "Start"})
                  }
                  frame "HotGunON" {
                    n687 = while {
                      tunnel: w1900 -> [w1933]
                      tunnel: w1899 -> [w1932]
                      tunnel: w1898 -> [w1928]
                      tunnel: [w1924] -> w1870
                      tunnel: w1895 -> [w1915]
                      tunnel: w1890 -> [w1925]
                      tunnel: w1889 -> [w1919]
                      tunnel: w1888 -> [w1916]
                      shift-right: [w1908] -> _
                      shift-left: 0.0 -> [w1909]
                      shift-right: [w1905] -> _
                      shift-left: 0.0 ("Value") -> [w1906]
                      tunnel: [w1903] -> w1868
                      stop <- w1913 stop-if-true
                      n688 = control-ref of="Power transistor Heat sink Temp."() -> (w1926:refnum<vi>)
                      n689 = property class="DigNum (strict)"(reference=w1926, error in=w1916) -> (error out=w1922:errorcluster, "Value"=w1905:dbl)  [unwired: 1 out]
                      n690 = Equal?(x=w1905, y=w1906) -> (x = y?=w1904:bool)
                      n691 = Number To Fractional String(number=w1905, precision (6)=i16 2) -> (F-format string=w1918:string)  [unwired: 2 in]
                      n692 = case shown="True" w1904 {
                        tunnel: w1909 -> [_ w1939]
                        tunnel: [0.0 w1937] -> w1908
                        tunnel: [FALSE w1936] -> w1907
                        frame False {
                        }
                        frame True {
                          n693 = Increment(x=w1939) -> (x+1=w1937:dbl)
                          n694 = Greater Or Equal?(x=w1937, y=300.0) -> (x >= y?=w1936:bool)
                        }
                      }
                      n695 = Concatenate Strings(w1919, "\nPCB Temperature [C]: " ("string"), w1918) -> (w1917:string)
                      n696 = call "Write panel message (SubVI).vi"("Stop BurnIn"=w1932, 4:"rpm"=w1928, 5:"rpm"=FALSE ("rpm"), "PrintTime"=FALSE, "Stop"=w1915, "error in (no error)"=w1922, "Time to wait"=0.2, "Strin"=w1917, "String in"=w1933) -> ("error out"=w1921:errorcluster)  [unwired: 2 in]
                      n697 = property class="Bool (strict)"(reference=w1915) -> ("Value"=w1914:bool)  [unwired: 1 in, 2 out]
                      n698 = call "GetADCTester (SubVI).vi"("error in (no error)"=w1921, "GetADCTester"=T15."Fan", "VISA Refnum in"=w1925) -> ("error out"=w1924:errorcluster, "ADCValOutput Single"=w1911:dbl)  [unwired: 6 in, 1 out]
                      n699 = Greater Or Equal?(x=w1905, y=61.0) -> (x >= y?=w1902:bool)
                      n700 = Less?(x=w1911, y=u32 100) -> (x < y?=w1903:bool)
                      n701 = Compound Arithmetic op=OR(w1903, w1914, w1902, w1907) -> (w1913:bool)
                    }
                    n702 = control-ref of="Power transistor Heat sink Temp."() -> (w1873:refnum<vi>)
                    n703 = property class="DigNum (strict)"(reference=w1873, error in=w1870) -> (error out=w1872:errorcluster, "Value"=w1871:dbl)  [unwired: 1 out]
                    n704 = In Range and Coerce(upper limit=62.0, x=w1871, lower limit=58.0) -> (In Range?=w1867:bool)  [unwired: 1 out]
                    n705 = Build Array(w1868, w1867) -> (w1869:bool[])
                    n706 = Increment(x=w1883) -> (x+1=w1882:i32)
                    n707 = call "PassOrFail (SubVI).vi"("index (row)"=w1882, "error in (no error)"=w1872, "Data in"=w1871, "Pass?Fail"=w1867, "Table in"=w1880) -> ("error out"=w1885:errorcluster)  [unwired: 6 in]
                    n708 = And Array Elements(Boolean array=w1869) -> (logical AND=→"AuxiONResult":bool)
                    n709 = Increment(x=w1882) -> (x+1=w1881:i32)
                    n710 = Select(t="ON", s=w1868, f="OFF") -> (s? t:f=w1878:string)
                    n711 = call "PassOrFail (SubVI).vi"("String Res"=w1878, "index (row)"=w1881, "error in (no error)"=w1885, "Data in"=-3.0, "Pass?Fail"=w1868, "Table in"=w1880) -> ("error out"=w1884:errorcluster)  [unwired: 5 in]
                    n712 = call "TesterOption (SubVI).vi"("On/Off 2"=FALSE, "Tester Option 2"=T13."Venable", "2 Options"=TRUE, "error in (no error)"=w1884, "On/Off"=FALSE, "Tester Option"=T13."Fan", "VISA Refnum in"=w1890) -> ("error out"=w1862:errorcluster)  [unwired: 3 in, 1 out]
                    n713 = call "Time Delay13"("error in (no error)"=w1862) -> ("error out"=w1861:errorcluster)  [unwired: 10 in]
                    n714 = property class="Bool (strict)"(reference=w1895, error in=w1861) -> ("Value"=w1901:bool)  [unwired: 2 out]
                    n715 = Select(t=enum16{"Stop", "CoolingON", "HotGunON", "Start"}."Stop", s=w1901, f=enum16{"Stop", "CoolingON", "HotGunON", "Start"}."CoolingON") -> (s? t:f=w1892:enum16{"Stop", "CoolingON", "HotGunON", "Start"})
                  }
                  frame "Start" {
                    n716 = call "Write panel message (SubVI).vi"("Stop BurnIn"=w1951, 4:"rpm"=w1948, 5:"rpm"=FALSE ("rpm"), "PrintTime"=FALSE, "Stop"=w1950, "Time to wait"=1.0, "Strin"=w1949, "String in"=w1952) -> ("error out"=w1959:errorcluster)  [unwired: 3 in]
                    n717 = call "TesterOption (SubVI).vi"("2 Options"=FALSE, "error in (no error)"=w1959, "On/Off"=FALSE, "Tester Option"=T13."Venable", "VISA Refnum in"=w1946) -> ("error out"=w1954:errorcluster)  [unwired: 5 in, 1 out]
                    n718 = while {
                      tunnel: w1954 -> [w1980]
                      tunnel: w1953 -> [w1979]
                      tunnel: w1952 -> [w1978]
                      tunnel: w1951 -> [w1977]
                      tunnel: w1950 -> [w1976]
                      tunnel: w1949 -> [w1975]
                      tunnel: w1948 -> [w1974]
                      shift-right: [w1971] -> _
                      shift-left: enum16{"Wait", "OFF", "ON", "Start"}."Start" -> [w1973]
                      tunnel: w1946 -> [w1972]
                      shift-right: [w1969] -> _
                      shift-left: 0 -> [w1970]
                      tunnel: w1944 -> [w1967]
                      shift-right: [w1966] -> w1940
                      shift-left: TRUE -> [w1965]
                      tunnel: w1942 -> [w1964]
                      stop <- w1968 stop-if-true
                      n719 = case shown="\"Start\"" w1973 {
                        tunnel: w1980 -> [_ w2027 _ w2092]
                        tunnel: w1979 -> [w1995 w2026 _ w2091]
                        tunnel: w1978 -> [_ w2024 _ w2089]
                        tunnel: w1977 -> [_ w2023 _ w2088]
                        tunnel: w1976 -> [_ w2002 _ w2074]
                        tunnel: w1975 -> [_ w2022 _ w2087]
                        tunnel: w1974 -> [_ w2021 _ w2086]
                        tunnel: w1972 -> [_ w2014 _ w2080]
                        tunnel: [w1998 w2004 enum16{"Wait", "OFF", "ON", "Start"}."OFF" w2071] -> w1971
                        tunnel: w1970 -> [w1999 w2012 _ w2079]
                        tunnel: [w1999 w2011 0 w2078] -> w1969
                        tunnel: [w1997 FALSE FALSE FALSE] -> w1968
                        tunnel: w1967 -> [w1983 _ w2063 _]
                        tunnel: [FALSE w2008 TRUE w2075] -> w1966
                        tunnel: w1965 -> [w1986 _ w2064 _]
                        tunnel: w1964 -> [w1985 _ w2062 _]
                        frame "Wait", Default {
                          n720 = call "SerialMarvinSendGet.vi"("write buffer"="EP=1\r\nAU=0\r\n", "VISA resource name"=w1995) -> ("error out"=w1994:errorcluster)  [unwired: 8 in, 1 out]
                          n721 = call "Time Delay19"("error in (no error)"=w1994) -> ("error out"=w1982:errorcluster)  [unwired: 10 in]
                          n722 = Not(x=w1986) -> (.not. x?=w1988:bool)
                          n723 = Select(t="OFF", s=w1988, f="ON") -> (s? t:f=w1987:string)
                          n724 = Add(x=2, y=w1985) -> (x+y=w1992:i32)
                          n725 = call "PassOrFail (SubVI).vi"("String Res"=w1987, "index (row)"=w1992, "error in (no error)"=w1982, "Data in"=-3.0, "Pass?Fail"=w1988, "Table in"=w1983) -> ("error out"=w1981:errorcluster)  [unwired: 5 in]
                          n726 = flat-sequence {
                            tunnel: [enum16{"Wait", "OFF", "ON", "Start"}."Wait"] -> w1998
                            tunnel: [TRUE] -> w1997
                            tunnel: w1981 -> [_]
                            frame #0 {
                            }
                          }
                        }
                        frame "OFF" {
                          n727 = call "SerialMarvinSendGet.vi"("error in (no error)"=w2027, "write buffer"="EP=1\r\nAU=0\r\n", "VISA resource name"=w2026) -> ("error out"=w2016:errorcluster)  [unwired: 7 in, 1 out]
                          n728 = call "Time Delay"("error in (no error)"=w2016) -> ("error out"=w2010:errorcluster)  [unwired: 10 in]
                          n729 = call "GetADCTester (SubVI).vi"("error in (no error)"=w2010, "GetADCTester"=T15."Fan", "TimeToGet"=5, "VISA Refnum in"=w2014) -> ("error out"=w2015:errorcluster, "ADCValOutput Single"=w2018:dbl)  [unwired: 5 in, 1 out]
                          n730 = Greater?(x=w2018, y=2400.0) -> (0:w2013:bool)
                          n731 = case shown="True" w2013 {
                            tunnel: w2024 -> [_ w2046]
                            tunnel: w2023 -> [_ w2045]
                            tunnel: w2002 -> [_ w2044]
                            tunnel: w2022 -> [_ w2043]
                            tunnel: w2021 -> [_ w2042]
                            tunnel: w2015 -> [w2029 w2041]
                            tunnel: [w2030 w2039] -> w2003
                            tunnel: w2012 -> [w2034 _]
                            tunnel: [w2035 0] -> w2011
                            tunnel: [w2029 w2037] -> w2005
                            tunnel: [w2028 FALSE] -> w2008
                            frame False {
                              n732 = Increment(x=w2034) -> (x+1=w2035:i32)
                              n733 = Greater Or Equal?(x=w2034, y=10) -> (x >= y?=w2028:bool)
                              n734 = Select(t=enum16{"Wait", "OFF", "ON", "Start"}."Wait", s=w2028, f=enum16{"Wait", "OFF", "ON", "Start"}."OFF") -> (s? t:f=w2030:enum16{"Wait", "OFF", "ON", "Start"})
                            }
                            frame True {
                              n735 = call "Write panel message (SubVI).vi"("Stop BurnIn"=w2045, 4:"rpm"=w2042, 5:"rpm"=FALSE ("rpm"), "PrintTime"=TRUE, "Stop"=w2044, "error in (no error)"=w2041, "Time to wait"=5.0, "Strin"=w2043, "String in"=w2046) -> ("error out"=w2040:errorcluster)  [unwired: 2 in]
                              n736 = flat-sequence {
                                tunnel: w2040 -> [w2050]
                                tunnel: [enum16{"Wait", "OFF", "ON", "Start"}."Wait"] -> w2039
                                tunnel: [w2050] -> w2037
                                frame #0 {
                                }
                              }
                            }
                          }
                          n737 = property class="Bool (strict)"(reference=w2002, error in=w2005) -> ("Value"=w2007:bool)  [unwired: 2 out]
                          n738 = Select(t=enum16{"Wait", "OFF", "ON", "Start"}."Wait", s=w2007, f=w2003) -> (s? t:f=w2004:enum16{"Wait", "OFF", "ON", "Start"})
                        }
                        frame "ON" {
                          n739 = Not(x=w2064) -> (.not. x?=w2057:bool)
                          n740 = Select(t="ON", s=w2057, f="OFF") -> (s? t:f=w2056:string)
                          n741 = Increment(x=w2062) -> (x+1=w2061:i32)
                          n742 = call "PassOrFail (SubVI).vi"("String Res"=w2056, "index (row)"=w2061, "Data in"=-3.0, "Pass?Fail"=w2057, "Table in"=w2063) -> ()  [unwired: 6 in, 1 out]
                        }
                        frame "Start" {
                          n743 = call "SerialMarvinSendGet.vi"("error in (no error)"=w2092, "write buffer"="EP=1\r\nAU=1\r\n", "VISA resource name"=w2091) -> ("error out"=w2082:errorcluster)  [unwired: 7 in, 1 out]
                          n744 = call "Time Delay18"("error in (no error)"=w2082) -> ("error out"=w2077:errorcluster)  [unwired: 10 in]
                          n745 = call "GetADCTester (SubVI).vi"("error in (no error)"=w2077, "GetADCTester"=T15."Fan", "TimeToGet"=10, "VISA Refnum in"=w2080) -> ("error out"=w2081:errorcluster, "ADCValOutput Single"=w2065:dbl)  [unwired: 5 in, 1 out]
                          "ADCValOutput Single" <- w2065
                          n746 = Not Equal To 0?(x=w2065) -> (x != 0?=w2066:bool)
                          n747 = Less?(x=w2065, y=200.0) -> (x < y?=w2068:bool)
                          n748 = And(x=w2068, y=w2066) -> (x .and. y?=w2067:bool)
                          n749 = case shown="False" w2067 {
                            tunnel: w2089 -> [_ w2111]
                            tunnel: w2088 -> [_ w2110]
                            tunnel: w2074 -> [_ w2109]
                            tunnel: w2087 -> [_ w2108]
                            tunnel: w2086 -> [_ w2107]
                            tunnel: w2081 -> [w2094 w2106]
                            tunnel: [w2095 w2104] -> w2072
                            tunnel: w2079 -> [w2099 _]
                            tunnel: [w2100 0] -> w2078
                            tunnel: [w2094 w2102] -> w2069
                            tunnel: [w2093 FALSE] -> w2075
                            frame False {
                              n750 = Increment(x=w2099) -> (x+1=w2100:i32)
                              n751 = Greater Or Equal?(x=w2099, y=5) -> (x >= y?=w2093:bool)
                              n752 = Select(t=enum16{"Wait", "OFF", "ON", "Start"}."ON", s=w2093, f=enum16{"Wait", "OFF", "ON", "Start"}."Start") -> (s? t:f=w2095:enum16{"Wait", "OFF", "ON", "Start"})
                            }
                            frame True {
                              n753 = call "Write panel message (SubVI).vi"("Stop BurnIn"=w2110, 4:"rpm"=w2107, 5:"rpm"=FALSE ("rpm"), "PrintTime"=TRUE, "Stop"=w2109, "error in (no error)"=w2106, "Time to wait"=10.0, "Strin"=w2108, "String in"=w2111) -> ("error out"=w2105:errorcluster)  [unwired: 2 in]
                              n754 = flat-sequence {
                                tunnel: w2105 -> [w2115]
                                tunnel: [enum16{"Wait", "OFF", "ON", "Start"}."ON"] -> w2104
                                tunnel: [w2115] -> w2102
                                frame #0 {
                                }
                              }
                            }
                          }
                          n755 = property class="Bool (strict)"(reference=w2074, error in=w2069) -> ("Value"=w2073:bool)  [unwired: 2 out]
                          n756 = Select(t=enum16{"Wait", "OFF", "ON", "Start"}."Wait", s=w2073, f=w2072) -> (s? t:f=w2071:enum16{"Wait", "OFF", "ON", "Start"})
                        }
                      }
                    }
                    n757 = flat-sequence {
                      tunnel: [enum16{"Stop", "CoolingON", "HotGunON", "Start"}."Stop"] -> w1941
                      tunnel: w1940 -> [_]
                      frame #0 {
                      }
                    }
                  }
                }
              }
            }
            frame False {
              n758 = property on="VISA Tester" class="VISAName"() -> ("Value"=w2120:refnum<visa-resource-name>)  [unwired: 2 in, 2 out]
              n759 = control-ref of="Stop Burn-in"() -> (w2123:refnum<vi>)
              n760 = control-ref of="Stop Button"() -> (w2124:refnum<vi>)
              n761 = control-ref of="Pannel User Message"() -> (w2125:refnum<vi>)
              n762 = control-ref of="ATR"() -> (w2118:refnum<vi>)
              n763 = control-ref of="Config_CANAT"() -> ()  [unwired: 1 out]
              n764 = control-ref of="Motor Speed RPM"() -> (w2122:refnum<vi>)
              n765 = while {
                shift-right: [w2133] -> _
                shift-left: enum16{"Stop", "CoolingON", "HotGunON", "Start"}."Start" -> [w2140]
                tunnel: w2126 -> [w2131]
                tunnel: w2125 -> [w2139]
                tunnel: w2124 -> [w2138]
                tunnel: w2123 -> [w2137]
                tunnel: w2122 -> [w2136]
                tunnel: w2121 -> [w2135]
                tunnel: w2120 -> [w2134]
                tunnel: w2119 -> [w2130]
                tunnel: w2118 -> [w2129]
                tunnel: w2117 -> [w2128]
                stop <- w2132 stop-if-true
                n766 = case shown="\"CoolingON\"" w2140 {
                  tunnel: w2139 -> [_ w2186 w2282 w2333]
                  tunnel: w2138 -> [_ w2181 w2277 w2331]
                  tunnel: w2137 -> [_ w2185 w2281 w2332]
                  tunnel: w2136 -> [_ w2184 w2280 w2329]
                  tunnel: w2135 -> [_ w2175 w2271 w2330]
                  tunnel: w2134 -> [_ w2176 w2272 w2328]
                  tunnel: [w2142 w2178 w2274 w2325] -> w2133
                  tunnel: [w2141 FALSE FALSE FALSE] -> w2132
                  tunnel: w2131 -> [_ w2174 w2270 _]
                  tunnel: w2130 -> [_ w2169 w2265 w2326]
                  tunnel: w2129 -> [_ w2165 w2262 w2327]
                  tunnel: w2128 -> [_ _ _ w2334]
                  frame "Stop", Default {
                    n767 = flat-sequence {
                      tunnel: [enum16{"Stop", "CoolingON", "HotGunON", "Start"}."Stop"] -> w2142
                      tunnel: [TRUE] -> w2141
                      frame #0 {
                        n768 = property on="VISA Tester" class="VISAName"() -> ("Value"=w2146:refnum<visa-resource-name>)  [unwired: 2 in, 2 out]
                        n769 = call "TesterOption (SubVI).vi"("2 Options"=FALSE, "On/Off"=FALSE, "Tester Option"=T13."Venable", "VISA Refnum in"=w2146) -> ()  [unwired: 6 in, 2 out]
                      }
                      frame #1 {
                      }
                    }
                  }
                  frame "CoolingON" {
                    n770 = while {
                      tunnel: w2186 -> [w2222]
                      tunnel: w2185 -> [w2221]
                      tunnel: w2184 -> [w2217]
                      tunnel: [w2214] -> w2154
                      tunnel: w2181 -> [w2205]
                      tunnel: w2176 -> [w2191]
                      tunnel: w2175 -> [w2209]
                      tunnel: w2174 -> [w2206]
                      shift-right: [w2198] -> w2149
                      shift-left: 0.0 -> [w2199]
                      shift-right: [w2194] -> w2153
                      shift-left: 0.0 ("Value") -> [w2196]
                      tunnel: [w2188] -> w2157
                      stop <- w2203 stop-if-true
                      n771 = control-ref of="Power transistor Heat sink Temp."() -> (w2215:refnum<vi>)
                      n772 = property class="DigNum (strict)"(reference=w2215, error in=w2206) -> (error out=w2212:errorcluster, "Value"=w2194:dbl)  [unwired: 1 out]
                      n773 = Equal?(x=w2194, y=w2196) -> (x = y?=w2195:bool)
                      n774 = Number To Fractional String(number=w2194, precision (6)=i16 2) -> (F-format string=w2208:string)  [unwired: 2 in]
                      n775 = case shown="True" w2195 {
                        tunnel: w2199 -> [_ w2242]
                        tunnel: [0.0 w2240] -> w2198
                        tunnel: [FALSE w2239] -> w2197
                        frame False {
                        }
                        frame True {
                          n776 = Increment(x=w2242) -> (x+1=w2240:dbl)
                          n777 = Greater Or Equal?(x=w2240, y=300.0) -> (x >= y?=w2239:bool)
                        }
                      }
                      n778 = Concatenate Strings(w2209, "\nPCB Temperature [C]: " ("string"), w2208) -> (w2207:string)
                      n779 = call "Write panel message (SubVI).vi"("Stop BurnIn"=w2221, 4:"rpm"=w2217, 5:"rpm"=FALSE ("rpm"), "PrintTime"=FALSE, "Stop"=w2205, "error in (no error)"=w2212, "Time to wait"=0.2, "Strin"=w2207, "String in"=w2222) -> ("error out"=w2211:errorcluster)  [unwired: 2 in]
                      n780 = property class="Bool (strict)"(reference=w2205) -> ("Value"=w2204:bool)  [unwired: 1 in, 2 out]
                      n781 = Less Or Equal?(x=w2194, y=52.0) -> (x <= y?=w2193:bool)
                      n782 = call "GetADCTester (SubVI).vi"("error in (no error)"=w2211, "GetADCTester"=T15."Fan", "VISA Refnum in"=w2191) -> ("error out"=w2214:errorcluster, "ADCValOutput Single"=w2201:dbl)  [unwired: 6 in, 1 out]
                      n783 = Greater?(x=w2201, y=u32 2100) -> (0:w2189:bool)
                      n784 = case shown="True" w2193 {
                        tunnel: [w2229 w2236] -> w2192
                        tunnel: w2193 -> [w2229 w2236]
                        tunnel: w2191 -> [w2227 w2234]
                        tunnel: [w2223 w2230] -> w2190
                        frame False {
                          n785 = call "Time Delay20"() -> ("error out"=w2226:errorcluster)  [unwired: 11 in]
                          n786 = call "GetADCTester (SubVI).vi"("error in (no error)"=w2226, "GetADCTester"=T15."Fan", "VISA Refnum in"=w2227) -> ("ADCValOutput Single"=w2225:dbl)  [unwired: 6 in, 2 out]
                          n787 = Greater?(x=w2225, y=2100.0) -> (0:w2223:bool)
                        }
                        frame True {
                          n788 = call "Time Delay21"() -> ("error out"=w2233:errorcluster)  [unwired: 11 in]
                          n789 = call "GetADCTester (SubVI).vi"("error in (no error)"=w2233, "GetADCTester"=T15."Fan", "VISA Refnum in"=w2234) -> ("ADCValOutput Single"=w2232:dbl)  [unwired: 6 in, 2 out]
                          n790 = Greater?(x=w2232, y=2100.0) -> (0:w2230:bool)
                        }
                      }
                      n791 = Compound Arithmetic op=OR(w2189, w2204, w2192, w2197) -> (w2203:bool)
                      n792 = Or(x=w2189, y=w2190) -> (x .or. y?=w2188:bool)
                    }
                    "Numeric 2" <- w2149
                    n793 = In Range and Coerce(upper limit=58.0, x=w2153, lower limit=52.0) -> (In Range?=w2156:bool)  [unwired: 1 out]
                    n794 = Build Array(w2157, w2156) -> (w2158:bool[])
                    n795 = And Array Elements(Boolean array=w2158) -> (logical AND=→"AuxiOFFResult 2":bool)
                    n796 = Add(x=w2169, y=3) -> (x+y=w2167:i32)
                    n797 = call "PassOrFail (SubVI).vi"("index (row)"=w2167, "error in (no error)"=w2154, "Data in"=w2153, "Pass?Fail"=w2156, "Table in"=w2165) -> ("error out"=w2171:errorcluster)  [unwired: 6 in]
                    n798 = Select(t="OFF", s=w2157, f="ON") -> (s? t:f=w2161:string)
                    n799 = Increment(x=w2167) -> (x+1=w2166:i32)
                    n800 = call "PassOrFail (SubVI).vi"("String Res"=w2161, "index (row)"=w2166, "error in (no error)"=w2171, "Data in"=-3.0, "Pass?Fail"=w2157, "Table in"=w2165) -> ("error out"=w2170:errorcluster)  [unwired: 5 in]
                    n801 = call "TesterOption (SubVI).vi"("2 Options"=FALSE, "error in (no error)"=w2170, "On/Off"=FALSE, "Tester Option"=T13."Venable" ("Tester Option 2"), "VISA Refnum in"=w2176) -> ("error out"=w2151:errorcluster)  [unwired: 5 in, 1 out]
                    n802 = call "Time Delay22"("error in (no error)"=w2151) -> ("error out"=w2150:errorcluster)  [unwired: 10 in]
                    n803 = property class="Bool (strict)"(reference=w2181, error in=w2150) -> ("Value"=w2187:bool)  [unwired: 2 out]
                    n804 = Select(t=enum16{"Stop", "CoolingON", "HotGunON", "Start"}."Stop", s=w2187, f=enum16{"Stop", "CoolingON", "HotGunON", "Start"}."Stop") -> (s? t:f=w2178:enum16{"Stop", "CoolingON", "HotGunON", "Start"})
                  }
                  frame "HotGunON" {
                    n805 = while {
                      tunnel: w2282 -> [w2315]
                      tunnel: w2281 -> [w2314]
                      tunnel: w2280 -> [w2310]
                      tunnel: [w2306] -> w2252
                      tunnel: w2277 -> [w2297]
                      tunnel: w2272 -> [w2307]
                      tunnel: w2271 -> [w2301]
                      tunnel: w2270 -> [w2298]
                      shift-right: [w2292] -> _
                      shift-left: 0.0 -> [w2293]
                      shift-right: [w2289] -> _
                      shift-left: 0.0 ("Value") -> [w2290]
                      tunnel: [w2284] -> w2250
                      stop <- w2295 stop-if-true
                      n806 = control-ref of="Power transistor Heat sink Temp."() -> (w2308:refnum<vi>)
                      n807 = property class="DigNum (strict)"(reference=w2308, error in=w2298) -> (error out=w2304:errorcluster, "Value"=w2289:dbl)  [unwired: 1 out]
                      n808 = Equal?(x=w2289, y=w2290) -> (x = y?=w2288:bool)
                      n809 = Number To Fractional String(number=w2289, precision (6)=i16 2) -> (F-format string=w2300:string)  [unwired: 2 in]
                      n810 = case shown="True" w2288 {
                        tunnel: w2293 -> [_ w2321]
                        tunnel: [0.0 w2319] -> w2292
                        tunnel: [FALSE w2318] -> w2291
                        frame False {
                        }
                        frame True {
                          n811 = Increment(x=w2321) -> (x+1=w2319:dbl)
                          n812 = Greater Or Equal?(x=w2319, y=300.0) -> (x >= y?=w2318:bool)
                        }
                      }
                      n813 = Concatenate Strings(w2301, "\nPCB Temperature [C]: " ("string"), w2300) -> (w2299:string)
                      n814 = call "Write panel message (SubVI).vi"("Stop BurnIn"=w2314, 4:"rpm"=w2310, 5:"rpm"=FALSE ("rpm"), "PrintTime"=FALSE, "Stop"=w2297, "error in (no error)"=w2304, "Time to wait"=0.2, "Strin"=w2299, "String in"=w2315) -> ("error out"=w2303:errorcluster)  [unwired: 2 in]
                      n815 = property class="Bool (strict)"(reference=w2297) -> ("Value"=w2296:bool)  [unwired: 1 in, 2 out]
                      n816 = call "GetADCTester (SubVI).vi"("error in (no error)"=w2303, "GetADCTester"=T15."Fan", "VISA Refnum in"=w2307) -> ("error out"=w2306:errorcluster, "ADCValOutput Single"=w2285:dbl)  [unwired: 6 in, 1 out]
                      n817 = Greater Or Equal?(x=w2289, y=61.0) -> (x >= y?=w2287:bool)
                      n818 = Less?(x=w2285, y=u32 100) -> (x < y?=w2284:bool)
                      n819 = Compound Arithmetic op=OR(w2284, w2296, w2287, w2291) -> (w2295:bool)
                    }
                    n820 = control-ref of="Power transistor Heat sink Temp."() -> (w2255:refnum<vi>)
                    n821 = property class="DigNum (strict)"(reference=w2255, error in=w2252) -> (error out=w2254:errorcluster, "Value"=w2253:dbl)  [unwired: 1 out]
                    n822 = In Range and Coerce(upper limit=62.0, x=w2253, lower limit=58.0) -> (In Range?=w2249:bool)  [unwired: 1 out]
                    n823 = Build Array(w2250, w2249) -> (w2251:bool[])
                    n824 = Increment(x=w2265) -> (x+1=w2264:i32)
                    n825 = call "PassOrFail (SubVI).vi"("index (row)"=w2264, "error in (no error)"=w2254, "Data in"=w2253, "Pass?Fail"=w2249, "Table in"=w2262) -> ("error out"=w2267:errorcluster)  [unwired: 6 in]
                    n826 = And Array Elements(Boolean array=w2251) -> (logical AND=→"AuxiONResult 2":bool)
                    n827 = Increment(x=w2264) -> (x+1=w2263:i32)
                    n828 = Select(t="ON", s=w2250, f="OFF") -> (s? t:f=w2260:string)
                    n829 = call "PassOrFail (SubVI).vi"("String Res"=w2260, "index (row)"=w2263, "error in (no error)"=w2267, "Data in"=-3.0, "Pass?Fail"=w2250, "Table in"=w2262) -> ("error out"=w2266:errorcluster)  [unwired: 5 in]
                    n830 = call "TesterOption (SubVI).vi"("On/Off 2"=FALSE, "Tester Option 2"=T13."Venable", "2 Options"=TRUE, "error in (no error)"=w2266, "On/Off"=FALSE, "Tester Option"=T13."Fan", "VISA Refnum in"=w2272) -> ("error out"=w2244:errorcluster)  [unwired: 3 in, 1 out]
                    n831 = call "Time Delay23"("error in (no error)"=w2244) -> ("error out"=w2243:errorcluster)  [unwired: 10 in]
                    n832 = property class="Bool (strict)"(reference=w2277, error in=w2243) -> ("Value"=w2283:bool)  [unwired: 2 out]
                    n833 = Select(t=enum16{"Stop", "CoolingON", "HotGunON", "Start"}."Stop", s=w2283, f=enum16{"Stop", "CoolingON", "HotGunON", "Start"}."CoolingON") -> (s? t:f=w2274:enum16{"Stop", "CoolingON", "HotGunON", "Start"})
                  }
                  frame "Start" {
                    n834 = call "Write panel message (SubVI).vi"("Stop BurnIn"=w2332, 4:"rpm"=w2329, 5:"rpm"=FALSE ("rpm"), "PrintTime"=FALSE, "Stop"=w2331, "Time to wait"=1.0, "Strin"=w2330, "String in"=w2333) -> ("error out"=w2340:errorcluster)  [unwired: 3 in]
                    n835 = call "TesterOption (SubVI).vi"("On/Off 2"=TRUE, "Tester Option 2"=T13."Fan", "2 Options"=TRUE, "error in (no error)"=w2340, "On/Off"=FALSE, "Tester Option"=T13."Venable", "VISA Refnum in"=w2328) -> ("error out"=w2335:errorcluster)  [unwired: 3 in, 1 out]
                    n836 = disable-structure shown="Enabled" {
                      disable-tunnel: w2335 -> [w2357 _]
                      disable-tunnel: w2334 -> [w2356 _]
                      disable-tunnel: w2333 -> [w2355 _]
                      disable-tunnel: w2332 -> [w2354 _]
                      disable-tunnel: w2331 -> [w2353 _]
                      disable-tunnel: w2330 -> [w2352 _]
                      disable-tunnel: w2329 -> [w2351 _]
                      disable-tunnel: w2328 -> [w2349 _]
                      disable-tunnel: w2327 -> [w2347 _]
                      disable-tunnel: w2326 -> [w2345 _]
                      disable-tunnel: [w2344 _] -> w2324
                      frame Disabled {
                        n837 = while {
                          tunnel: w2357 -> [w2374]
                          tunnel: w2356 -> [w2373]
                          tunnel: w2355 -> [w2372]
                          tunnel: w2354 -> [w2371]
                          tunnel: w2353 -> [w2370]
                          tunnel: w2352 -> [w2369]
                          tunnel: w2351 -> [w2368]
                          shift-right: [w2365] -> _
                          shift-left: enum16{"Wait", "OFF", "ON", "Start"}."Start" -> [w2367]
                          tunnel: w2349 -> [w2366]
                          shift-right: [w2363] -> _
                          shift-left: 0 -> [w2364]
                          tunnel: w2347 -> [w2361]
                          shift-right: [w2360] -> w2344
                          shift-left: TRUE -> [w2359]
                          tunnel: w2345 -> [w2358]
                          stop <- w2362 stop-if-true
                          n838 = case shown="\"Start\"" w2367 {
                            tunnel: w2374 -> [_ w2421 _ w2484]
                            tunnel: w2373 -> [w2389 w2420 _ w2483]
                            tunnel: w2372 -> [_ w2418 _ w2481]
                            tunnel: w2371 -> [_ w2417 _ w2480]
                            tunnel: w2370 -> [_ w2396 _ w2464]
                            tunnel: w2369 -> [_ w2416 _ w2479]
                            tunnel: w2368 -> [_ w2415 _ w2478]
                            tunnel: w2366 -> [_ w2408 _ w2471]
                            tunnel: [w2392 w2398 enum16{"Wait", "OFF", "ON", "Start"}."OFF" w2461] -> w2365
                            tunnel: w2364 -> [w2393 w2406 _ w2469]
                            tunnel: [w2393 w2405 0 w2468] -> w2363
                            tunnel: [w2391 FALSE FALSE FALSE] -> w2362
                            tunnel: w2361 -> [w2377 _ w2457 _]
                            tunnel: [FALSE w2402 TRUE w2465] -> w2360
                            tunnel: w2359 -> [w2380 _ w2458 _]
                            tunnel: w2358 -> [w2379 _ w2456 _]
                            frame "Wait", Default {
                              n839 = call "SerialMarvinSendGet.vi"("write buffer"="EP=1\r\nAU=0\r\n", "VISA resource name"=w2389) -> ("error out"=w2388:errorcluster)  [unwired: 8 in, 1 out]
                              n840 = call "Time Delay24"("error in (no error)"=w2388) -> ("error out"=w2376:errorcluster)  [unwired: 10 in]
                              n841 = Not(x=w2380) -> (.not. x?=w2382:bool)
                              n842 = Select(t="OFF", s=w2382, f="ON") -> (s? t:f=w2381:string)
                              n843 = Add(x=2, y=w2379) -> (x+y=w2386:i32)
                              n844 = call "PassOrFail (SubVI).vi"("String Res"=w2381, "index (row)"=w2386, "error in (no error)"=w2376, "Data in"=-3.0, "Pass?Fail"=w2382, "Table in"=w2377) -> ("error out"=w2375:errorcluster)  [unwired: 5 in]
                              n845 = flat-sequence {
                                tunnel: [enum16{"Wait", "OFF", "ON", "Start"}."Wait"] -> w2392
                                tunnel: [TRUE] -> w2391
                                tunnel: w2375 -> [_]
                                frame #0 {
                                }
                              }
                            }
                            frame "OFF" {
                              n846 = call "SerialMarvinSendGet.vi"("error in (no error)"=w2421, "write buffer"="EP=1\r\nAU=0\r\n", "VISA resource name"=w2420) -> ("error out"=w2410:errorcluster)  [unwired: 7 in, 1 out]
                              n847 = call "Time Delay25"("error in (no error)"=w2410) -> ("error out"=w2404:errorcluster)  [unwired: 10 in]
                              n848 = call "GetADCTester (SubVI).vi"("error in (no error)"=w2404, "GetADCTester"=T15."Fan", "TimeToGet"=5, "VISA Refnum in"=w2408) -> ("error out"=w2409:errorcluster, "ADCValOutput Single"=w2412:dbl)  [unwired: 5 in, 1 out]
                              n849 = Greater?(x=w2412, y=2400.0) -> (0:w2407:bool)
                              n850 = case shown="True" w2407 {
                                tunnel: w2418 -> [_ w2440]
                                tunnel: w2417 -> [_ w2439]
                                tunnel: w2396 -> [_ w2438]
                                tunnel: w2416 -> [_ w2437]
                                tunnel: w2415 -> [_ w2436]
                                tunnel: w2409 -> [w2423 w2435]
                                tunnel: [w2424 w2433] -> w2397
                                tunnel: w2406 -> [w2428 _]
                                tunnel: [w2429 0] -> w2405
                                tunnel: [w2423 w2431] -> w2399
                                tunnel: [w2422 FALSE] -> w2402
                                frame False {
                                n851 = Increment(x=w2428) -> (x+1=w2429:i32)
                                n852 = Greater Or Equal?(x=w2428, y=10) -> (x >= y?=w2422:bool)
                                n853 = Select(t=enum16{"Wait", "OFF", "ON", "Start"}."Wait", s=w2422, f=enum16{"Wait", "OFF", "ON", "Start"}."OFF") -> (s? t:f=w2424:enum16{"Wait", "OFF", "ON", "Start"})
                                }
                                frame True {
                                n854 = call "Write panel message (SubVI).vi"("Stop BurnIn"=w2439, 4:"rpm"=w2436, 5:"rpm"=FALSE ("rpm"), "PrintTime"=TRUE, "Stop"=w2438, "error in (no error)"=w2435, "Time to wait"=5.0, "Strin"=w2437, "String in"=w2440) -> ("error out"=w2434:errorcluster)  [unwired: 2 in]
                                n855 = flat-sequence {
                                tunnel: w2434 -> [w2444]
                                tunnel: [enum16{"Wait", "OFF", "ON", "Start"}."Wait"] -> w2433
                                tunnel: [w2444] -> w2431
                                frame #0 {
                                }
                                }
                                }
                              }
                              n856 = property class="Bool (strict)"(reference=w2396, error in=w2399) -> ("Value"=w2401:bool)  [unwired: 2 out]
                              n857 = Select(t=enum16{"Wait", "OFF", "ON", "Start"}."Wait", s=w2401, f=w2397) -> (s? t:f=w2398:enum16{"Wait", "OFF", "ON", "Start"})
                            }
                            frame "ON" {
                              n858 = Not(x=w2458) -> (.not. x?=w2451:bool)
                              n859 = Select(t="ON", s=w2451, f="OFF") -> (s? t:f=w2450:string)
                              n860 = Increment(x=w2456) -> (x+1=w2455:i32)
                              n861 = call "PassOrFail (SubVI).vi"("String Res"=w2450, "index (row)"=w2455, "Data in"=-3.0, "Pass?Fail"=w2451, "Table in"=w2457) -> ()  [unwired: 6 in, 1 out]
                            }
                            frame "Start" {
                              n862 = call "SerialMarvinSendGet.vi"("error in (no error)"=w2484, "write buffer"="EP=1\r\nAU=1\r\n", "VISA resource name"=w2483) -> ("error out"=w2473:errorcluster)  [unwired: 7 in, 1 out]
                              n863 = call "Time Delay26"("error in (no error)"=w2473) -> ("error out"=w2467:errorcluster)  [unwired: 10 in]
                              n864 = call "GetADCTester (SubVI).vi"("error in (no error)"=w2467, "GetADCTester"=T15."Fan", "TimeToGet"=5, "VISA Refnum in"=w2471) -> ("error out"=w2472:errorcluster, "ADCValOutput Single"=w2475:dbl)  [unwired: 5 in, 1 out]
                              n865 = Less?(x=w2475, y=100.0) -> (x < y?=w2470:bool)
                              n866 = case shown="False" w2470 {
                                tunnel: w2481 -> [_ w2503]
                                tunnel: w2480 -> [_ w2502]
                                tunnel: w2464 -> [_ w2501]
                                tunnel: w2479 -> [_ w2500]
                                tunnel: w2478 -> [_ w2499]
                                tunnel: w2472 -> [w2486 w2498]
                                tunnel: [w2487 w2496] -> w2462
                                tunnel: w2469 -> [w2491 _]
                                tunnel: [w2492 0] -> w2468
                                tunnel: [w2486 w2494] -> w2459
                                tunnel: [w2485 FALSE] -> w2465
                                frame False {
                                n867 = Increment(x=w2491) -> (x+1=w2492:i32)
                                n868 = Greater Or Equal?(x=w2491, y=5) -> (x >= y?=w2485:bool)
                                n869 = Select(t=enum16{"Wait", "OFF", "ON", "Start"}."ON", s=w2485, f=enum16{"Wait", "OFF", "ON", "Start"}."Start") -> (s? t:f=w2487:enum16{"Wait", "OFF", "ON", "Start"})
                                }
                                frame True {
                                n870 = call "Write panel message (SubVI).vi"("Stop BurnIn"=w2502, 4:"rpm"=w2499, 5:"rpm"=FALSE ("rpm"), "PrintTime"=TRUE, "Stop"=w2501, "error in (no error)"=w2498, "Time to wait"=60.0, "Strin"=w2500, "String in"=w2503) -> ("error out"=w2497:errorcluster)  [unwired: 2 in]
                                n871 = flat-sequence {
                                tunnel: w2497 -> [w2507]
                                tunnel: [enum16{"Wait", "OFF", "ON", "Start"}."ON"] -> w2496
                                tunnel: [w2507] -> w2494
                                frame #0 {
                                }
                                }
                                }
                              }
                              n872 = property class="Bool (strict)"(reference=w2464, error in=w2459) -> ("Value"=w2463:bool)  [unwired: 2 out]
                              n873 = Select(t=enum16{"Wait", "OFF", "ON", "Start"}."Wait", s=w2463, f=w2462) -> (s? t:f=w2461:enum16{"Wait", "OFF", "ON", "Start"})
                            }
                          }
                        }
                      }
                      frame Enabled {
                      }
                    }
                    n874 = flat-sequence {
                      tunnel: [enum16{"Stop", "CoolingON", "HotGunON", "Start"}."HotGunON"] -> w2325
                      tunnel: w2324 -> [_]
                      frame #0 {
                      }
                    }
                  }
                }
              }
            }
          }
        }
      }
      "CurrentTest" <- w229
    }
    n875 = flat-sequence {
      tunnel: w216 -> [_]
      frame #0 {
        w224 = T21."Enabled" ("Disabled")
        w225 = FALSE ("Start")
        n876 = property on="Start" class="Bool (strict)"("Value"=w225, "DisabledEnum"=w224) -> ()  [unwired: 2 in, 2 out]
        n877 = property on="Report" class="Bool (strict)"("Value"=w225, "DisabledEnum"=w224) -> ()  [unwired: 2 in, 2 out]
      }
    }
  }
  n878 = while {
    shift-right: [w2515] -> _
    shift-left: T11."Initialize" -> [w2534]
    shift-right: [w2531] -> _
    shift-left: _ -> [w2530]
    shift-right: [w2529] -> _
    shift-left: w33 -> [w2527]
    shift-right: [w2528] -> _
    shift-left: refnum<vi> refnum ("Config_CANAT") -> [w2526]
    shift-right: [w2524] -> _
    shift-left: w30 -> [w2525]
    tunnel: "ATR" -> [_]
    tunnel: w22 -> [w2523]
    tunnel: w21 -> [w2522]
    shift-right: [w2520] -> _
    shift-left: w2 -> [w2521]
    tunnel: w8 -> [w2519]
    tunnel: w3 -> [w2518]
    tunnel: w19 -> [_]
    tunnel: w31 -> [w2533]
    tunnel: [w2532] -> _
    tunnel: w9 -> [_]
    tunnel: w1 -> [w2516]
    shift-right: [w2513] -> _
    shift-left: w2 -> [w2514]
    shift-right: [w2511] -> _
    shift-left: w2 -> [w2512]
    tunnel: w1 -> [w2510]
    stop <- w2517 stop-if-true
    n879 = case shown="\"MainProgram\"" w2534 {
      tunnel: [w2545 w2693 w2769 T11."Erase ATR Table"] -> w2515
      tunnel: [FALSE w2679 FALSE FALSE] -> w2517
      tunnel: [w2541 w2684 w2763 w3804] -> w2532
      tunnel: w2533 -> [_ w2704 w2767 _]
      tunnel: [w2578 refnum<visa-resource-name> refnum ("VISA resource name") w2764 w3808] -> w2531
      tunnel: w2530 -> [w2578 w2712 w2765 _]
      tunnel: [w2569 w2673 w2759 w3802] -> w2529
      tunnel: [w2568 refnum<vi> refnum ("Config_CANAT") w2760 w3805] -> w2528
      tunnel: w2527 -> [w2569 w2714 w2762 w3802]
      tunnel: w2526 -> [w2568 w2696 w2761 _]
      tunnel: w2525 -> [w2567 w2707 w2758 w3801]
      tunnel: [w2567 w2672 w2757 w3801] -> w2524
      tunnel: w2523 -> [_ _ w2756 _]
      tunnel: w2522 -> [_ _ w2755 _]
      tunnel: w2521 -> [w2564 w2698 w2754 w3798]
      tunnel: [w2564 w2698 w2753 w3798] -> w2520
      tunnel: w2519 -> [w2554 _ w2752 _]
      tunnel: w2518 -> [_ _ w2751 _]
      tunnel: w2516 -> [_ _ w2750 _]
      tunnel: w2514 -> [_ _ w2749 _]
      tunnel: [w2539 w2671 w2748 w3789] -> w2513
      tunnel: w2512 -> [_ _ w2747 _]
      tunnel: [w2539 w2671 w2746 w3789] -> w2511
      tunnel: w2510 -> [_ _ w2745 _]
      frame "Erase ATR Table", Default {
        w2539 = 0
        w2548 = T21."Enabled" ("Disabled")
        w2558 = "Marvin" ("section")
        w2565 = refnum<visa-resource-name> "COM4" ("VISA resource name")
        w2574 = FALSE ("Visible")
        n880 = property on="Serial Com" class="Bool"(error in=errorcluster {"status"=FALSE, "code"=0, "source"=""} ("error out"), "Visible"=TRUE) -> (error out=w2566:errorcluster)  [unwired: 1 in, 1 out]
        n881 = property on="VISA Marvin" class="VISAName"(error in=w2566, "Visible"=w2574, "Value"=w2565) -> (error out=w2576:errorcluster)  [unwired: 1 in, 1 out]
        n882 = property on="VISA Marvin" class="VISAName"(error in=w2566, "Value"=w2565) -> ()  [unwired: 1 in, 2 out]
        n883 = property on="Status" class="Bool (strict)"(error in=w2576, "Value"=w2574) -> (error out=w2551:errorcluster)  [unwired: 1 in, 1 out]
        n884 = call "Select UUT"("error in (no error)"=w2551) -> ("EBAY"=w2549:bool, "error out"=w2550:errorcluster)  [unwired: 17 in]
        n885 = case shown="False" w2549 {
          tunnel: [string[][] [["1", "Communication Test", "", "", "", "", ""], ["1.1", "Serial RS-232", "N/A", "-", "", "", ""], ["1.2", "CAN Bus", "N/A", "-", "", "", ""], ["", "", "", "", "", "", ""], ["2", "Temperature Sensor Calibration", "", "", "", "", ""], ["2.1", "Sensor Reading Analog Offset", "0", "+/-0.100", ".", "", ""], ["", "", "", "", "", "", ""], ["3", "Motor Termistor Input Test", "", "", "", "", ""], ["3.1", "60 Degree", "60", "+/-3.00", "°C", "", ""], ["3.2", "90 Degree", "90", "+/-3.00", "°C", "", ""], ["3.3", "120 Degree", "120", "+/-3.00", "°C", "", ""], ["", "", "", "", "", "", ""], ["4", "Enable Test", "", "", "", "", ""], ["4.1", "Fan Speed at Opened Enable ", "5000", "+/-200.0", "rpm", "", ""], ["4.2", "Fan Speed at Opened Enable ", "0", "+/-200.0", "rpm", "", ""], ["4.3", "Fan Speed at Closed Enable ", "5000", "+/-200.0", "rpm", "", ""], ["4.4", "Motor Rotation Direction", "CCW", "-", "", "", ""], ["", "", "", "", "", "", ""], ["5", "Speed Command Test", "", "", "", "", ""], ["5.1", "Fan  Speed", "6000", "+/-200.0", "rpm", "", ""], ["5.2", "Fan  Speed", "9000", "+/-200.0", "rpm", "", ""], ["5.3", "Fan  Speed", "12100", "+/-200.0", "rpm", "", ""], ["", "", "", "", "", "", ""], ["6", "Motor Stop time", "< 50", "-", "sec", "", ""], ["", "", "", "", "", "", ""], ["7", "Burn-in Test", "", "", "", "", ""], ["7.1", "DC Input Current", "28", "+/-5.000", "A", "", ""], ["7.2", "Fan speed", "12100", "+/-200.0", "rpm", "", ""], ["7.3", "Ambient Temperature", "25", "+/-13.00", "°C", "", ""], ["7.4", "After 10 min of operation", "", "-", "°C", "", ""], ["7.5", "After 20 min of operation", "", "-", "°C", "", ""], ["7.6", "After 30 min of operation", "", "-", "°C", "", ""], ["", "", "", "", "", "", ""], ["8", "Visual Inspection", "", "", "", "", ""], ["8.1", "Verification of Components Not Installed", "N/A", "-", "", "", ""], ["8.2", "Manufacturing Defects", "N/A", "-", "", "", ""], ["", "", "", "", "", "", ""], ["9", "Power Supply Testing", "", "", "", "", ""], ["9.1", "DC Input Current Drawn", "150", "+/-10.00", "mA", "", ""], ["", "", "", "", "", "", ""], ["10", "Power Supply Voltages", "", "", "", "", ""], ["10.1", "12V", "12.0", "+/-0.500", "V", "", ""], ["10.2", "5V", "5.0", "+/-0.200", "V", "", ""], ["10.3", "3.3V", "3.3", "+/-0.100", "V", "", ""], ["10.4", "1.8V", "1.8", "+/-0.100", "V", "", ""], ["", "", "", "", "", "", ""], ["11", "Reverse Polarity Test - DC Input Current", "< 1", "-", "mA", "", ""], ["", "", "", "", "", "", ""], ["12", "Functional Test Procedure", "", "", "", "", ""], ["12.1", "Weight Check", "3800", "+/-100.0", "gr", "", ""], ["", "", "", "", "", "", ""], ["13", "Insulation Resistance Test", "", "", "", "", ""], ["13.1", "J3.B to Chassis", "> 1M", "-", "ohms", "", ""], ["13.2", "J1.16 to Chassis", "> 100K", "-", "ohms", "", ""], ["", "", "", "", "", "", ""], ["14", "Bonding Resistance", "", "", "", "", ""], ["14.1", "J1 Body to Chassis", "< 2m", "-", "ohms", "", ""], ["14.2", "J2  Body to Chassis", "< 2m", "-", "ohms", "", ""], ["14.3", "J3  Body to Chassis", "< 2m", "-", "ohms", "", ""], ["", "", "", "", "", "", ""], ["15", "CANbus Resistance Test", "", "", "", "", ""], ["15.1", "J1.17 to J1.18", "> 10K", "-", "ohms", "", ""], ["", "", "", "", "", "", ""], ["16", "Sealing Test", "N/A", "-", "", "", ""], ["", "", "", "", "", "", ""], ["17", "Mounting Holes Test - Jig Fit", "214", "-", "mm", "", ""]] ("ArrAHU 2") string[][] [["1", "Communication Test", "", "", "", "", ""], ["1.1", "Serial RS-232", "N/A", "-", "", "", ""], ["1.2", "CAN Bus", "N/A", "-", "", "", ""], ["", "", "", "", "", "", ""], ["2", "Auxiliary Fan Test", "", "", "", "", ""], ["2.1", "Fan status-ON", "ON", "-", "-", "", ""], ["2.2", "Fan status-OFF", "OFF", "-", "-", "", ""], ["", "", "", "", "", "", ""], ["3", "Temperature Sensor Calibration", "", "", "", "", ""], ["3.1", "Sensor Reading Analog Offset", "0", "+/-0.100", ".", "", ""], ["", "", "", "", "", "", ""], ["4", "Motor Termistor Input Test", "", "", "", "", ""], ["4.1", "60 Degree", "60", "+/-3.00", "°C", "", ""], ["4.2", "90 Degree", "90", "+/-3.00", "°C", "", ""], ["4.3", "120 Degree", "120", "+/-3.00", "°C", "", ""], ["", "", "", "", "", "", ""], ["5", "Enable Test", "", "", "", "", ""], ["5.1", "Fan Speed at Opened Enable ", "5000", "+/-200.0", "rpm", "", ""], ["5.2", "Fan Speed at Opened Enable ", "0", "+/-200.0", "rpm", "", ""], ["5.3", "Fan Speed at Closed Enable ", "5000", "+/-200.0", "rpm", "", ""], ["5.4", "Motor Rotation Direction", "CCW", "-", "", "", ""], ["", "", "", "", "", "", ""], ["6", "Speed Command Test", "", "", "", "", ""], ["6.1", "Fan  Speed", "11500", "+/-200.0", "rpm", "", ""], ["6.2", "Fan  Speed", "12700", "+/-200.0", "rpm", "", ""], ["6.3", "Fan  Speed", "14700", "+/-200.0", "rpm", "", ""], ["", "", "", "", "", "", ""], ["7", "Motor Stop time", "< 50", "-", "sec", "", ""], ["", "", "", "", "", "", ""], ["8", "Temperature Control Algorithm Test", "", "", "", "", ""], ["8.1", "Tair <   67 ± 3 °C", "11500", "+/-200.0", "rpm", "", ""], ["8.2", "Measured Temp.", "", "", "°C", "", ""], ["8.3", "Tair >= 67 ± 3 °C", "12700", "+/-200.0", "rpm", "", ""], ["8.4", "Transition Temp.", "", "", "°C", "", ""], ["8.5", "Tair >= 83 ± 3 °C", "14700", "+/-400.0", "rpm", "", ""], ["8.6", "Transition Temp.", "", "", "°C", "", ""], ["8.7", "Tair <= 80 ± 3 °C", "12700", "+/-200.0", "rpm", "", ""], ["8.8", "Transition Temp.", "", "", "°C", "", ""], ["8.9", "Tair <= 64 ± 3 °C", "11500", "+/-200.0", "rpm", "", ""], ["8.10", "Transition Temp.", "", "", "°C", "", ""], ["", "", "", "", "", "", ""], ["9", "Burn-in Test", "", "", "", "", ""], ["9.1", "DC Input Current", "45", "+/-5.000", "A", "", ""], ["9.2", "Fan speed", "14700", "+/-200.0", "rpm", "", ""], ["9.3", "Ambient Temperature", "25", "+/-13.00", "°C", "", ""], ["9.4", "After 10 min of operation", "", "-", "°C", "", ""], ["9.5", "After 20 min of operation", "", "-", "°C", "", ""], ["9.6", "After 30 min of operation", "", "-", "°C", "", ""], ["", "", "", "", "", "", ""], ["10", "Visual Inspection", "", "", "", "", ""], ["10.1", "Verification of Components Not Installed", "N/A", "-", "", "", ""], ["10.2", "Manufacturing Defects", "N/A", "-", "", "", ""], ["", "", "", "", "", "", ""], ["11", "Power Supply Testing", "", "", "", "", ""], ["11.1", "DC Input Current Drawn", "150", "+/-10.00", "mA", "", ""], ["", "", "", "", "", "", ""], ["12", "Power Supply Voltages", "", "", "", "", ""], ["12.1", "12V", "12.0", "+/-0.500", "V", "", ""], ["12.2", "5V", "5.0", "+/-0.200", "V", "", ""], ["12.3", "3.3V", "3.3", "+/-0.100", "V", "", ""], ["12.4", "1.8V", "1.8", "+/-0.100", "V", "", ""], ["", "", "", "", "", "", ""], ["13", "Reverse Polarity Test - DC Input Current", "< 1", "-", "mA", "", ""], ["", "", "", "", "", "", ""], ["14", "Functional Test Procedure", "", "", "", "", ""], ["14.1", "Weight Check", "4180", "+/-100.0", "gr", "", ""], ["", "", "", "", "", "", ""], ["15", "Insulation Resistance Test", "", "", "", "", ""], ["15.1", "J3.B to Chassis", "> 1M", "-", "ohms", "", ""], ["15.2", "J1.16 to Chassis", "> 100K", "-", "ohms", "", ""], ["", "", "", "", "", "", ""], ["16", "Bonding Resistance", "", "", "", "", ""], ["16.1", "J1 Body to Chassis", "< 2m", "-", "ohms", "", ""], ["16.2", "J2  Body to Chassis", "< 2m", "-", "ohms", "", ""], ["16.3", "J3  Body to Chassis", "< 2m", "-", "ohms", "", ""], ["", "", "", "", "", "", ""], ["17", "CANbus Resistance Test", "", "", "", "", ""], ["17.1", "J1.17 to J1.18", "> 10K", "-", "ohms", "", ""], ["", "", "", "", "", "", ""], ["18", "Sealing Test", "N/A", "-", "", "", ""], ["", "", "", "", "", "", ""], ["19", "Mounting Holes Test - Jig Fit", "214", "-", "mm", "", ""]] ("ArrEbay 3")] -> w2572
          tunnel: ["AHU" "EBAY"] -> w2571
          tunnel: [w2642 w2655] -> w2570
          tunnel: w2550 -> [w2643 w2655]
          tunnel: [w2638 u8 95] -> w2538
          frame False {
            (unwired) string[][] [["6.1", "Visual Inspection", "", "", "", "", ""], ["6.1.1", "Verification of Components Not Installed", "N/A", "-", "", "", ""], ["", "", "", "", "", "", ""], ["6.1.2", "Manufacturing Defects", "N/A", "-", "", "", ""], ["", "", "", "", "", "", ""], ["6.2", "Power Supply Testing", "", "", "", "", ""], ["6.2.1", "Input Current Drawn", "", "", "", "", ""], ["6.2.1.1", "DC Input Current", "< 150", "-", "mA", "", ""], ["", "", "", "", "", "", ""], ["6.2.2", "Power Supply Voltages", "", "", "", "", ""], ["6.2.2.1", "12V", "12.0", "+/-0.500", "V", "", ""], ["6.2.2.2", "5V", "5.0", "+/-0.200", "V", "", ""], ["6.2.2.3", "3.3V", "3.3", "+/-0.100", "V", "", ""], ["6.2.2.4", "1.8V", "1.8", "+/-0.100", "V", "", ""], ["", "", "", "", "", "", ""], ["7", "Functional Test Procedure", "", "", "", "", ""], ["7.1", "Weight Check", "3800", "+/-100.0", "gr", "", ""], ["", "", "", "", "", "", ""], ["7.2", "Insulation Resistance Test", "", "", "", "", ""], ["7.2.1", "J3.B to Chassis", "> 1M", "-", "W", "", ""], ["7.2.2", "J1.16 to Chassis", "> 100K", "-", "W", "", ""], ["", "", "", "", "", "", ""], ["7.2", "Bonding Resistance", "", "", "", "", ""], ["7.2.3", "J1 Body to Chassis", "< 2m", "-", "W", "", ""], ["7.2.4", "J2  Body to Chassis", "< 2m", "-", "W", "", ""], ["7.2.5", "J3  Body to Chassis", "< 2m", "-", "W", "", ""], ["", "", "", "", "", "", ""], ["7.2.1", "CANbus Resistance Test", "", "", "", "", ""], ["7.2.1.1", "J1.17 to J1.18", "> 10K", "-", "W", "", ""], ["", "", "", "", "", "", ""], ["7.3", "Sealing Test", "N/A", "-", "", "", ""], ["", "", "", "", "", "", ""], ["7.4", "Communication Test", "", "", "", "", ""], ["7.4.1", "Serial RS-232", "N/A", "-", "", "", ""], ["7.4.2", "CAN Bus", "N/A", "-", "", "", ""], ["", "", "", "", "", "", ""], ["7.5", "Performances Tests", "", "", "", "", ""], ["7.5.1", "Reverse Polarity Test", "", "", "", "", ""], ["7.5.1.1", "DC Input Current", "< 1", "-", "mA", "", ""], ["", "", "", "", "", "", ""], ["7.5.2", "Enable Test", "", "", "", "", ""], ["7.5.2.1", "Fan Speed at Opened Enable ", "5000", "+/-200.0", "rpm", "", ""], ["7.5.2.2", "Fan Speed at Opened Enable ", "0", "+/-200.0", "rpm", "", ""], ["7.5.2.3", "Fan Speed at Closed Enable ", "5000", "+/-200.0", "rpm", "", ""], ["7.5.2.4", "Motor Rotation Direction", "Counter-clockwise (Inlet)", "-", "", "", ""], ["", "", "", "", "", "", ""], ["7.5.3", "Stop Time Test ", "", "", "", "", ""], ["7.5.3.1", "Motor Stop time", "< 50", "-", "sec", "", ""], ["", "", "", "", "", "", ""], ["7.5.4", "Speed Command Test", "", "", "", "", ""], ["7.5.4.1", "Fan Speed", "6000", "+/-200.0", "rpm", "", ""], ["7.5.4.2", "Fan Speed", "9000", "+/-200.0", "rpm", "", ""], ["7.5.4.3", "Fan Speed", "12100", "+/-200.0", "rpm", "", ""], ["", "", "", "", "", "", ""], ["7.5.5", "Temperature Sensor Calibration Test", "", "", "", "", ""], ["7.5.5.1", "Sensor Reading Analog Offset", "0", "+/-0.100", ".", "", ""], ["", "", "", "", "", "", ""], ["7.5.6", "Burn-in Test", "", "", "", "", ""], ["7.5.6.1", "DC Input Current", "28", "+/-3.000", "A", "", ""], ["7.5.6.2", "Fan Speed", "12100", "+/-200.000", "rpm", "", ""], ["7.5.6.3", "Ambient Temperature", "25", "+/-13.00", "C", "", ""], ["7.5.6.4", "After 10 min of operation", "", "", "C", "", ""], ["7.5.6.5", "After 20 min of operation", "", "", "C", "", ""], ["7.5.6.6", "After 30 min of operation", "", "", "C", "", ""], ["", "", "", "", "", "", ""], ["9", "Motor Temp Test", "", "", "", "", ""], ["9.1", "60 C", "60", "+/-3.000", "C", "", ""], ["9.2", "90 C", "90", "+/-3.000", "C", "", ""], ["9.3", "120 C", "120", "+/-3.000", "C", "", ""]] ("data")
            n886 = while {
              shift-right: [w2650] -> w2642
              shift-left: w2643 -> [w2651]
              tunnel: [w2645] -> w2641
              stop <- w2649 stop-if-true
              n887 = call "AHU UUT (subVI).vi"("error in (no error)"=w2651) -> ("AHU 47"=w2646:bool, "AHU 63"=w2645:bool, "OK"=w2648:bool, "error out"=w2650:errorcluster)  [unwired: 15 in]
              n888 = Exclusive Or(1:w2646, 2:w2645) -> (0:w2647:bool)
              n889 = And(x=w2648, y=w2647) -> (x .and. y?=w2649:bool)
            }
            n890 = Select(t=u8 63, s=w2641, f=u8 47) -> (s? t:f=w2638:u8)
          }
          frame True {
            # "5.4.0"
            "MaxEbaySpeed" <- u16 14700 ("MaxEbaySpeed")
          }
        }
        "UUT" <- w2571
        "UUT" <- w2538
        n891 = for {
          tunnel: w2572 -> [w2661] mode=indexing
          tunnel: w2570 -> [w2659]
          tunnel: [w2658] -> w2543
          tunnel: w2572 -> [w2657]
          i -> [w2660]
          n892 = for {
            tunnel: w2661 -> [_] mode=indexing
            tunnel: w2660 -> [w2667]
            tunnel: w2659 -> [w2664]
            tunnel: [w2663] -> w2658
            tunnel: w2657 -> [w2662]
            i -> [w2668]
            n893 = Bundle By Name(cluster=T22 {"Row"=0, "Column"=0} ("Active Cell:Active Cell"), "Row"=w2667, "Column"=w2668) -> (w2666:T22)
            n894 = control-ref of="ATR"() -> (w2665:refnum<vi>)
            n895 = property class="Tbl (strict)"(reference=w2665, error in=w2664, "Active Cell"=w2666, "Cell BG Color"=u32 16777226, "Value"=w2662) -> (error out=w2663:errorcluster)  [unwired: 1 out]
          }
        }
        n896 = case shown="95" w2538 {
          tunnel: ["AHU Software Version" ("key") "AHU Software Version" ("key") "EBAY Software Version1" ("key")] -> w2560
          tunnel: ["AHU R Serial Number" ("key") "AHU L Serial Number" ("key") "EBAY Serial Number" ("key")] -> w2561
          tunnel: [2 2 1] -> w2547
          frame 63, Default {
          }
          frame 47 {
          }
          frame 95 {
          }
        }
        n897 = property on="Start" class="Bool (strict)"("DisabledEnum"=w2548) -> ()  [unwired: 2 in, 2 out]
        n898 = property on="Report" class="Bool (strict)"("DisabledEnum"=w2548) -> ()  [unwired: 2 in, 2 out]
        n899 = call <vilib>:"Open Config Data.vi"("error in (no error)"=w2543, "create file if necessary (T)"=FALSE, "configuration file path"=w2554) -> ("error out"=w2555:errorcluster, "refnum"=w2556:T12)  [unwired: 7 out]
        n900 = call-poly <vilib>:"Read Key.vi"("section"=w2558, "error in (no error)"=w2555, "key"=w2560, "refnum"=w2556) -> ("error out"=w2562:errorcluster, "value"=→"UUT SoftwareVer":string, "refnum out"=w2559:T12)  [unwired: 2 in, 3 out]
        n901 = call-poly <vilib>:"Read Key.vi"("section"=w2558, "error in (no error)"=w2562, "key"=w2561, "refnum"=w2559) -> ("error out"=w2536:errorcluster, "value"=w2552:string, "refnum out"=w2537:T12)  [unwired: 2 in, 3 out]
        n902 = case shown="95" w2538 {
          tunnel: w2537 -> [w2579 w2583]
          tunnel: w2536 -> [_ w2582]
          tunnel: [w2579 w2581] -> w2535
          frame 0, Default {
          }
          frame 95 {
            n903 = call-poly <vilib>:"Read Key.vi"("section"="Marvin", "error in (no error)"=w2582, "key"="EBAY Software Version2", "refnum"=w2583) -> ("value"=→"UUT SoftwareVer2":string, "refnum out"=w2581:T12)  [unwired: 2 in, 4 out]
          }
        }
        n904 = call <vilib>:"Close Config Data.vi"("refnum"=w2535) -> ("error out"=w2544:errorcluster)  [unwired: 9 in, 1 out]
        n905 = Decimal String To Number(string=w2552) -> (number=w2546:i32)  [unwired: 2 in, 1 out]
        n906 = case shown="63, Default" w2538 {
          tunnel: w2546 -> [w2605 w2618 _]
          tunnel: [w2601 w2614 T11."MainProgram"] -> w2545
          tunnel: w2544 -> [w2600 w2613 w2626]
          tunnel: [w2600 w2613 w2626] -> w2542
          tunnel: [w2599 w2612 FALSE] -> w2540
          frame 63, Default {
            n907 = Quotient & Remainder(x=w2605, y=2) -> (x-y*floor(x/y)=w2603:i32)  [unwired: 1 out]
            n908 = Equal To 0?(x=w2603) -> (x = 0?=w2602:bool)
            n909 = case shown="False" w2602 {
              tunnel: [T11."MainProgram" w2609] -> w2601
              tunnel: [FALSE w2608] -> w2599
              frame False {
              }
              frame True {
                n910 = flat-sequence {
                  tunnel: [T11."Stop"] -> w2609
                  tunnel: [TRUE] -> w2608
                  frame #0 {
                    n911 = call "Display Message to User11"() -> ()  [unwired: 10 in, 2 out]
                  }
                  frame #1 {
                  }
                }
              }
            }
          }
          frame 47 {
            n912 = Quotient & Remainder(x=w2618, y=2) -> (x-y*floor(x/y)=w2616:i32)  [unwired: 1 out]
            n913 = Not Equal To 0?(x=w2616) -> (x != 0?=w2615:bool)
            n914 = case shown="True" w2615 {
              tunnel: [T11."MainProgram" w2622] -> w2614
              tunnel: [FALSE w2621] -> w2612
              frame False {
              }
              frame True {
                n915 = flat-sequence {
                  tunnel: [T11."Stop"] -> w2622
                  tunnel: [TRUE] -> w2621
                  frame #0 {
                    n916 = call "Display Message to User13"() -> ()  [unwired: 10 in, 2 out]
                  }
                  frame #1 {
                  }
                }
              }
            }
          }
          frame 95 {
          }
        }
        n917 = case shown="False" w2540 {
          tunnel: w2542 -> [w2590 w2598]
          tunnel: [w2589 w2598] -> w2541
          frame False {
            n918 = call "Boards S/N"("error in (no error)"=w2590) -> ("POWER Board S/N"=→"POWER Board S/N":string, "DSP Board S/N"=→"DSP Board S/N":string, "error out"=w2588:errorcluster)  [unwired: 15 in, 1 out]
            n919 = call "COM EvolutionBoard.vi"("error in (no error)"=w2588, "VISA resource name 2"=refnum<visa-resource-name> "COM1" ("VISA resource name")) -> ("error out"=w2596:errorcluster, "VISA resource name out"=w2595:refnum<visa-resource-name>)  [unwired: 8 in]
            n920 = call "TesterOption (SubVI).vi"("2 Options"=FALSE, "error in (no error)"=w2596, "On/Off"=FALSE, "Tester Option"=T13."Venable", "VISA Refnum in"=w2595) -> ("error out"=w2589:errorcluster, "VISA Refnum out"=→"VISA Tester":refnum<visa-resource-name>)  [unwired: 5 in]
          }
          frame True {
          }
        }
        n921 = Add(x=w2546, y=w2547) -> (x+y=→"Next SN":i32)
      }
      frame "Stop" {
        w2671 = 0
        n922 = flat-sequence {
          tunnel: w2704 -> [w2742]
          tunnel: [w2741] -> w2697
          frame #0 {
            n923 = control-ref of="Pannel User Message"() -> (w2744:refnum<vi>)
            n924 = property class="Str"(reference=w2744, error in=w2742, "Value"="Program Stopped...\r\nPlease turn OFF All Power sinks") -> (error out=w2741:errorcluster)  [unwired: 1 out]
          }
        }
        n925 = control-ref of="VISA Tester"() -> (w2705:refnum<vi>)
        n926 = property class="VISAName"(reference=w2705, error in=w2697) -> ("Value"=w2703:refnum<visa-resource-name>)  [unwired: 2 out]
        n927 = disable-structure shown="Enabled" {
          disable-tunnel: w2697 -> [w2729 w2730]
          disable-tunnel: w2696 -> [w2727 _]
          disable-tunnel: [w2726 w2730] -> w2683
          frame Disabled {
            n928 = call "Clear CAN Buffer.vi"("error in (no error)"=w2729, "Cluster in"=w2727) -> ("error out"=w2728:errorcluster)  [unwired: 8 in, 1 out]
            n929 = call "Close CAN Device.vi"("error in (no error)"=w2728, "Cluster in"=w2727) -> ("error out"=w2726:errorcluster)  [unwired: 8 in, 1 out]
          }
          frame Enabled {
          }
        }
        n930 = VISA Close(VISA resource name=w2712, error in (no error)=w2697) -> (error out=w2706:errorcluster)
        n931 = property on="Stop Button" class="Bool (strict)"() -> ("Value"=w2675:bool)  [unwired: 2 in, 2 out]
        n932 = call "TesterOption (SubVI).vi"("2 Options"=FALSE, "On/Off"=FALSE, "Tester Option"=T13."Power", "VISA Refnum in"=w2703) -> ("error out"=w2692:errorcluster, "VISA Refnum out"=w2702:refnum<visa-resource-name>)  [unwired: 6 in]
        n933 = property on="ClosePanel" class="Bool (strict)"() -> ("Value"=w2676:bool)  [unwired: 2 in, 2 out]
        n934 = VISA Close(VISA resource name=w2702, error in (no error)=w2692) -> (error out=w2689:errorcluster)
        n935 = Or(x=w2676, y=w2675) -> (x .or. y?=w2674:bool)
        n936 = Flush Queue(queue=w2707, error in (no error)=w2706) -> (queue out=w2709:refnum<queue>, error out=w2708:errorcluster)  [unwired: 1 out]
        n937 = Flush Queue(queue=w2714, error in (no error)=w2706) -> (queue out=w2713:refnum<queue>, error out=w2715:errorcluster)  [unwired: 1 out]
        n938 = case shown="False" w2674 {
          tunnel: w2715 -> [w2717 w2725]
          tunnel: w2713 -> [w2719 w2721]
          tunnel: w2709 -> [w2718 w2720]
          tunnel: w2708 -> [w2716 w2724]
          tunnel: [w2717 w2723] -> w2691
          tunnel: [w2716 w2722] -> w2690
          tunnel: [w2719 w2721] -> w2673
          tunnel: [w2718 w2720] -> w2672
          frame False {
          }
          frame True {
            n939 = Release Queue(queue=w2720, error in (no error)=w2724) -> (error out=w2722:errorcluster)  [unwired: 1 in, 2 out]
            n940 = Release Queue(queue=w2721, error in (no error)=w2725) -> (error out=w2723:errorcluster)  [unwired: 1 in, 2 out]
          }
        }
        n941 = Merge Errors(w2691, w2690, w2689, w2683) -> (w2688:errorcluster)
        n942 = property on="Refresh Button" class="Bool (strict)"() -> ("Value"=w2677:bool)  [unwired: 2 in, 2 out]
        n943 = call <vilib>:"Clear Errors.vi"("error in (no error)"=w2688) -> ("error out"=w2687:errorcluster)  [unwired: 5 in, 1 out]
        n944 = property on="Stop Button" class="Bool (strict)"() -> ("Value"=w2681:bool)  [unwired: 2 in, 2 out]
        n945 = property on="ClosePanel" class="Bool (strict)"(error in=w2687) -> (error out=w2685:errorcluster, "Value"=w2686:bool)  [unwired: 1 in, 1 out]
        n946 = Not(x=w2677) -> (.not. x?=w2678:bool)
        n947 = Select(t=T11."Initialize", s=w2677, f=T11."Stop") -> (s? t:f=w2693:T11)
        n948 = Not(x=w2681) -> (.not. x?=w2680:bool)
        n949 = Compound Arithmetic op=AND(w2686, w2680, w2678) -> (w2682:bool)
        n950 = case shown="False" w2682 {
          tunnel: w2685 -> [w2733 w2737]
          tunnel: [w2733 w2737] -> w2684
          tunnel: [w2732 w2736] -> w2679
          tunnel: w2677 -> [w2731 _]
          frame False {
            n951 = case shown="False" w2731 {
              tunnel: [TRUE FALSE] -> w2732
              frame False {
              }
              frame True {
              }
            }
          }
          frame True {
            n952 = flat-sequence {
              tunnel: [TRUE] -> w2736
              frame #0 {
              }
              frame #1 {
                n953 = control-ref of="This VI"() -> (w2740:refnum<vi>)
                n954 = property class="VI"(reference=w2740, "FP.State"=T23."Closed" ("Front Panel Window:State")) -> ()  [unwired: 1 in, 2 out]
              }
            }
          }
        }
      }
      frame "MainProgram" {
        n955 = event shown="[7] \"Report\", \"Stop Button\": Value Change" {
          selector: w2756 -> [_ _ _ _ _ _ _ _ _ _ _ _ _]
          dyn-events: _ -> [_ _ _ _ _ _ _ _ _ _ _ _ _]
          timeout: 70 -> [_ _ _ _ _ _ _ _ _ _ _ _ _]
          tunnel: [T11."MainProgram" T11."MainProgram" T11."MainProgram" T11."MainProgram" T11."MainProgram" T11."Stop" T11."MainProgram" w3499 T11."MainProgram" T11."MainProgram" T11."MainProgram" T11."Stop" T11."MainProgram"] -> w2769
          tunnel: [w2776 w2922 w2994 w3003 w3014 w3034 w3064 w3547 w3618 w3633 w3645 w3762 w3770] -> w2763
          tunnel: w2767 -> [w2801 w2922 w2993 w3005 w3014 w3034 w3071 w3547 w3619 w3632 w3641 w3762 w3775]
          tunnel: [w2809 w2916 w2995 w3004 w3015 w3032 w3061 w3504 w3616 w3630 w3646 w3760 w3768] -> w2764
          tunnel: w2765 -> [w2809 w2916 w2995 w3004 w3015 w3032 w3061 w3504 w3616 w3630 _ w3760 w3768]
          tunnel: w2762 -> [w2803 w2928 w2989 w3000 w3011 w3031 w3069 w3531 w3615 w3629 w3649 w3759 w3773]
          tunnel: w2761 -> [w2799 w2927 w2990 w3001 w3012 w3030 w3043 w3530 w3614 w3628 w3648 w3758 w3766]
          tunnel: [w2800 w2927 w2990 w3001 w3012 w3030 w3043 w3530 w3614 w3628 w3648 w3758 w3766] -> w2760
          tunnel: [w2802 w2928 w2989 w3000 w3011 w3031 w3069 w3531 w3615 w3629 w3649 w3759 w3773] -> w2759
          tunnel: w2758 -> [w2797 w2926 w2988 w2999 w3010 w3029 w3068 w3529 w3613 w3627 w3647 w3757 w3772]
          tunnel: [w2797 w2926 w2988 w2999 w3010 w3029 w3063 w3529 w3613 w3627 w3647 w3757 w3772] -> w2757
          tunnel: w2755 -> [_ _ _ _ _ _ _ w3475 _ _ _ _ _]
          tunnel: w2754 -> [w2798 w2925 w2987 w2998 w3009 w3027 w3059 w3508 w3612 w3626 w3643 w3756 w3771]
          tunnel: [w2798 w2925 w2987 w2998 w3009 w3027 w3059 w3507 w3612 w3626 w3643 w3756 w3771] -> w2753
          tunnel: w2752 -> [_ w2923 _ _ _ _ _ w3506 _ _ _ _ _]
          tunnel: w2751 -> [_ w2915 _ _ _ _ _ _ _ _ _ _ _]
          tunnel: w2750 -> [_ _ _ _ _ _ _ _ w3611 _ _ _ _]
          tunnel: w2749 -> [w2774 w2896 w2986 w2997 w3008 w3024 w3042 w3477 w3609 w3625 w3638 w3755 w3764]
          tunnel: [w2773 w2896 w2986 w2997 w3008 w3024 w3042 w3477 w3609 w3625 w3638 w3755 w3764] -> w2748
          tunnel: w2747 -> [w2772 w2895 w2985 w2996 w3007 w3023 w3041 w3465 w3608 w3624 w3637 w3754 w3763]
          tunnel: [w2771 w2895 w2985 w2996 w3007 w3023 w3041 w3465 w3608 w3624 w3637 w3754 w3763] -> w2746
          tunnel: w2745 -> [_ _ _ _ _ _ _ w3464 _ _ _ _ _]
          event Timeout {
            n956 = event-data() -> ()  [unwired: 1 in, 3 out]
            n957 = property on="5.4.0" class="Bool (strict)"() -> ("Value"=w2770:bool)  [unwired: 2 in, 2 out]
            n958 = property class="Clust (strict)"(reference=w2799, error in=w2801) -> (reference out=w2800:refnum<vi>, error out=w2775:errorcluster, "Value"=w2806:T28)
            n959 = case shown="True" w2770 {
              tunnel: w2775 -> [_ w2814]
              tunnel: w2774 -> [_ w2813]
              tunnel: [0 w2812] -> w2773
              frame False {
              }
              frame True {
                n960 = case shown="12" w2813 {
                  selector: w2813 -> [w2816 _]
                  tunnel: w2814 -> [_ w2820]
                  tunnel: [w2815 0] -> w2812
                  frame 0, Default {
                    n961 = Increment(x=w2816) -> (x+1=w2815:i32)
                  }
                  frame 12 {
                    n962 = property on="CurrentTest" class="Enum (strict)"() -> ("Value"=w2821:T1)  [unwired: 2 in, 2 out]
                    n963 = case shown="\"Temp Control\"" w2821 {
                      tunnel: [TRUE TRUE TRUE TRUE TRUE TRUE FALSE TRUE TRUE TRUE] -> w2819
                      tunnel: [u16 0 u16 0 u16 0 w2830 w2832 u16 0 u16 0 w2838 u16 0 u16 0] -> w2818
                      frame "Auxiliary", Default {
                      }
                      frame "Temp Sens Cal" {
                      }
                      frame "Com Test" {
                      }
                      frame "Enable Test" {
                        n964 = property on="VenableSpeed" class="DigNum (strict)"() -> ("Value"=w2830:u16)  [unwired: 2 in, 2 out]
                      }
                      frame "Speed Command" {
                        n965 = property on="SpeedCommandSpeed" class="DigNum (strict)"() -> ("Value"=w2832:u16)  [unwired: 2 in, 2 out]
                      }
                      frame "Stop Time" {
                      }
                      frame "Temp Control" {
                      }
                      frame "Burn in" {
                        n966 = property on="BurnInSpeed" class="DigNum (strict)"() -> ("Value"=w2838:u16)  [unwired: 2 in, 2 out]
                      }
                      frame "Visual Inspec" {
                      }
                      frame "Empty" {
                      }
                    }
                    n967 = control-ref of="Config_CANAT"() -> (w2823:refnum<vi>)
                    n968 = control-ref of="UUT"() -> (w2822:refnum<vi>)
                    n969 = call "CANSendMotorSpeed.vi"("Remote"=w2819, "error in (no error)"=w2820, "Motor Speed RPM"=w2818, "UUT"=w2822, "CAN Cluster in"=w2823) -> ()  [unwired: 6 in, 1 out]
                  }
                }
              }
            }
            n970 = Unbundle By Name(w2806) -> ("DevType"=w2807:T26, "CanIndex"=w2805:T27)
            n971 = property on="ClosePanel" class="Bool (strict)"("Value"=FALSE ("ClosePanel")) -> ()  [unwired: 2 in, 2 out]
            n972 = call "VCI_Receive.vi"("CANIndex"=w2805, "DevIndex"=u32 0, "DevType"=w2807) -> ("Recieve"=w2804:T29[])  [unwired: 3 in, 5 out]
            n973 = Empty Array?(array=w2804) -> (empty?=w2792:bool)
            n974 = case shown="False" w2792 {
              tunnel: w2805 -> [w2857 _]
              tunnel: w2800 -> [w2855 _]
              tunnel: w2803 -> [w2854 w2894]
              tunnel: w2775 -> [w2853 w2893]
              tunnel: w2804 -> [w2858 _]
              tunnel: [w2848 w2893] -> w2776
              tunnel: [w2847 w2894] -> w2802
              tunnel: [TRUE w2888] -> w2790
              tunnel: w2772 -> [_ w2892]
              tunnel: [0 w2891] -> w2771
              frame False {
                n975 = call "Demo_MakeDispBuff.vi"("Channel"=w2857, "Type"=enum16{"接收", "发送"}."接收", "OBJs"=w2858) -> ("Buffer"=w2856:T30)
                n976 = for {
                  N: 3 -> [_]
                  tunnel: w2856 -> [w2872]
                  tunnel: w2855 -> [w2871]
                  tunnel: w2854 -> [w2862]
                  tunnel: w2853 -> [w2861]
                  tunnel: [w2864] -> w2851 mode=indexing
                  tunnel: [w2862] -> w2850
                  tunnel: [w2861] -> w2849
                  i -> [w2860]
                  n977 = property class="Clust (strict)"(reference=w2871) -> ("Value"=w2869:T28)  [unwired: 1 in, 2 out]
                  n978 = Index Array(array=w2872, index=w2860) -> (element=w2865:T31)
                  n979 = Unbundle By Name(w2865) -> ("Channel"=w2867:T2, "VCI_CAN_OBJ"=w2870:T29)  [unwired: 2 out]
                  n980 = Unbundle By Name(w2869) -> ("CanIndex"=w2868:T27)
                  n981 = Equal?(x=w2868, y=w2867) -> (x = y?=w2866:bool)
                  n982 = case shown="True" w2866 {
                    tunnel: w2870 -> [_ w2883]
                    tunnel: [w2873 w2879] -> w2864
                    tunnel: T24 {"ID"=0, "MSGTYPE"=0, "LEN"=0, "aDATA"=[]} ("Msg") -> [w2873 w2878]
                    frame False {
                    }
                    frame True {
                      n983 = Unbundle By Name(w2883) -> ("ID"=w2877:u32, "DataLen"=w2882:u8, "Data"=w2880:u8[])
                      n984 = Bundle By Name(cluster=w2878, "ID"=w2877, "MSGTYPE"=u8 0, "LEN"=w2882, "aDATA"=w2880) -> (w2879:T24)
                      n985 = Unbundle By Name(w2879) -> ("ID"=w2875:u32)
                      n986 = Split Number(x=w2875) -> (lo(x)=w2876:u16)  [unwired: 1 out]
                      n987 = Split Number(x=w2876) -> (lo(x)=w2874:u8)  [unwired: 1 out]
                      n988 = case shown="63" w2874 {
                        tunnel: ["EBAY 5F" "" "AHU 3F" "AHU 2F"] -> _
                        frame 95 {
                        }
                        frame Default {
                        }
                        frame 63 {
                        }
                        frame 47 {
                        }
                      }
                    }
                  }
                }
                n989 = Enqueue Element(queue=w2850, element=w2851, error in (no error)=w2849) -> (queue out=w2847:refnum<queue>, error out=w2848:errorcluster)  [unwired: 2 out]
              }
              frame True {
                n990 = Increment(x=w2892) -> (x+1=w2891:i32)
                n991 = Greater Or Equal?(x=w2891, y=7) -> (x >= y?=w2889:bool)
                n992 = Not(x=w2889) -> (.not. x?=w2888:bool)
              }
            }
            n993 = property on="CAN Status" class="Bool (strict)"("Value"=w2790) -> ()  [unwired: 2 in, 2 out]
            n994 = control-ref of="ATR"() -> (w2791:refnum<vi>)
            n995 = call <vilib>:"Application Directory.vi"() -> ("Application Directory"=w2784:path)
            n996 = call "PassFailUUT (SubVI).vi"("error in (no error)"=w2776, "Table in"=w2791) -> ("PassFaileUUTresult"=w2780:bool)  [unwired: 7 in, 2 out]
            n997 = Select(t="PASS" ("name or relative path"), s=w2780, f="FAIL" ("name or relative path")) -> (s? t:f=w2777:string)
            n998 = Build Path(base path=w2784, name or relative path="data\\TestResult.ini") -> (appended path=w2788:path)
            n999 = property on="Test Failed" class="Bool (strict)"("Value"=w2780) -> ()  [unwired: 2 in, 2 out]
            n1000 = call <vilib>:"Open Config Data.vi"("configuration file path"=w2788) -> ("error out"=w2786:errorcluster, "refnum"=w2787:T12)  [unwired: 2 in, 7 out]
            n1001 = property on="Automation" class="Bool (strict)"() -> ("Value"=w2794:bool)  [unwired: 2 in, 2 out]
            n1002 = call-poly <vilib>:"Write Key.vi"("section"="Marvin", "error in (no error)"=w2786, "value"=w2777, "key"="Result", "refnum"=w2787) -> ("error out"=w2783:errorcluster, "refnum out"=w2782:T12)  [unwired: 4 in, 1 out]
            n1003 = property on="Start" class="Bool (strict)"() -> ("Value"=w2796:bool)  [unwired: 2 in, 2 out]
            n1004 = Or(x=w2794, y=w2796) -> (x .or. y?=w2795:bool)
            n1005 = call <vilib>:"Close Config Data.vi"("error in (no error)"=w2783, "refnum"=w2782) -> ()  [unwired: 8 in, 2 out]
            n1006 = case shown="False" w2795 {
              frame False {
                n1007 = property on="Pannel User Message" class="Str"("Value"="You can press start to execute(s) test(s).") -> ()  [unwired: 2 in, 2 out]
              }
              frame True {
              }
            }
          }
          event "SetSN": Value Change {
            n1008 = event-data() -> ()  [unwired: 1 in, 6 out]
            n1009 = property on="UUT" class="DigNum (strict)"() -> ("Value"=w2906:u8)  [unwired: 2 in, 2 out]
            n1010 = Equal?(x=w2906, y=u8 95) -> (x = y?=w2904:bool)
            n1011 = control-ref of="ATR"() -> (w2907:refnum<vi>)
            n1012 = Select(t=u8 50 ("y"), s=w2904, f=u8 36 ("y")) -> (s? t:f=w2899:u8)
            n1013 = property on="Current SN" class="DigNum (strict)"(error in=w2922) -> (error out=w2901:errorcluster, "Value"=w2921:i32)  [unwired: 1 in, 1 out]
            n1014 = call "PassFailUUT (SubVI).vi"("error in (no error)"=w2901, "Table in"=w2907) -> ("Total Pass"=w2900:u8)  [unwired: 7 in, 2 out]
            n1015 = Equal To 0?(x=w2921) -> (x = 0?=w2918:bool)
            n1016 = Equal?(x=w2921, y=-1) -> (x = y?=w2919:bool)
            n1017 = Equal?(x=w2900, y=w2899) -> (x = y?=w2898:bool)
            n1018 = Or(x=w2919, y=w2918) -> (x .or. y?=w2917:bool)
            n1019 = property on="CAN Status" class="Bool (strict)"() -> ("Value"=w2908:bool)  [unwired: 2 in, 2 out]
            n1020 = property on="Status" class="Bool (strict)"() -> ("Value"=w2913:bool)  [unwired: 2 in, 2 out]
            n1021 = And(x=w2913, y=w2908) -> (x .and. y?=w2909:bool)
            n1022 = case shown="True" w2909 {
              tunnel: w2923 -> [_ w2942]
              tunnel: w2917 -> [_ w2931]
              tunnel: w2916 -> [_ w2941]
              tunnel: w2915 -> [_ w2940]
              tunnel: [errorcluster {"status"=FALSE, "code"=0, "source"=""} ("error out") w2939] -> w2912
              tunnel: [w2929 w2938] -> w2914
              tunnel: w2898 -> [_ w2932]
              frame False {
                w2929 = FALSE ("Value")
                n1023 = property on="SetSN" class="Bool (strict)"("Value"=w2929) -> ()  [unwired: 2 in, 2 out]
                n1024 = call "Display Message to User10"() -> ()  [unwired: 10 in, 2 out]
              }
              frame True {
                n1025 = property on="Test Failed" class="Bool (strict)"() -> ("Value"=w2936:bool)  [unwired: 2 in, 2 out]
                n1026 = property on="Automation" class="Bool (strict)"() -> ("Value"=w2938:bool)  [unwired: 2 in, 2 out]
                n1027 = Not(x=w2936) -> (.not. x?=w2937:bool)
                n1028 = Select(t=w2937, s=w2938, f=w2940) -> (s? t:f=w2934:bool)
                n1029 = Or(x=w2932, y=w2934) -> (x .or. y?=w2933:bool)
                n1030 = And(x=w2931, y=w2933) -> (x .and. y?=w2935:bool)
                n1031 = case shown="True" w2935 {
                  tunnel: w2942 -> [_ w2973]
                  tunnel: w2941 -> [_ w2966]
                  tunnel: [w2944 w2958] -> w2939
                  tunnel: w2931 -> [w2943 _]
                  frame False {
                    n1032 = case shown="True" w2943 {
                      tunnel: [w2946 w2947] -> w2944
                      frame False {
                        n1033 = call "Display Message to User9"() -> ("error out"=w2946:errorcluster)  [unwired: 10 in, 1 out]
                      }
                      frame True {
                        n1034 = call "Display Message to User3"() -> ("error out"=w2947:errorcluster)  [unwired: 10 in, 1 out]
                      }
                    }
                    n1035 = property on="Automation" class="Bool (strict)"(error in=w2944, "Value"=FALSE ("Automation")) -> ()  [unwired: 1 in, 2 out]
                  }
                  frame True {
                    w2965 = FALSE ("SetSN")
                    n1036 = property on="Next SN" class="DigNum (strict)"() -> ("Value"=w2949:i32)  [unwired: 2 in, 2 out]
                    n1037 = property on="VISA Tester" class="VISAName"() -> ("Value"=w2956:refnum<visa-resource-name>)  [unwired: 2 in, 2 out]
                    n1038 = call "TesterOption (SubVI).vi"("2 Options"=FALSE, "On/Off"=FALSE, "Tester Option"=T13."Venable", "VISA Refnum in"=w2956) -> ("error out"=w2951:errorcluster)  [unwired: 6 in, 1 out]
                    n1039 = call <vilib>:"Clear Errors.vi"("error in (no error)"=w2951) -> ("error out"=w2952:errorcluster)  [unwired: 5 in, 1 out]
                    n1040 = Number To Decimal String(number=w2949) -> (decimal integer string=w2950:string)  [unwired: 1 in]
                    "UUT SN Report" <- w2950
                    n1041 = Search and Replace String(input string="EP=1\r\nSN=0\r\n" ("write buffer"), search string="0", replace string=w2950) -> (result string=w2968:string)  [unwired: 5 in, 3 out]
                    n1042 = call "SerialMarvinSendGet.vi"("error in (no error)"=w2952, "Clear Log"=FALSE, "write buffer"=w2968, "VISA resource name"=w2966) -> ("error out"=w2957:errorcluster)  [unwired: 6 in, 1 out]
                    n1043 = property on="UUT" class="DigNum (strict)"(error in=w2957) -> ("Value"=w2974:u8)  [unwired: 1 in, 2 out]
                    n1044 = case shown="47" w2974 {
                      tunnel: ["AHU R Serial Number" ("key") "AHU L Serial Number" ("key") "EBAY Serial Number" ("key")] -> w2977
                      tunnel: [2 2 1] -> w2948
                      frame 63, Default {
                      }
                      frame 47 {
                      }
                      frame 95 {
                      }
                    }
                    n1045 = call <vilib>:"Open Config Data.vi"("create file if necessary (T)"=FALSE, "configuration file path"=w2973) -> ("error out"=w2971:errorcluster, "refnum"=w2972:T12)  [unwired: 1 in, 7 out]
                    n1046 = call-poly <vilib>:"Write Key.vi"("section"="Marvin", "error in (no error)"=w2971, "value"=w2950, "key"=w2977, "refnum"=w2972) -> ("error out"=w2961:errorcluster, "refnum out"=w2960:T12)  [unwired: 4 in, 1 out]
                    n1047 = call <vilib>:"Close Config Data.vi"("error in (no error)"=w2961, "refnum"=w2960) -> ("error out"=w2959:errorcluster)  [unwired: 8 in, 1 out]
                    n1048 = property on="Current SN" class="DigNum (strict)"("Value"=w2949) -> ()  [unwired: 2 in, 2 out]
                    n1049 = property on="SetSN" class="Bool (strict)"(error in=w2959, "Value"=w2965) -> (error out=w2964:errorcluster)  [unwired: 1 in, 1 out]
                    n1050 = property on="Automation" class="Bool (strict)"(error in=w2964, "Value"=w2965) -> (error out=w2963:errorcluster)  [unwired: 1 in, 1 out]
                    n1051 = Add(x=w2949, y=w2948) -> (x+y=w2962:i32)
                    n1052 = property on="Next SN" class="DigNum (strict)"(error in=w2963, "Value"=w2962) -> (error out=w2958:errorcluster)  [unwired: 1 in, 1 out]
                  }
                }
              }
            }
            n1053 = call <vilib>:"Clear Errors.vi"("error in (no error)"=w2912) -> ("error out"=w2897:errorcluster)  [unwired: 5 in, 1 out]
            n1054 = property on="SetSN" class="Bool (strict)"(error in=w2897, "Value"=FALSE ("SetSN")) -> (error out=w2911:errorcluster)  [unwired: 1 in, 1 out]
            n1055 = case shown="True" w2914 {
              tunnel: w2911 -> [_ _]
              frame False {
              }
              frame True {
                w2984 = TRUE ("Value (Signaling)")
                n1056 = property on="Report" class="Bool (strict)"("Val(Sgnl)"=w2984, "Value"=w2984) -> ()  [unwired: 2 in, 2 out]
              }
            }
          }
          event "ATR": Mouse Enter {
            n1057 = event-data() -> ()  [unwired: 1 in, 4 out]
            n1058 = call-poly <vilib>:"Set Cursor.vi"("error in (no error)"=w2993, "icon"=u16 1) -> ("error out"=w2994:errorcluster)  [unwired: 8 in, 1 out]
          }
          event "ATR": Mouse Leave {
            n1059 = event-data() -> ()  [unwired: 1 in, 4 out]
            n1060 = call-poly <vilib>:"Set Cursor.vi"("error in (no error)"=w3005, "icon"=u16 0) -> ("error out"=w3003:errorcluster)  [unwired: 8 in, 1 out]
          }
          event "ATR": Mouse Down? {
            n1061 = event-data() -> ("Coords"=w3022:T32)  [unwired: 1 in, 4 out]
            n1062 = invoke on="ATR" class="Tbl (strict)" method="Point To Row Column"("Point"=w3022) -> ("InBounds"=w3018:bool, "CellPosition"=w3017:T22)  [unwired: 5 in, 4 out]
            n1063 = Greater Than 0?(x=w3017) -> (x > 0?=w3021:cluster{"Row":bool, "Column":bool})
            n1064 = Cluster To Array(cluster=w3021) -> (array=w3020:bool[])
            n1065 = Or Array Elements(Boolean array=w3020) -> (logical OR=w3019:bool)
            n1066 = Or(x=w3018, y=w3019) -> (x .or. y?=w3016:bool)
            n1067 = event-data("Discard?"=w3016) -> ()  [unwired: 1 in, 1 out]
          }
          event Panel Close? {
            n1068 = event-data() -> ("VIRef"=w3028:refnum<vi>)  [unwired: 1 in, 3 out]
            n1069 = Close Reference(reference=w3028) -> ()  [unwired: 1 in, 1 out]
            n1070 = disable-structure shown="Disabled" {
              frame Disabled {
                n1071 = property on="Stop Button" class="Bool (strict)"("Val(Sgnl)"=TRUE ("Stop Button"), "Value"=FALSE ("Stop Button")) -> ()  [unwired: 2 in, 2 out]
              }
              frame Enabled {
              }
            }
            n1072 = event-data("Discard?"=TRUE) -> ()  [unwired: 1 in, 1 out]
            "ClosePanel" <- TRUE ("ClosePanel")
          }
          event "Start": Value Change {
            w3060 = T18 [] items=["Auxiliary", "Temp Sens Cal", "Com Test", "Enable Test", "Speed Command", "Stop Time", "Temp Control", "Burn in", "Visual Inspec", "Empty"]
            n1073 = event-data() -> ()  [unwired: 1 in, 2 out]
            n1074 = property on="VISA Tester" class="VISAName"() -> ("Value"=w3058:refnum<visa-resource-name>)  [unwired: 2 in, 2 out]
            n1075 = property on="UUT" class="Str"(error in=w3071) -> (error out=w3054:errorcluster, "Value"=w3070:string)  [unwired: 1 in, 1 out]
            n1076 = control-ref of="Pannel User Message"() -> (w3051:refnum<vi>)
            n1077 = control-ref of="Motor Speed RPM"() -> (w3046:refnum<vi>)
            n1078 = call "TesterOption (SubVI).vi"("2 Options"=FALSE, "error in (no error)"=w3054, "On/Off"=FALSE, "Tester Option"=T13."Venable", "VISA Refnum in"=w3058) -> ("error out"=w3053:errorcluster)  [unwired: 5 in, 1 out]
            n1079 = control-ref of="Stop Burn-in"() -> (w3049:refnum<vi>)
            n1080 = control-ref of="Stop Button"() -> (w3050:refnum<vi>)
            n1081 = Select(t=enum16{"Stop", "Tests", "Bit test", "Start"}."Start", s=TRUE, f=enum16{"Stop", "Tests", "Bit test", "Start"}."Tests") -> (s? t:f=w3039:enum16{"Stop", "Tests", "Bit test", "Start"})
            n1082 = call "Write panel message (SubVI).vi"("Stop BurnIn"=w3049, 4:"rpm"=w3046, 5:"rpm"=FALSE ("rpm"), "PrintTime"=TRUE, "Stop"=w3050, "error in (no error)"=w3053, "Time to wait"=5.0, "Strin"="TESTER BIT TEST OPERATION IN PROCESS", "String in"=w3051) -> ("error out"=w3052:errorcluster)  [unwired: 2 in]
            n1083 = while {
              tunnel: w3070 -> [w3099]
              tunnel: [w3098] -> w3066
              tunnel: [w3097] -> w3065
              shift-right: [w3094] -> _
              shift-left: w3039 -> [w3096]
              tunnel: w3061 -> [w3095]
              tunnel: w3060 -> [w3093]
              tunnel: w3052 -> [w3078]
              tunnel: w3050 -> [w3087]
              tunnel: w3049 -> [w3086]
              tunnel: w3051 -> [w3085]
              tunnel: w3046 -> [w3084]
              tunnel: w3043 -> [w3077]
              stop <- w3092 stop-if-true
              n1084 = property class="Clust (strict)"(reference=w3077, error in=w3078) -> ("Value"=w3080:T28)  [unwired: 2 out]
              n1085 = Unbundle By Name(w3080) -> ("DevType"=w3082:T26, "CanIndex"=w3081:T27)
              n1086 = property on="VISA Tester" class="VISAName"() -> ("Value"=w3090:refnum<visa-resource-name>)  [unwired: 2 in, 2 out]
              n1087 = call "VCI_Receive.vi"("CANIndex"=w3081, "DevIndex"=u32 0, "DevType"=w3082) -> ("Recieve"=w3083:T29[])  [unwired: 3 in, 5 out]
              n1088 = Empty Array?(array=w3083) -> (empty?=w3076:bool)
              n1089 = Not(x=w3076) -> (.not. x?=w3075:bool)
              n1090 = property on="CAN Status" class="Bool (strict)"("Value"=w3075) -> (error out=w3074:errorcluster)  [unwired: 2 in, 1 out]
              n1091 = property on="CAN Status" class="Bool (strict)"(error in=w3074) -> (error out=w3073:errorcluster, "Value"=w3088:bool)  [unwired: 1 in, 1 out]
              n1092 = property on="Status" class="Bool (strict)"(error in=w3073) -> (error out=w3089:errorcluster, "Value"=w3091:bool)  [unwired: 1 in, 1 out]
              n1093 = case shown="\"Start\"" w3096 {
                tunnel: w3099 -> [_ w3115 w3291 _]
                tunnel: [w3104 w3114 w3315 w3423] -> w3098
                tunnel: [w3100 w3113 w3289 w3415] -> w3097
                tunnel: w3095 -> [_ _ w3302 w3428]
                tunnel: w3085 -> [_ _ _ w3427]
                tunnel: w3087 -> [_ _ _ w3426]
                tunnel: w3086 -> [_ _ _ w3425]
                tunnel: w3084 -> [_ _ _ w3424]
                tunnel: [w3103 w3112 w3294 w3419] -> w3094
                tunnel: w3093 -> [w3104 _ w3315 w3423]
                tunnel: [w3102 w3111 FALSE FALSE] -> w3092
                tunnel: w3091 -> [_ _ _ w3421]
                tunnel: w3090 -> [_ _ w3285 _]
                tunnel: w3089 -> [w3100 _ _ _]
                tunnel: w3088 -> [_ _ _ w3416]
                frame "Stop", Default {
                  n1094 = property on="Start" class="Bool (strict)"(error in=w3100, "Value"=FALSE ("Start")) -> ()  [unwired: 1 in, 2 out]
                  n1095 = flat-sequence {
                    tunnel: [enum16{"Stop", "Tests", "Bit test", "Start"}."Stop"] -> w3103
                    tunnel: w3100 -> [_]
                    tunnel: [TRUE] -> w3102
                    frame #0 {
                    }
                  }
                }
                frame "Tests" {
                  w3109 = FALSE ("Stop Burn-in")
                  w3110 = T21."Disabled and Grayed Out" ("Disabled")
                  n1096 = case shown="\"EBAY\"" w3115 {
                    tunnel: [w3131 w3180] -> w3114
                    tunnel: [w3130 w3179] -> w3113
                    tunnel: [w3119 w3167] -> w3107
                    frame "AHU", Default {
                      n1097 = call "Load Program Process AHU.vi"() -> ("Speed Command Test"=w3124:bool, "Enable Test"=w3125:bool, "Burn-in Test"=w3122:bool, "Auxiliary"=w3120:bool, "Temperature Sensor Calibration Test"=w3127:bool, "Communication Test"=w3126:bool, "Stop Time Test"=w3123:bool, "Visual Inspection"=w3121:bool, "OK"=w3128:bool, "Automation"=w3119:bool, "error out"=w3130:errorcluster)  [unwired: 8 in, 9 out]
                      n1098 = Or(x=w3128, y=w3119) -> (x .or. y?=w3129:bool)
                      n1099 = case shown="True" w3129 {
                        tunnel: [w3132 w3142] -> w3131
                        tunnel: w3119 -> [_ w3141]
                        tunnel: w3127 -> [_ w3140]
                        tunnel: w3126 -> [_ w3139]
                        tunnel: w3125 -> [_ w3138]
                        tunnel: w3124 -> [_ w3137]
                        tunnel: w3123 -> [_ w3136]
                        tunnel: w3122 -> [_ w3135]
                        tunnel: w3121 -> [_ w3134]
                        tunnel: w3120 -> [_ w3133]
                        frame False {
                          w3132 = T18 [] items=["Auxiliary", "Temp Sens Cal", "Com Test", "Enable Test", "Speed Command", "Stop Time", "Temp Control", "Burn in", "Visual Inspec", "Empty"]
                        }
                        frame True {
                          n1100 = case shown="False" w3141 {
                            tunnel: [w3165 w3166] -> w3142
                            tunnel: w3140 -> [w3147 _]
                            tunnel: w3139 -> [w3146 _]
                            tunnel: w3138 -> [w3148 _]
                            tunnel: w3137 -> [w3145 _]
                            tunnel: w3136 -> [w3144 _]
                            tunnel: w3135 -> [w3158 _]
                            tunnel: w3134 -> [w3143 _]
                            tunnel: w3133 -> [_ _]
                            frame False {
                              w3151 = T1."Empty" ("f")
                              n1101 = Select(t=T1."Com Test" ("f"), s=w3146, f=w3151) -> (s? t:f=w3157:T1)
                              n1102 = Select(t=T1."Temp Sens Cal" ("f"), s=w3147, f=w3151) -> (s? t:f=w3156:T1)
                              n1103 = Select(t=T1."Stop Time" ("f"), s=w3144, f=w3151) -> (s? t:f=w3155:T1)
                              n1104 = Select(t=T1."Enable Test" ("f"), s=w3148, f=w3151) -> (s? t:f=w3154:T1)
                              n1105 = Select(t=T1."Speed Command" ("f"), s=w3145, f=w3151) -> (s? t:f=w3153:T1)
                              n1106 = Select(t=T1."Burn in" ("f"), s=w3158, f=w3151) -> (s? t:f=w3152:T1)
                              n1107 = Select(t=T1."Visual Inspec" ("f"), s=w3143, f=w3151) -> (s? t:f=w3149:T1)
                              n1108 = Build Array(w3157, w3156, w3155, w3154, w3153, w3152, w3149) -> (w3165:T18)
                            }
                            frame True {
                              w3166 = T18 [enum."Com Test", enum."Temp Sens Cal", enum."Stop Time", enum."Enable Test", enum."Speed Command", enum."Burn in", enum."Visual Inspec"] items=["Auxiliary", "Temp Sens Cal", "Com Test", "Enable Test", "Speed Command", "Stop Time", "Temp Control", "Burn in", "Visual Inspec", "Empty"]
                            }
                          }
                        }
                      }
                    }
                    frame "EBAY" {
                      n1109 = call "Load Program Process EBAY.vi"() -> ("Speed Command Test"=w3173:bool, "Enable Test"=w3174:bool, "Burn-in Test"=w3171:bool, "Temperature Control Algorithm Test"=w3170:bool, "Auxiliary"=w3168:bool, "Temperature Sensor Calibration Test"=w3176:bool, "Communication Test"=w3175:bool, "Stop Time Test"=w3172:bool, "Visual Inspection"=w3169:bool, "OK"=w3177:bool, "Automation"=w3167:bool, "error out"=w3179:errorcluster)  [unwired: 8 in, 8 out]
                      n1110 = Or(x=w3177, y=w3167) -> (x .or. y?=w3178:bool)
                      n1111 = case shown="True" w3178 {
                        tunnel: [w3181 w3192] -> w3180
                        tunnel: w3167 -> [_ w3191]
                        tunnel: w3176 -> [_ w3190]
                        tunnel: w3175 -> [_ w3189]
                        tunnel: w3174 -> [_ w3188]
                        tunnel: w3173 -> [_ w3187]
                        tunnel: w3172 -> [_ w3186]
                        tunnel: w3171 -> [_ w3185]
                        tunnel: w3170 -> [_ w3184]
                        tunnel: w3169 -> [_ w3183]
                        tunnel: w3168 -> [_ w3182]
                        frame False {
                          w3181 = T18 [] items=["Auxiliary", "Temp Sens Cal", "Com Test", "Enable Test", "Speed Command", "Stop Time", "Temp Control", "Burn in", "Visual Inspec", "Empty"]
                        }
                        frame True {
                          n1112 = case shown="False" w3191 {
                            tunnel: [w3203 w3263] -> w3192
                            tunnel: w3190 -> [w3198 _]
                            tunnel: w3189 -> [w3197 _]
                            tunnel: w3188 -> [w3196 _]
                            tunnel: w3187 -> [w3195 _]
                            tunnel: w3186 -> [w3194 _]
                            tunnel: w3185 -> [w3200 _]
                            tunnel: w3184 -> [w3199 _]
                            tunnel: w3183 -> [w3202 _]
                            tunnel: w3182 -> [w3201 _]
                            frame False {
                              n1113 = property on="5.4.0" class="Bool (strict)"() -> ("Value"=w3193:bool)  [unwired: 2 in, 2 out]
                              n1114 = case shown="False" w3193 {
                                tunnel: [w3232 w3261] -> w3203
                                tunnel: w3202 -> [w3223 w3252]
                                tunnel: w3201 -> [w3214 w3243]
                                tunnel: w3200 -> [w3211 w3240]
                                tunnel: w3199 -> [w3210 w3239]
                                tunnel: w3198 -> [w3209 w3238]
                                tunnel: w3197 -> [w3208 w3237]
                                tunnel: w3196 -> [w3207 w3236]
                                tunnel: w3195 -> [w3206 w3235]
                                tunnel: w3194 -> [w3205 w3234]
                                frame False {
                                w3212 = T1."Empty" ("f")
                                n1115 = Select(t=T1."Com Test" ("f"), s=w3208, f=w3212) -> (s? t:f=w3222:T1)
                                n1116 = Select(t=T1."Temp Sens Cal" ("f"), s=w3209, f=w3212) -> (s? t:f=w3221:T1)
                                n1117 = Select(t=T1."Stop Time" ("f"), s=w3205, f=w3212) -> (s? t:f=w3220:T1)
                                n1118 = Select(t=T1."Enable Test" ("f"), s=w3207, f=w3212) -> (s? t:f=w3219:T1)
                                n1119 = Select(t=T1."Speed Command" ("f"), s=w3206, f=w3212) -> (s? t:f=w3218:T1)
                                n1120 = Select(t=T1."Temp Control" ("f"), s=w3210, f=w3212) -> (s? t:f=w3217:T1)
                                n1121 = Select(t=T1."Burn in" ("f"), s=w3211, f=w3212) -> (s? t:f=w3216:T1)
                                n1122 = Select(t=T1."Visual Inspec" ("f"), s=w3223, f=w3212) -> (s? t:f=w3215:T1)
                                n1123 = Select(t=T1."Auxiliary" ("f"), s=w3214, f=w3212) -> (s? t:f=w3204:T1)
                                n1124 = Build Array(w3222, w3221, w3220, w3219, w3218, w3217, w3216, w3204, w3215) -> (w3232:T18)
                                }
                                frame True {
                                w3241 = T1."Empty" ("f")
                                n1125 = Select(t=T1."Com Test" ("f"), s=w3237, f=w3241) -> (s? t:f=w3251:T1)
                                n1126 = Select(t=T1."Temp Sens Cal" ("f"), s=w3238, f=w3241) -> (s? t:f=w3250:T1)
                                n1127 = Select(t=T1."Stop Time" ("f"), s=w3234, f=w3241) -> (s? t:f=w3249:T1)
                                n1128 = Select(t=T1."Enable Test" ("f"), s=w3236, f=w3241) -> (s? t:f=w3248:T1)
                                n1129 = Select(t=T1."Speed Command" ("f"), s=w3235, f=w3241) -> (s? t:f=w3247:T1)
                                n1130 = Select(t=T1."Temp Control" ("f"), s=w3239, f=w3241) -> (s? t:f=w3246:T1)
                                n1131 = Select(t=T1."Burn in" ("f"), s=w3240, f=w3241) -> (s? t:f=w3245:T1)
                                n1132 = Select(t=T1."Visual Inspec" ("f"), s=w3252, f=w3241) -> (s? t:f=w3244:T1)
                                n1133 = Select(t=T1."Auxiliary" ("f"), s=w3243, f=w3241) -> (s? t:f=w3233:T1)
                                n1134 = Build Array(w3251, w3233, w3250, w3249, w3248, w3247, w3246, w3245, w3244) -> (w3261:T18)
                                }
                              }
                            }
                            frame True {
                              n1135 = property on="5.4.0" class="Bool (strict)"() -> ("Value"=w3262:bool)  [unwired: 2 in, 2 out]
                              n1136 = case shown="False" w3262 {
                                tunnel: [w3264 w3265] -> w3263
                                frame False {
                                w3264 = T18 [enum."Com Test", enum."Temp Sens Cal", enum."Stop Time", enum."Enable Test", enum."Speed Command", enum."Temp Control", enum."Burn in", enum."Auxiliary", enum."Visual Inspec"] items=["Auxiliary", "Temp Sens Cal", "Com Test", "Enable Test", "Speed Command", "Stop Time", "Temp Control", "Burn in", "Visual Inspec", "Empty"]
                                }
                                frame True {
                                w3265 = T18 [enum."Com Test", enum."Auxiliary", enum."Temp Sens Cal", enum."Stop Time", enum."Enable Test", enum."Speed Command", enum."Temp Control", enum."Burn in", enum."Visual Inspec"] items=["Auxiliary", "Temp Sens Cal", "Com Test", "Enable Test", "Speed Command", "Stop Time", "Temp Control", "Burn in", "Visual Inspec", "Empty"]
                                }
                              }
                            }
                          }
                        }
                      }
                    }
                  }
                  "Automation" <- w3107
                  n1137 = control-ref of="ATR"() -> (w3108:refnum<vi>)
                  n1138 = flat-sequence {
                    tunnel: [enum16{"Stop", "Tests", "Bit test", "Start"}."Tests"] -> w3112
                    tunnel: [TRUE] -> w3111
                    frame #0 {
                    }
                  }
                  n1139 = case shown="True" w3107 {
                    tunnel: w3108 -> [_ w3116]
                    frame False {
                    }
                    frame True {
                      n1140 = call "ResetTable Result (SubVI).vi"("Table in"=w3116) -> ()  [unwired: 11 in]
                    }
                  }
                  n1141 = property on="Stop Button" class="Bool (strict)"("Value"=w3109) -> ()  [unwired: 2 in, 2 out]
                  n1142 = property on="Stop Burn-in" class="Bool (strict)"("Value"=w3109) -> ()  [unwired: 2 in, 2 out]
                  n1143 = property on="Start" class="Bool (strict)"("DisabledEnum"=w3110) -> ()  [unwired: 2 in, 2 out]
                  n1144 = property on="Report" class="Bool (strict)"("DisabledEnum"=w3110) -> ()  [unwired: 2 in, 2 out]
                }
                frame "Bit test" {
                  # "Stop"
                  n1145 = call "SerialMarvinSendGet.vi"("write buffer"="TA[1]\r\n", "VISA resource name"=w3302) -> ("error out"=w3276:errorcluster, "read buffer"=w3312:string)  [unwired: 8 in]
                  n1146 = Fract/Exp String To Number(string=w3312) -> (number=w3275:dbl)  [unwired: 3 in, 1 out]
                  n1147 = call "TAs StartTest (SubVI).vi"("error in"=w3276, "Numeric"=w3275, "Enum"=enum16{"TA3", "TA2", "TA1"}."TA1") -> ("error out"=w3274:errorcluster, "String Out"=w3273:string, "Result"=w3272:bool)  [unwired: 6 in]
                  n1148 = call "TesterOption (SubVI).vi"("On/Off 2"=FALSE, "Tester Option 2"=T13."Venable", "2 Options"=TRUE, "error in (no error)"=w3274, "On/Off"=TRUE, "Tester Option"=T13."25C", "VISA Refnum in"=w3285) -> ("error out"=w3304:errorcluster)  [unwired: 3 in, 1 out]
                  n1149 = call "Time Delay5"("error in (no error)"=w3304) -> ("error out"=w3303:errorcluster)  [unwired: 10 in]
                  n1150 = call "SerialMarvinSendGet.vi"("error in (no error)"=w3303, "write buffer"="TA[2]\r\n", "VISA resource name"=w3302) -> ("error out"=w3270:errorcluster, "read buffer"=w3306:string)  [unwired: 7 in]
                  n1151 = Fract/Exp String To Number(string=w3306) -> (number=w3269:dbl)  [unwired: 3 in, 1 out]
                  n1152 = call "TAs StartTest (SubVI).vi"("error in"=w3270, "Numeric"=w3269, "Enum"=enum16{"TA3", "TA2", "TA1"}."TA2") -> ("error out"=w3268:errorcluster, "String Out"=w3267:string, "Result"=w3266:bool)  [unwired: 6 in]
                  n1153 = call "GetADCTester (SubVI).vi"("error in (no error)"=w3268, "GetADCTester"=T15."Term1", "TimeToGet"=5, "VISA Refnum in"=w3285) -> ("error out"=w3284:errorcluster, "ADCValOutput Single"=w3282:dbl)  [unwired: 5 in, 1 out]
                  n1154 = case shown="\"EBAY\"" w3291 {
                    tunnel: w3285 -> [w3345 _ w3377]
                    tunnel: w3302 -> [_ _ w3380]
                    tunnel: w3284 -> [w3346 w3363 w3379]
                    tunnel: [w3339 w3363 w3376] -> w3293
                    tunnel: [w3336 "" w3373] -> w3299
                    tunnel: [w3335 bool[] [] w3372] -> w3283
                    frame "AHU" {
                      n1155 = call "TesterOption (SubVI).vi"("On/Off 2"=FALSE, "Tester Option 2"=T13."Venable", "2 Options"=TRUE, "error in (no error)"=w3346, "On/Off"=TRUE, "Tester Option"=T13."K17", "VISA Refnum in"=w3345) -> ("error out"=w3348:errorcluster)  [unwired: 3 in, 1 out]
                      n1156 = call "Time Delay7"("error in (no error)"=w3348) -> ("error out"=w3347:errorcluster)  [unwired: 10 in]
                      n1157 = call "GetADCTester (SubVI).vi"("error in (no error)"=w3347, "GetADCTester"=T15."Current", "TimeToGet"=5, "VISA Refnum in"=w3345) -> ("error out"=w3339:errorcluster, "ADCValOutput Single"=w3341:dbl)  [unwired: 5 in, 1 out]
                      n1158 = Less Or Equal?(x=w3341, y=10.0) -> (x <= y?=w3340:bool)
                      n1159 = Build Array(w3340) -> (w3335:bool[])
                      n1160 = for {
                        tunnel: w3335 -> [w3360] mode=indexing
                        tunnel: string[] ["Current sensor not connected!"] -> [w3357] mode=indexing
                        shift-right: [w3358] -> w3336
                        shift-left: "" -> [w3355]
                        n1161 = Concatenate Strings(w3357, "\r\n") -> (w3354:string)
                        n1162 = Select(t=w3355, s=w3360, f=w3354) -> (s? t:f=w3359:string)
                        n1163 = Concatenate Strings(w3355, w3359) -> (w3358:string)
                      }
                    }
                    frame Default {
                    }
                    frame "EBAY" {
                      w3378 = T33 [enum."Fan", enum."Current"] items=["Term1", "Term2", "Current", "Fan", "TempCPU"]
                      n1164 = call "TesterOption (SubVI).vi"("On/Off 2"=FALSE, "Tester Option 2"=T13."Venable", "2 Options"=TRUE, "error in (no error)"=w3379, "On/Off"=TRUE, "Tester Option"=T13."K17", "VISA Refnum in"=w3377) -> ("error out"=w3382:errorcluster)  [unwired: 3 in, 1 out]
                      n1165 = call "Time Delay6"("error in (no error)"=w3382) -> ("error out"=w3381:errorcluster)  [unwired: 10 in]
                      n1166 = call "SerialMarvinSendGet.vi"("error in (no error)"=w3381, "write buffer"="TA[3]\r\n", "VISA resource name"=w3380) -> ("error out"=w3367:errorcluster, "read buffer"=w3384:string)  [unwired: 7 in]
                      n1167 = Fract/Exp String To Number(string=w3384) -> (number=w3368:dbl)  [unwired: 3 in, 1 out]
                      n1168 = call "TAs StartTest (SubVI).vi"("error in"=w3367, "Numeric"=w3368, "Enum"=enum16{"TA3", "TA2", "TA1"}."TA3") -> ("error out"=w3364:errorcluster, "String Out"=w3366:string, "Result"=w3365:bool)  [unwired: 6 in]
                      n1169 = for {
                        tunnel: w3378 -> [w3407] mode=indexing
                        tunnel: w3377 -> [w3406]
                        tunnel: w3364 -> [w3404]
                        tunnel: [w3403] -> w3376
                        tunnel: [w3400] -> w3375 mode=indexing
                        i -> [w3401]
                        n1170 = call "GetADCTester (SubVI).vi"("error in (no error)"=w3404, "GetADCTester"=w3407, "TimeToGet"=5, "VISA Refnum in"=w3406) -> ("error out"=w3403:errorcluster, "ADCValOutput Single"=w3402:dbl)  [unwired: 5 in, 1 out]
                        n1171 = case shown="0" w3401 {
                          tunnel: w3402 -> [w3410 w3413 _]
                          tunnel: [w3408 w3411 FALSE] -> w3400
                          frame 1 {
                            n1172 = Less Or Equal?(x=w3410, y=10.0) -> (x <= y?=w3408:bool)
                          }
                          frame 0 {
                            n1173 = Greater Or Equal?(x=w3413, y=2200.0) -> (x >= y?=w3411:bool)
                          }
                          frame Default {
                          }
                        }
                      }
                      n1174 = Build Array (concatenate)(w3365, w3375) -> (w3372:bool[])
                      n1175 = Build Array (concatenate)(w3366, string[] ["AUX Fan not connected!", "Current sensor not connected!"]) -> (w3370:string[])
                      n1176 = for {
                        tunnel: w3372 -> [w3390] mode=indexing
                        tunnel: w3370 -> [w3393] mode=indexing
                        shift-right: [w3395] -> w3373
                        shift-left: "" -> [w3394]
                        n1177 = Concatenate Strings(w3393, "\r\n") -> (w3391:string)
                        n1178 = case shown="False" w3390 {
                          tunnel: [w3398 w3399] -> w3395
                          tunnel: w3394 -> [w3397 w3399]
                          tunnel: w3391 -> [w3396 _]
                          frame False {
                            n1179 = Concatenate Strings(w3397, w3396) -> (w3398:string)
                          }
                          frame True {
                          }
                        }
                      }
                    }
                  }
                  n1180 = Less Or Equal?(x=w3282, y=100.0) -> (x <= y?=w3280:bool)
                  n1181 = Build Array(w3273, w3267, "Failure - check 28V or GND signals. Pin28 or Pin2") -> (w3279:string[])
                  n1182 = Build Array(w3272, w3266, w3280) -> (w3298:bool[])
                  n1183 = for {
                    tunnel: w3298 -> [w3324] mode=indexing
                    tunnel: w3279 -> [w3328] mode=indexing
                    shift-right: [w3330] -> w3300
                    shift-left: "" -> [w3329]
                    tunnel: w3293 -> [w3325]
                    tunnel: [w3325] -> w3292
                    n1184 = Concatenate Strings(w3328, "\r\n") -> (w3326:string)
                    n1185 = case shown="False" w3324 {
                      tunnel: [w3333 w3334] -> w3330
                      tunnel: w3329 -> [w3332 w3334]
                      tunnel: w3326 -> [w3331 _]
                      frame False {
                        n1186 = Concatenate Strings(w3332, w3331) -> (w3333:string)
                      }
                      frame True {
                      }
                    }
                  }
                  n1187 = Build Array (concatenate)(w3298, w3283) -> (w3297:bool[])
                  n1188 = And Array Elements(Boolean array=w3297) -> (logical AND=w3288:bool)
                  n1189 = case shown="False" w3288 {
                    tunnel: w3300 -> [w3322 _]
                    tunnel: w3299 -> [w3321 _]
                    tunnel: w3292 -> [w3319 w3323]
                    tunnel: [w3319 w3323] -> w3290
                    frame False {
                      n1190 = Concatenate Strings(w3322, w3321) -> (w3320:string)
                      n1191 = One Button Dialog(message=w3320) -> ()  [unwired: 1 in, 1 out]
                    }
                    frame True {
                    }
                  }
                  n1192 = case shown="False" w3288 {
                    tunnel: w3290 -> [w3317 w3318]
                    tunnel: [w3316 w3318] -> w3289
                    frame False {
                      n1193 = call "Display Message to User6"("error in (no error)"=w3317) -> ("error out"=w3316:errorcluster)  [unwired: 9 in, 1 out]
                    }
                    frame True {
                    }
                  }
                  n1194 = Select(t=enum16{"Stop", "Tests", "Bit test", "Start"}."Tests", s=w3288, f=enum16{"Stop", "Tests", "Bit test", "Start"}."Stop") -> (s? t:f=w3294:enum16{"Stop", "Tests", "Bit test", "Start"})
                }
                frame "Start" {
                  n1195 = And(x=w3416, y=w3421) -> (x .and. y?=w3417:bool)
                  n1196 = case shown="True" w3417 {
                    tunnel: w3428 -> [_ w3456]
                    tunnel: w3427 -> [_ w3448]
                    tunnel: w3426 -> [_ w3444]
                    tunnel: w3425 -> [_ w3442]
                    tunnel: w3424 -> [_ w3441]
                    tunnel: [FALSE w3437] -> w3420
                    tunnel: [w3434 w3440] -> w3415
                    tunnel: [FALSE TRUE] -> w3418
                    frame False {
                      n1197 = call "Display Message to User5"() -> ("error out"=w3434:errorcluster)  [unwired: 10 in, 1 out]
                    }
                    frame True {
                      n1198 = property on="VISA Tester" class="VISAName"() -> (error out=w3455:errorcluster, "Value"=w3454:refnum<visa-resource-name>)  [unwired: 2 in, 1 out]
                      n1199 = property on="UUT SoftwareVer" class="Str"() -> ("Value"=w3435:string)  [unwired: 2 in, 2 out]
                      n1200 = call "TesterOption (SubVI).vi"("2 Options"=FALSE, "error in (no error)"=w3455, "On/Off"=FALSE, "Tester Option"=T13."Venable", "VISA Refnum in"=w3454) -> ("error out"=w3450:errorcluster)  [unwired: 5 in, 1 out]
                      n1201 = call "Write panel message (SubVI).vi"("Stop BurnIn"=w3442, 4:"rpm"=w3441, 5:"rpm"=FALSE ("rpm"), "PrintTime"=FALSE, "Stop"=w3444, "error in (no error)"=w3450, "Time to wait"=3.0, "Strin"="TESTER BIT TEST OPERATION IN PROCESS\nPlease wait...", "String in"=w3448) -> ("error out"=w3449:errorcluster)  [unwired: 2 in]
                      n1202 = call "SerialMarvinSendGet.vi"("error in (no error)"=w3449, "write buffer"="VR\r\n", "VISA resource name"=w3456) -> ("error out"=w3440:errorcluster, "read buffer"=w3436:string)  [unwired: 7 in]
                      n1203 = Equal?(x=w3436, y=w3435) -> (x = y?=w3438:bool)
                      n1204 = case shown="False" w3438 {
                        selector: w3438 -> [_ w3463]
                        tunnel: [w3461 w3463] -> w3437
                        tunnel: w3436 -> [w3462 _]
                        tunnel: w3435 -> [w3459 _]
                        frame False {
                          n1205 = property on="UUT SoftwareVer2" class="Str"() -> ("Value"=w3458:string)  [unwired: 2 in, 2 out]
                          n1206 = Equal?(x=w3462, y=w3458) -> (x = y?=w3461:bool)
                          n1207 = Select(t=w3458, s=w3461, f=w3459) -> (s? t:f=w3460:string)
                          n1208 = property on="UUT SoftwareVer" class="Str"("Value"=w3460) -> ()  [unwired: 2 in, 2 out]
                        }
                        frame True {
                        }
                      }
                    }
                  }
                  n1209 = case shown="True" w3420 {
                    tunnel: [enum16{"Stop", "Tests", "Bit test", "Start"}."Stop" enum16{"Stop", "Tests", "Bit test", "Start"}."Bit test"] -> w3419
                    tunnel: w3418 -> [w3429 _]
                    frame False {
                      n1210 = case shown="True" w3429 {
                        frame False {
                        }
                        frame True {
                          n1211 = call "Display Message to User4"() -> ()  [unwired: 10 in, 2 out]
                        }
                      }
                    }
                    frame True {
                    }
                  }
                }
              }
            }
            n1212 = Bundle By Name(cluster=T9 {"VISA"="COM1", "Array Test"=[]}, "VISA"=w3061, "Array Test"=w3066) -> (w3062:T9)
            n1213 = Enqueue Element(queue=w3068, element=w3062, error in (no error)=w3065) -> (queue out=w3063:refnum<queue>, error out=w3064:errorcluster)  [unwired: 2 out]
          }
          event "Report", "Stop Button": Value Change {
            w3479 = T34 1 items=["User Home"=0, "User Desktop"=1, "User Documents"=2, "User Application Data"=3, "User Preferences"=4, "User Temporary"=5, "Public Documents"=6, "Public Application Data"=7, "Public Preferences"=8, "Public Cache"=13, "System Core Libraries"=9, "System Installed Libraries"=10, "Application Files"=11, "Boot Volume Root"=12] ("system directory type")
            w3511 = "Marvin" ("section")
            n1214 = event-data() -> ("CtlRef"=w3503:refnum<vi>)  [unwired: 1 in]
            n1215 = local read "UUT"() -> (w3476:string)
            n1216 = call <vilib>:"Get System Directory.vi"("system directory type"=w3479) -> ("system directory"=w3478:path)  [unwired: 10 in]
            n1217 = Build Path(base path=w3478, name or relative path="MarvinReports") -> (appended path=w3540:path)
            n1218 = property on="CAN Status" class="Bool (strict)"() -> ("Value"=w3482:bool)  [unwired: 2 in, 2 out]
            n1219 = property on="Status" class="Bool (strict)"() -> ("Value"=w3483:bool)  [unwired: 2 in, 2 out]
            n1220 = case shown="\"AHU\"" w3476 {
              tunnel: ["REV EBAY" ("key") "REV AHU" ("key")] -> w3509
              frame "EBAY", Default {
              }
              frame "AHU" {
              }
            }
            n1221 = call <vilib>:"Check if File or Folder Exists.vi"("path"=w3540) -> ("error out"=w3538:errorcluster, "file or folder exists?"=w3541:bool, "dup path"=w3539:path)  [unwired: 8 in]
            n1222 = And(x=w3483, y=w3482) -> (x .and. y?=w3484:bool)
            n1223 = case shown="False" w3541 {
              tunnel: w3538 -> [w3605 w3606]
              tunnel: w3539 -> [w3604 w3607]
              tunnel: [w3603 w3607] -> w3481
              tunnel: [w3602 w3606] -> w3543
              frame False {
                n1224 = Create Folder(path (use dialog)=w3604, error in=w3605) -> (created path=w3603:path, error out=w3602:errorcluster)  [unwired: 1 in, 1 out]
              }
              frame True {
              }
            }
            n1225 = case shown="True" w3484 {
              tunnel: [w3550 w3570] -> w3527
              tunnel: [w3550 w3569] -> w3470
              tunnel: w3504 -> [_ w3558]
              tunnel: [w3550 w3563] -> w3474
              tunnel: [w3550 w3562] -> w3472
              tunnel: [w3550 w3566] -> w3497
              tunnel: [w3550 w3565] -> w3473
              tunnel: [w3550 w3554] -> w3471
              frame False {
                (unwired) "47"
                (unwired) " 413-8005_47_AHU"
                (unwired) "413-8005-1-47"
                (unwired) "5.3.9" ("read buffer")
                (unwired) "95"
                (unwired) "414-8005_95_EBAY_"
                (unwired) "414-8005-95"
                (unwired) "414-8005-95   "
                w3550 = "N_A" ("read buffer")
                n1226 = disable-structure shown="Disabled" {
                  frame Disabled {
                    n1227 = call "Display Message to User7"() -> ()  [unwired: 10 in, 2 out]
                  }
                  frame Enabled {
                  }
                }
                n1228 = Decimal String To Number(string="1" ("Value")) -> (number=w3551:i32)  [unwired: 2 in, 1 out]
                n1229 = Number To Decimal String(number=w3551, width (-)=i16 4) -> ()  [unwired: 1 out]
              }
              frame True {
                n1230 = call "SerialMarvinSendGet.vi"("write buffer"="SN\r\n", "VISA resource name"=w3558) -> ("error out"=w3557:errorcluster, "read buffer"=w3560:string)  [unwired: 8 in]
                n1231 = call "Time Delay2"("error in (no error)"=w3557) -> ("error out"=w3556:errorcluster)  [unwired: 10 in]
                n1232 = Decimal String To Number(string=w3560) -> (number=w3559:i32)  [unwired: 2 in, 1 out]
                n1233 = Number To Decimal String(number=w3559, width (-)=i16 4) -> (decimal integer string=w3563:string)
                n1234 = call "SerialMarvinSendGet.vi"("error in (no error)"=w3556, "write buffer"="VR\r\n", "VISA resource name"=w3558) -> ("error out"=w3567:errorcluster, "read buffer"=w3562:string)  [unwired: 7 in]
                n1235 = property on="UUT" class="DigNum (strict)"(error in=w3567) -> ("Value"=w3555:u8)  [unwired: 1 in, 2 out]
                n1236 = call "SentenceFromFile (SubVI).vi"("UUT"=w3555) -> ("Sentence"=w3554:string)  [unwired: 9 in, 1 out]
                n1237 = case shown="95, Default" w3555 {
                  tunnel: ["414-8005_95_EBAY_" " 413-8005_47_AHU" " 413-8005_63_AHU"] -> w3570
                  tunnel: ["414-8005-95   " w3576 w3579] -> w3569
                  tunnel: ["414-8005-95" w3576 w3579] -> w3566
                  tunnel: ["95" "47" "63"] -> w3565
                  frame 95, Default {
                  }
                  frame 47 {
                    w3576 = "413-8005-1-47"
                    (unwired) "AHU-L (47) 413-8005-1"
                  }
                  frame 63 {
                    w3579 = "413-8005-2-63"
                    (unwired) "AHU-R (63) 413-8005-2"
                  }
                }
              }
            }
            n1238 = Get Date/Time String(want seconds? (F)=TRUE) -> (date string=w3542:string)  [unwired: 2 in, 1 out]
            n1239 = call <vilib>:"Open Config Data.vi"("create file if necessary (T)"=FALSE, "configuration file path"=w3506) -> ("refnum"=w3518:T12)  [unwired: 1 in, 8 out]
            n1240 = property on="POWER Board S/N" class="Str"() -> ("Value"=w3469:string)  [unwired: 2 in, 2 out]
            n1241 = property on="Logger Path" class="Path"(error in=w3543, "Value"=w3481, "StartPath"=w3481) -> (error out=w3521:errorcluster)  [unwired: 1 in, 1 out]
            n1242 = Search and Replace String(replace all?=TRUE ("replace all? (F)"), input string=w3542, search string="/") -> (result string=w3524:string)  [unwired: 5 in, 3 out]
            n1243 = call-poly <vilib>:"Read Key.vi"("section"=w3511, "key"=w3509, "refnum"=w3518) -> ("error out"=w3513:errorcluster, "value"=w3516:string, "refnum out"=w3515:T12)  [unwired: 5 in, 1 out]
            n1244 = property on="DSP Board S/N" class="Str"() -> ("Value"=w3468:string)  [unwired: 2 in, 2 out]
            n1245 = call-poly <vilib>:"Read Key.vi"("section"=w3511, "error in (no error)"=w3513, "key"="Tester Software Ver", "refnum"=w3515) -> ("error out"=w3510:errorcluster, "refnum out"=w3514:T12)  [unwired: 4 in, 2 out]
            n1246 = Concatenate Strings("ATR" ("string"), w3527, w3474, "_", w3524, ".docx" ("string")) -> (w3522:string)
            n1247 = call <vilib>:"Close Config Data.vi"("error in (no error)"=w3510, "refnum"=w3514) -> ()  [unwired: 8 in, 2 out]
            n1248 = Build Path(base path=w3481, name or relative path=w3522) -> (appended path=w3523:path)
            n1249 = Concatenate Strings("  Rev-" ("string"), w3516) -> (w3505:string)
            n1250 = while {
              tunnel: w3522 -> [w3587]
              tunnel: w3481 -> [w3584]
              shift-right: [w3586] -> w3520
              shift-left: w3523 -> [w3585]
              shift-right: [w3582] -> w3507
              shift-left: w3508 -> [w3583]
              tunnel: w3521 -> [w3588]
              tunnel: [w3589] -> w3480
              stop <- w3581 continue-if-true
              n1251 = call <vilib>:"Check if File or Folder Exists.vi"("error in (no error)"=w3588, "path"=w3585) -> ("error out"=w3589:errorcluster, "file or folder exists?"=w3581:bool)  [unwired: 7 in, 1 out]
              n1252 = case shown="True" w3581 {
                tunnel: w3587 -> [_ w3601]
                tunnel: w3583 -> [_ w3593]
                tunnel: [w3591 w3598] -> w3586
                tunnel: w3585 -> [w3591 _]
                tunnel: w3584 -> [_ w3599]
                tunnel: [1 w3592] -> w3582
                frame False {
                }
                frame True {
                  w3594 = ".docx" ("search string")
                  n1253 = Search and Replace String(input string=w3601, search string=w3594) -> (result string=w3600:string)  [unwired: 6 in, 3 out]
                  n1254 = Number To Decimal String(number=w3593) -> (decimal integer string=w3596:string)  [unwired: 1 in]
                  n1255 = call <vilib>:"Space Constant.vi"() -> ("String"=w3595:string)
                  n1256 = Concatenate Strings(w3600, w3595, w3596, w3594) -> (w3597:string)
                  n1257 = Build Path(base path=w3599, name or relative path=w3597) -> (appended path=w3598:path)
                  n1258 = Increment(x=w3593) -> (x+1=w3592:i32)
                }
              }
            }
            n1259 = call "HeaderBis.vi"("UUTHeader"=w3476, "UA"=w3473, "POWER SN"=w3469, "Revision Param"=w3471, "P/N UUT"=w3470, "DSP SN"=w3468, "Driver S/N"=w3474, "VR"=w3472, "Oper."=w3475, "Tester Software Ver"=w3464) -> ("table header"=w3467:string, "Array"=w3466:string[][])  [unwired: 3 in, 1 out]
            n1260 = Open/Create/Replace File(file path (use dialog)=w3520, error in=w3480, operation (0:open)=T25."create") -> (error out=w3533:errorcluster)  [unwired: 3 in, 2 out]
            n1261 = control-ref of="ATR"() -> (w3545:refnum<vi>)
            n1262 = property class="Tbl (strict)"(reference=w3545, error in=w3533) -> ("Value"=w3546:string[][])  [unwired: 2 out]
            n1263 = call "MarvinReport.vi"("HEADER1"=w3467, "ATR Or"=w3545, "Steps   pfull"=w3546, "Footer UUT"=w3497, "pageNum"=3, "InputHeaderArray"=w3466, "FILE NAME"=w3522, "Report Folder"=w3520, "REV"=w3505, "Test-Conductor"=w3475) -> ("error out"=w3492:errorcluster)  [unwired: 4 in, 1 out]
            n1264 = call <vilib>:"Clear Errors.vi"("error in (no error)"=w3492) -> ("error out"=w3491:errorcluster)  [unwired: 5 in, 1 out]
            n1265 = property class="Bool (strict)"(reference=w3503, error in=w3491) -> ("BoolText.Text"=w3502:string)  [unwired: 2 out]
            n1266 = Equal?(x=w3502, y="Report") -> (x = y?=w3496:bool)
            n1267 = Select(t=T11."MainProgram", s=w3496, f=T11."Stop") -> (s? t:f=w3499:T11)
            n1268 = Select(t="Save Report...", s=w3496, f="Program Stopped...\r\nPlease turn OFF All Power sinks") -> (s? t:f=w3494:string)
            n1269 = property on="Report" class="Bool (strict)"(error in=w3491, "Value"=FALSE ("Report")) -> (error out=w3485:errorcluster)  [unwired: 1 in, 1 out]
            n1270 = property on="VISA Tester" class="VISAName"() -> ("Value"=w3489:refnum<visa-resource-name>)  [unwired: 2 in, 2 out]
            n1271 = property on="Pannel User Message" class="Str"("Value"=w3494) -> ()  [unwired: 2 in, 2 out]
            n1272 = call "TesterOption (SubVI).vi"("2 Options"=FALSE, "error in (no error)"=w3485, "On/Off"=FALSE, "Tester Option"=T13."Venable", "VISA Refnum in"=w3489) -> ()  [unwired: 5 in, 2 out]
          }
          event "Help Button": Value Change {
            n1273 = event-data() -> ()  [unwired: 1 in, 6 out]
            n1274 = vi-ref "Help.vi"() -> (w3621:refnum<vi>)
            n1275 = invoke class="VI" method="FP.Open"(reference=w3621, error in=w3619, "Activate"=TRUE ("Activate?"), "State"=T23."Standard") -> (error out=w3620:errorcluster)  [unwired: 1 in, 4 out]
            n1276 = call "Help.vi"("error in"=w3620, "TesterSWVersion"=w3611) -> ("error out"=w3618:errorcluster)  [unwired: 6 in]
            n1277 = property on="Help Button" class="Bool (strict)"("Value"=FALSE ("Help Button")) -> ()  [unwired: 2 in, 2 out]
          }
          event "Serial Com": Value Change {
            n1278 = event-data() -> ()  [unwired: 1 in, 6 out]
            n1279 = property on="Serial Com" class="Bool"(error in=w3632, "Visible"=FALSE) -> (error out=w3636:errorcluster)  [unwired: 1 in, 1 out]
            n1280 = property on="VISA Marvin" class="VISAName"(error in=w3636, "Visible"=TRUE) -> (error out=w3633:errorcluster)  [unwired: 1 in, 1 out]
          }
          event "VISA Marvin": Value Change {
            n1281 = event-data() -> ()  [unwired: 1 in, 6 out]
            n1282 = property on="Serial Com" class="Bool"(error in=w3641, "Visible"=FALSE) -> (error out=w3640:errorcluster)  [unwired: 1 in, 1 out]
            n1283 = control-ref of="This VI"() -> (w3652:refnum<vi>)
            n1284 = property on="Pannel User Message" class="Str"(error in=w3641, "Value"="Serial connection in process" ("Pannel User Message")) -> ()  [unwired: 1 in, 2 out]
            n1285 = call "Serial InitMarvin.vi"("error in (no error)"=w3640, "VI reference (current VI)"=w3652, "VISA Refnum in"="VISA Marvin") -> ("error out"=w3644:errorcluster, "Boolean"=w3642:bool)  [unwired: 7 in]
            n1286 = property on="VISA Marvin" class="VISAName"(error in=w3644, "Visible"=FALSE) -> (error out=w3655:errorcluster)  [unwired: 1 in, 1 out]
            n1287 = property on="Serial Com" class="Bool"(error in=w3655, "Visible"=TRUE) -> (error out=w3651:errorcluster)  [unwired: 1 in, 1 out]
            n1288 = case shown="True" w3642 {
              tunnel: w3651 -> [w3658 w3671]
              tunnel: "VISA Marvin" -> [w3659 w3668]
              tunnel: [w3659 w3667] -> w3646
              tunnel: [w3658 w3666] -> w3645
              frame False {
              }
              frame True {
                n1289 = call "SerialMarvinSendGet.vi"("error in (no error)"=w3671, "Clear Log"=FALSE, "write buffer"="VC\r\n", "VISA resource name"=w3668) -> ("error out"=w3670:errorcluster, "read buffer"=w3664:string)  [unwired: 6 in]
                n1290 = Decimal String To Number(string=w3664) -> (number=w3663:i32)  [unwired: 2 in, 1 out]
                n1291 = property on="UUT" class="Str"() -> ("Value"=w3660:string)  [unwired: 2 in, 2 out]
                n1292 = Less Or Equal?(x=w3663, y=50) -> (x <= y?=w3661:bool)
                n1293 = property on="Status" class="Bool (strict)"("Value"=w3661) -> ()  [unwired: 2 in, 2 out]
                n1294 = case shown="True" w3661 {
                  tunnel: w3670 -> [w3672 w3704]
                  tunnel: w3668 -> [w3673 w3703]
                  tunnel: [w3673 w3677] -> w3667
                  tunnel: [w3672 w3680] -> w3666
                  tunnel: w3660 -> [_ w3674]
                  frame False {
                  }
                  frame True {
                    n1295 = call <vilib>:"Clear Errors.vi"("error in (no error)"=w3704) -> ("error out"=w3705:errorcluster)  [unwired: 5 in, 1 out]
                    n1296 = control-ref of="ATR"() -> (w3675:refnum<vi>)
                    n1297 = VISA Flush I/O Buffer(VISA resource name=w3703, error in (no error)=w3705) -> (VISA resource name out=w3677:refnum<visa-resource-name>, error out=w3702:errorcluster)  [unwired: 1 in]
                    n1298 = call "Display Message to User2"("error in (no error)"=w3702) -> ("error out"=w3701:errorcluster, "Yes"=w3700:bool)  [unwired: 9 in]
                    n1299 = case shown="True" w3700 {
                      tunnel: w3701 -> [w3731 w3753]
                      tunnel: [w3731 w3732] -> w3699
                      tunnel: w3677 -> [_ w3750]
                      frame False {
                      }
                      frame True {
                        w3738 = FALSE ("2 Options")
                        n1300 = property on="UUT" class="DigNum (strict)"() -> ("Value"=w3752:u8)  [unwired: 2 in, 2 out]
                        n1301 = call "SetParam.vi"("RS"=TRUE, "error in (no error)"=w3753, "Param to Set in"=w3752, "Visa"=w3750) -> ("error out"=w3733:errorcluster)  [unwired: 7 in]
                        n1302 = control-ref of="Pannel User Message"() -> (w3749:refnum<vi>)
                        n1303 = control-ref of="Stop Burn-in"() -> (w3747:refnum<vi>)
                        n1304 = control-ref of="Stop Button"() -> (w3748:refnum<vi>)
                        n1305 = control-ref of="Motor Speed RPM"() -> (w3746:refnum<vi>)
                        n1306 = property on="VISA Tester" class="VISAName"() -> ("Value"=w3742:refnum<visa-resource-name>)  [unwired: 2 in, 2 out]
                        n1307 = call "TesterOption (SubVI).vi"("2 Options"=w3738, "error in (no error)"=w3733, "On/Off"=FALSE, "Tester Option"=T13."Power", "VISA Refnum in"=w3742) -> ("error out"=w3743:errorcluster, "VISA Refnum out"=w3745:refnum<visa-resource-name>)  [unwired: 5 in]
                        n1308 = call "Write panel message (SubVI).vi"("Stop BurnIn"=w3747, "rpm"=w3746, "PrintTime"=TRUE, "Stop"=w3748, "error in (no error)"=w3743, "Time to wait"=20.0, "Strin"="Restart the UUT\nPlease wait...", "String in"=w3749) -> ("error out"=w3744:errorcluster)  [unwired: 3 in]
                        n1309 = call "TesterOption (SubVI).vi"("2 Options"=w3738, "error in (no error)"=w3744, "On/Off"=FALSE, "Tester Option"=T13."Venable", "VISA Refnum in"=w3745) -> ("error out"=w3732:errorcluster)  [unwired: 5 in, 1 out]
                      }
                    }
                    n1310 = call "SerialMarvinSendGet.vi"("error in (no error)"=w3699, "write buffer"="SN\r\n", "VISA resource name"=w3677) -> ("error out"=w3679:errorcluster, "read buffer"=w3687:string)  [unwired: 7 in]
                    n1311 = case shown="\"AHU\"" w3674 {
                      tunnel: w3679 -> [w3713 w3729]
                      tunnel: [w3711 w3729] -> w3678
                      tunnel: w3677 -> [w3710 _]
                      tunnel: [w3709 w3730] -> w3676
                      tunnel: w3675 -> [w3708 w3730]
                      frame "False", Default {
                        n1312 = property on="UUT SoftwareVer" class="Str"() -> ("Value"=w3717:string)  [unwired: 2 in, 2 out]
                        n1313 = call "SerialMarvinSendGet.vi"("error in (no error)"=w3713, "write buffer"="VR\r\n", "VISA resource name"=w3710) -> ("error out"=w3712:errorcluster, "read buffer"=w3716:string)  [unwired: 7 in]
                        n1314 = Equal?(x=w3716, y=w3717) -> (x = y?=w3715:bool)
                        n1315 = case shown="True" w3715 {
                          tunnel: w3712 -> [w3721 w3728]
                          tunnel: [w3721 w3727] -> w3711
                          tunnel: [w3720 w3726] -> w3709
                          tunnel: w3708 -> [w3720 w3725]
                          tunnel: [u16 14700 ("MaxEbaySpeed") u16 15100 ("MaxEbaySpeed")] -> w3707
                          tunnel: [TRUE ("5.4.0") FALSE ("5.4.0")] -> w3706
                          frame False {
                          }
                          frame True {
                            # "5.3.9"
                            n1316 = property class="Tbl (strict)"(reference=w3725, error in=w3728, "Value"=string[][] [["1", "Communication Test", "", "", "", "", ""], ["1.1", "Serial RS-232", "N/A", "-", "", "", ""], ["1.2", "CAN Bus", "N/A", "-", "", "", ""], ["", "", "", "", "", "", ""], ["2", "Auxiliary Fan Test", "", "", "", "", ""], ["2.1", "Auxiliary Cooling Fan ON", "60", "+/-2.00", "°C", "", ""], ["2.2", "Fan status", "ON", "-", "-", "", ""], ["2.3", "Fan status-OFF", "55", "+/-2.00", "°C", "", ""], ["2.4", "Fan status", "OFF", "-", "-", "", ""], ["", "", "", "", "", "", ""], ["3", "Temperature Sensor Calibration", "", "", "", "", ""], ["3.1", "Sensor Reading Analog Offset", "0", "+/-0.100", ".", "", ""], ["", "", "", "", "", "", ""], ["4", "Motor Termistor Input Test", "", "", "", "", ""], ["4.1", "60 Degree", "60", "+/-3.00", "°C", "", ""], ["4.2", "90 Degree", "90", "+/-3.00", "°C", "", ""], ["4.3", "120 Degree", "120", "+/-3.00", "°C", "", ""], ["", "", "", "", "", "", ""], ["5", "Enable Test", "", "", "", "", ""], ["5.1", "Fan Speed at Opened Enable ", "5000", "+/-200.0", "rpm", "", ""], ["5.2", "Fan Speed at Opened Enable ", "0", "+/-200.0", "rpm", "", ""], ["5.3", "Fan Speed at Closed Enable ", "5000", "+/-200.0", "rpm", "", ""], ["5.4", "Motor Rotation Direction", "CCW", "-", "", "", ""], ["", "", "", "", "", "", ""], ["6", "Speed Command Test", "", "", "", "", ""], ["6.1", "Fan  Speed", "6000", "+/-200.0", "rpm", "", ""], ["6.2", "Fan  Speed", "11500", "+/-200.0", "rpm", "", ""], ["6.3", "Fan  Speed", "15100", "+/-200.0", "rpm", "", ""], ["", "", "", "", "", "", ""], ["7", "Motor Stop time", "< 50", "-", "sec", "", ""], ["", "", "", "", "", "", ""], ["8", "Temperature Control Algorithm Test", "", "", "", "", ""], ["8.1", "Tair <   68 ± 2 °C", "6000", "+/-200.0", "rpm", "", ""], ["8.2", "Measured Temp.", "", "", "°C", "", ""], ["8.3", "Tair >= 68 ± 2 °C", "11500", "+/-200.0", "rpm", "", ""], ["8.4", "Transition Temp.", "", "", "°C", "", ""], ["8.5", "Tair >= 88 ± 2 °C", "15100", "+/-400.0", "rpm", "", ""], ["8.6", "Transition Temp.", "", "", "°C", "", ""], ["8.7", "Tair <= 80 ± 2 °C", "11500", "+/-200.0", "rpm", "", ""], ["8.8", "Transition Temp.", "", "", "°C", "", ""], ["8.9", "Tair <= 60 ± 2 °C", "6000", "+/-200.0", "rpm", "", ""], ["8.10", "Transition Temp.", "", "", "°C", "", ""], ["", "", "", "", "", "", ""], ["9", "Burn-in Test", "", "", "", "", ""], ["9.1", "DC Input Current", "50", "+/-5.000", "A", "", ""], ["9.2", "Fan speed", "15100", "+/-200.0", "rpm", "", ""], ["9.3", "Ambient Temperature", "25", "+/-13.00", "°C", "", ""], ["9.4", "After 10 min of operation", "", "-", "°C", "", ""], ["9.5", "After 20 min of operation", "", "-", "°C", "", ""], ["9.6", "After 30 min of operation", "", "-", "°C", "", ""], ["", "", "", "", "", "", ""], ["10", "Visual Inspection", "", "", "", "", ""], ["10.1", "Verification of Components Not Installed", "N/A", "-", "", "", ""], ["10.2", "Manufacturing Defects", "N/A", "-", "", "", ""], ["", "", "", "", "", "", ""], ["11", "Power Supply Testing", "", "", "", "", ""], ["11.1", "DC Input Current Drawn", "150", "+/-10.00", "mA", "", ""], ["", "", "", "", "", "", ""], ["12", "Power Supply Voltages", "", "", "", "", ""], ["12.1", "12V", "12.0", "+/-0.500", "V", "", ""], ["12.2", "5V", "5.0", "+/-0.200", "V", "", ""], ["12.3", "3.3V", "3.3", "+/-0.100", "V", "", ""], ["12.4", "1.8V", "1.8", "+/-0.100", "V", "", ""], ["", "", "", "", "", "", ""], ["13", "Reverse Polarity Test - DC Input Current", "< 1", "-", "mA", "", ""], ["", "", "", "", "", "", ""], ["14", "Functional Test Procedure", "", "", "", "", ""], ["14.1", "Weight Check", "4180", "+/-100.0", "gr", "", ""], ["", "", "", "", "", "", ""], ["15", "Insulation Resistance Test", "", "", "", "", ""], ["15.1", "J3.B to Chassis", "> 1M", "-", "ohms", "", ""], ["15.2", "J1.16 to Chassis", "> 100K", "-", "ohms", "", ""], ["", "", "", "", "", "", ""], ["16", "Bonding Resistance", "", "", "", "", ""], ["16.1", "J1 Body to Chassis", "< 2m", "-", "ohms", "", ""], ["16.2", "J2  Body to Chassis", "< 2m", "-", "ohms", "", ""], ["16.3", "J3  Body to Chassis", "< 2m", "-", "ohms", "", ""], ["", "", "", "", "", "", ""], ["17", "CANbus Resistance Test", "", "", "", "", ""], ["17.1", "J1.17 to J1.18", "> 10K", "-", "ohms", "", ""], ["", "", "", "", "", "", ""], ["18", "Sealing Test", "N/A", "-", "", "", ""], ["", "", "", "", "", "", ""], ["19", "Mounting Holes Test - Jig Fit", "214", "-", "mm", "", ""]] ("ArrEbay 3")) -> (reference out=w3726:refnum<vi>, error out=w3727:errorcluster)
                          }
                        }
                        "5.4.0" <- w3706
                        n1317 = property on="MaxEbaySpeed" class="DigNum (strict)"("Value"=w3707) -> ()  [unwired: 2 in, 2 out]
                      }
                      frame "AHU" {
                      }
                    }
                    n1318 = call "SerialMarvinSendGet.vi"("error in (no error)"=w3678, "write buffer"="AO[1]\r\n", "VISA resource name"=w3677) -> ("error out"=w3692:errorcluster, "read buffer"=w3693:string)  [unwired: 7 in]
                    n1319 = Fract/Exp String To Number(string=w3693) -> (number=w3689:dbl)  [unwired: 3 in, 1 out]
                    n1320 = In Range and Coerce(upper limit=0.1 ("x"), x=w3689, lower limit=-0.1) -> (In Range?=w3688:bool)  [unwired: 1 out]
                    n1321 = call "Find_Number_LineMARVIN.vi"("Test Paragraph"="Sensor Reading Analog Offset", "TableIn"=w3676) -> ("Line number"=w3694:i32)  [unwired: 3 in, 3 out]
                    n1322 = call "PassOrFail (SubVI).vi"("Test#"="2", "index (row)"=w3694, "error in (no error)"=w3692, "Data in"=w3689, "Pass?Fail"=w3688, "Table in"=w3676) -> ("error out"=w3681:errorcluster)  [unwired: 5 in]
                    n1323 = property on="VISA Marvin" class="VISAName"(error in=w3681) -> (error out=w3684:errorcluster, "Value"=w3685:refnum<visa-resource-name>)  [unwired: 1 in, 1 out]
                    n1324 = property on="UUT SN Report" class="Str"("Value"=w3687) -> ()  [unwired: 2 in, 2 out]
                    n1325 = call "SerialMarvinSendGet.vi"("error in (no error)"=w3684, "Clear Log"=FALSE, "write buffer"="EP=1\r\nMD[1]=1\r\n", "VISA resource name"=w3685) -> ("error out"=w3680:errorcluster)  [unwired: 6 in, 1 out]
                    n1326 = Decimal String To Number(string=w3687) -> (number=→"Current SN":i32)  [unwired: 2 in, 1 out]
                  }
                }
              }
            }
          }
          event "Refresh Button": Value Change {
            n1327 = event-data() -> ()  [unwired: 1 in, 6 out]
          }
          event "Settings": Value Change {
            n1328 = event-data() -> ()  [unwired: 1 in, 6 out]
            n1329 = control-ref of="VISA Tester"() -> (w3767:refnum<vi>)
            n1330 = control-ref of="UUT"() -> (w3765:refnum<vi>)
            n1331 = property on="Status" class="Bool (strict)"() -> ("Value"=w3769:bool)  [unwired: 2 in, 2 out]
            n1332 = case shown="True" w3769 {
              tunnel: w3775 -> [_ w3787]
              tunnel: [w3776 w3782] -> w3770
              tunnel: w3768 -> [_ w3781]
              tunnel: w3767 -> [_ w3780]
              tunnel: w3766 -> [_ w3779]
              tunnel: w3765 -> [_ w3778]
              frame False {
                n1333 = call "Display Message to User8"() -> ("error out"=w3776:errorcluster)  [unwired: 10 in, 1 out]
              }
              frame True {
                n1334 = vi-ref "Calibration (SubVI).vi"() -> (w3786:refnum<vi>)
                n1335 = invoke class="VI" method="FP.Open"(reference=w3786, error in=w3787, "Activate"=TRUE ("Activate?"), "State"=T23."Standard") -> (error out=w3783:errorcluster)  [unwired: 1 in, 4 out]
                n1336 = call "Calibration (SubVI).vi"("VISA UUT"=w3781, "error constant"=w3783, "UUT"=w3778, "CAN Cluster in"=w3779, "Visa Tester"=w3780) -> ("error constant 2"=w3782:errorcluster, "AO[1]Meas"=→"Cal":dbl)  [unwired: 5 in]
              }
            }
          }
        }
      }
      frame "Initialize" {
        w3789 = 0
        w3794 = FALSE ("Visible")
        w3795 = FALSE ("Visible")
        w3796 = FALSE ("Visible")
        w3797 = FALSE ("Visible")
        w3808 = refnum<visa-resource-name> "COM1" ("VISA resource name")
        w3799 = FALSE ("Visible")
        w3792 = FALSE ("Serial Status")
        n1337 = property on="ComTestResult" class="Bool (strict)"("Value"=w3797) -> ()  [unwired: 2 in, 2 out]
        n1338 = property on="VenableResult" class="Bool (strict)"("Value"=w3797) -> ()  [unwired: 2 in, 2 out]
        n1339 = property on="VenableDirectionResult" class="Bool (strict)"("Value"=w3797) -> ()  [unwired: 2 in, 2 out]
        n1340 = property on="SpeedResult" class="Bool (strict)"("Value"=w3797) -> ()  [unwired: 2 in, 2 out]
        n1341 = property on="Serial Com" class="Bool"(error in=errorcluster {"status"=FALSE, "code"=0, "source"=""} ("error out"), "Visible"=TRUE) -> (error out=w3810:errorcluster)  [unwired: 1 in, 1 out]
        n1342 = property on="AuxiOFFResult" class="Bool (strict)"("Value"=w3796) -> ()  [unwired: 2 in, 2 out]
        n1343 = property on="AuxiONResult" class="Bool (strict)"("Value"=w3796) -> ()  [unwired: 2 in, 2 out]
        n1344 = property on="VisualInspectionResult" class="Bool (strict)"("Value"=w3796) -> ()  [unwired: 2 in, 2 out]
        n1345 = property on="SensCalResult" class="Bool (strict)"("Value"=w3796) -> ()  [unwired: 2 in, 2 out]
        n1346 = property on="VISA Marvin" class="VISAName"(error in=w3810, "Visible"=w3799, "Value"=w3808) -> (error out=w3800:errorcluster)  [unwired: 1 in, 1 out]
        n1347 = property on="Stop Burn-in" class="Bool (strict)"(error in=w3800, "Visible"=w3799) -> (error out=w3793:errorcluster)  [unwired: 1 in, 1 out]
        n1348 = property on="BurnDC" class="Bool (strict)"("Value"=w3795) -> ()  [unwired: 2 in, 2 out]
        n1349 = property on="BurnTemp" class="Bool (strict)"("Value"=w3795) -> ()  [unwired: 2 in, 2 out]
        n1350 = property on="BurnSpeed" class="Bool (strict)"("Value"=w3795) -> ()  [unwired: 2 in, 2 out]
        n1351 = property on="BurnResult" class="Bool (strict)"("Value"=w3795) -> ()  [unwired: 2 in, 2 out]
        n1352 = property on="Refresh Button" class="Bool (strict)"(error in=w3793, "Value"=FALSE ("Refresh Button")) -> ()  [unwired: 1 in, 2 out]
        n1353 = property on="StopTimeResult" class="Bool (strict)"("Value"=w3794) -> ()  [unwired: 2 in, 2 out]
        n1354 = property on="MotorTempResult" class="Bool (strict)"("Value"=w3794) -> ()  [unwired: 2 in, 2 out]
        n1355 = property on="TempControlResult" class="Bool (strict)"("Value"=w3794) -> ()  [unwired: 2 in, 2 out]
        n1356 = property on="Automation" class="Bool (strict)"("Value"=w3794) -> ()  [unwired: 2 in, 2 out]
        n1357 = flat-sequence {
          tunnel: w3793 -> [w3812]
          tunnel: [w3812] -> w3790
          tunnel: [w3814] -> w3806
          tunnel: w3790 -> [w3814]
          tunnel: [w3826] -> w3805
          tunnel: w3806 -> [w3827]
          tunnel: [w3827] -> w3804
          frame #0 {
          }
          frame #1 {
            w3817 = u32 4294967295  # AccMask
            w3813 = T5 0 items=["使用Flash参数", "使用界面设置参数"] ("InitFlag")
            w3815 = T7 0 items=["normal operation", "Listen-only mode", "test mode"]  # Mode
            w3816 = T6 3 items=["接收所有类型"=1, "只接收标准帧"=2, "只接收扩展帧"=3] ("Fliter")
            w3821 = u8 10 items=["5k bps"=1, "10k bps"=2, "20k bps"=3, "40k bps"=4, "50k bps"=5, "80k bps"=6, "100k bps"=7, "125k bps"=8, "200k bps"=9, "250k bps"=10, "400k bps"=11, "500k bps"=12, "666k bps"=13, "800k bps"=14, "1000k bps"=15, "33.33k bps"=16, "66.66k bps"=17, "83.33k bps"=18]  # kBaudRate
            w3818 = u32 0  # AccCode
            w3819 = T3 4 items=["USB-CAN"=3, "USB-CAN2"=4] ("DevType")
            w3820 = T8 {"DevType"=3, "DevIndex"=0, "CanIndex"=0, "VCI_INIT_CONFIG"={"AccCode"=0, "AccMask"=0, "InitFlag"=1, "Fliter"=7, "Timing0"=0, "Timing1"=0, "Mode"=0}}  # Config
            # "CANalystII"
            n1358 = call "Demo_GetT0T1.vi"("kBaudRate"=w3821) -> ("Timing0"=w3823:u8, "Timing1"=w3824:u8)
            n1359 = Bundle By Name(cluster=w3820, "DevType"=w3819, "CanIndex"="Channel 2", "VCI_INIT_CONFIG.AccCode"=w3818, "VCI_INIT_CONFIG.AccMask"=w3817, "VCI_INIT_CONFIG.InitFlag"=w3813, "VCI_INIT_CONFIG.Fliter"=w3816, "VCI_INIT_CONFIG.Timing0"=w3823, "VCI_INIT_CONFIG.Timing1"=w3824, "VCI_INIT_CONFIG.Mode"=w3815) -> (→"Config_CANAT":T8)
          }
          frame #2 {
            w3828 = u16 284 items=["1M"=20, "500K"=28, "250K"=284, "125K"=796, "100K"=17199, "50K"=18223, "20K"=21295, "10K"=26415, "5K"=32639] ("baud in")
            n1360 = control-ref of="Config_CANAT"() -> (w3826:refnum<vi>)
            n1361 = call "InitCAN_ATII.vi"("Config"=w3826) -> ("Sts"=→"CAN Status":bool)
            n1362 = call "ChangeCANBaud.vi"("baud in"=w3828, "reference"=w3826) -> ()
          }
        }
        n1363 = property on="5.4.0" class="Bool (strict)"("Value"=FALSE ("5.4.0")) -> ()  [unwired: 2 in, 2 out]
        "Status" <- w3792
        "Test Failed" <- w3792
      }
    }
  }
  n1364 = property on="Settings" class="Bool (strict)"("Visible"=w20) -> ()  [unwired: 2 in, 2 out]
  n1365 = property on="Cal" class="DigNum (strict)"("Visible"=w20) -> ()  [unwired: 2 in, 2 out]
  n1366 = disable-structure shown="Disabled" {
    frame Disabled {
      w3830 = T21."Disabled and Grayed Out" ("Disabled")
      w3831 = FALSE ("Start")
      n1367 = property on="VISA Tester" class="VISAName" props=["Value"]() -> ()  [unwired: 2 in, 3 out]
      n1368 = property on="Current SN" class="DigNum (strict)" props=["Value"]() -> ()  [unwired: 2 in, 3 out]
      n1369 = property on="UUT" class="DigNum (strict)" props=["Value"]() -> ()  [unwired: 2 in, 3 out]
      n1370 = property on="Status" class="Bool (strict)" props=["Value"]() -> ()  [unwired: 2 in, 3 out]
      n1371 = property on="UUT SoftwareVer" class="Str" props=["Value"]() -> ()  [unwired: 2 in, 3 out]
      n1372 = property on="Next SN" class="DigNum (strict)" props=["Value"]() -> ()  [unwired: 3 in, 2 out]
      n1373 = property on="Start" class="Bool (strict)"("Value"=w3831, "DisabledEnum"=w3830) -> ()  [unwired: 2 in, 2 out]
      n1374 = property on="Report" class="Bool (strict)"("Value"=w3831, "DisabledEnum"=w3830) -> ()  [unwired: 2 in, 2 out]
    }
    frame Enabled {
    }
  }
  n1375 = disable-structure shown="Disabled" {
    frame Disabled {
      (unwired) 0.02003173828125 ("x")
      n1376 = control-ref of="Stop Burn-in"() -> ()  [unwired: 1 out]
      n1377 = control-ref of="Stop Button"() -> ()  [unwired: 1 out]
      n1378 = control-ref of="Motor Speed RPM"() -> ()  [unwired: 1 out]
      n1379 = control-ref of="Config_CANAT"() -> ()  [unwired: 1 out]
      n1380 = control-ref of="UUT"() -> ()  [unwired: 1 out]
      n1381 = call "GetADCTester (SubVI).vi"() -> ()  [unwired: 9 in, 3 out]
      n1382 = call "CANSendMotorSpeed.vi"() -> ()  [unwired: 11 in, 1 out]
      n1383 = control-ref of="Config_CANAT"() -> ()  [unwired: 1 out]
      n1384 = call "Find_Number_LineMARVIN.vi"() -> ()  [unwired: 5 in, 4 out]
      n1385 = property on="UUT" class="DigNum (strict)" props=["Value"]() -> ()  [unwired: 2 in, 3 out]
      n1386 = control-ref of="UUT"() -> ()  [unwired: 1 out]
      n1387 = call "DegToDAC (SubVI).vi"() -> ()  [unwired: 10 in, 2 out]
      n1388 = call "Write panel message (SubVI).vi"() -> ()  [unwired: 11 in, 1 out]
      n1389 = property on="VISA Tester" class="VISAName" props=["Value"]() -> ()  [unwired: 2 in, 3 out]
      n1390 = control-ref of="ATR"() -> ()  [unwired: 1 out]
      n1391 = call "TesterOption (SubVI).vi"() -> ()  [unwired: 10 in, 2 out]
      n1392 = call "TesterOption (SubVI).vi"() -> ()  [unwired: 10 in, 2 out]
      n1393 = call "PassOrFail (SubVI).vi"() -> ()  [unwired: 11 in, 1 out]
    }
    frame Enabled {
    }
  }
  n1394 = disable-structure shown="Disabled" {
    frame Disabled {
      n1395 = flat-sequence {
        frame #0 {
          n1396 = call "CANSendMotorSpeed.vi"("Remote"=TRUE, "Motor Speed RPM"=u16 0) -> ("error out"=w3833:errorcluster, "UUT"=w3836:refnum<vi>)  [unwired: 8 in]
          n1397 = property on="VISA Tester" class="VISAName"() -> ("Value"=w3832:refnum<visa-resource-name>)  [unwired: 2 in, 2 out]
          n1398 = call "TesterOption (SubVI).vi"("error in (no error)"=w3833, "On/Off"=FALSE, "Tester Option"=T13."Power", "VISA Refnum in"=w3832) -> ()  [unwired: 6 in, 2 out]
        }
      }
    }
    frame Enabled {
    }
  }
  "Pannel User Message" <- w19
  "TesterVersion" <- w1
